vi "CellBild-v6.2.vi"() -> ()   [LabVIEW 2014]
uses:
  <vilib>/Utility/error.llb/DialogType.ctl
  <vilib>/DAQmx/create/channels.llb/DAQmx Create Channel (DI-Digital Input).vi
  <vilib>/DAQmx/create/channels.llb/DAQmx Create Channel (CO-Pulse Generation-Frequency).vi
  <vilib>/DAQmx/configure/timing.llb/DAQmx Timing (Implicit).vi
  <vilib>/DAQmx/create/channels.llb/DAQmx Create Channel (DO-Digital Output).vi
  <vilib>/DAQmx/write.llb/DAQmx Write (Digital Bool 1Line 1Point).vi
  <vilib>/DAQmx/write.llb/DAQmx Write (Analog DBL 1Chan 1Samp).vi
  <resource>/objmgr/daqmx.rc
panel:
  out "Pump running":bool
  out "dV":dbl format="%#.4g"
  out "Closing":bool
  out "In Done\nstate":bool
  in  "Tab Control":T1(tab)
  out "Shots to acquire":i32
  out "Shot no.":i32
  in  "Pump start":bool
  in  "Pulsed":bool
  in  "Populate":bool
  out "Full Power \nFrames":i32
  in  "Low Power\nFrames":i32
  in  "Link shutters":bool
  in  "FRAP":bool
  in  "EPI":bool
  in  "HALF DC":bool caption="Power"
  in  "manual laser control":bool
  in  "Continous ill":bool
  in  "Link rates":bool=TRUE
  in  "ALL OFF":bool
  in  "561 nm":bool
  in  "473 nm":bool
  in  "ALL LASERS":bool
  in  "Duty Cycle 1":dbl(knob)=0.47 caption="Duty Cycle\nlaser on state" min=0.001 max=0.999 step=0.05 scale=0.1..0.5
  in  "Frequency 1":dbl(knob)=100.0 caption="Laser\nrepetition rate" min=0.001 max=40000000.0 step=1.0 scale=1.0..500.0
  in  "stop":bool
  in  "Illuminated Frames":i32=10 min=0
  in  "Frame rate":dbl(knob)=200.0 min=0.01 max=40000000.0 step=1.0 scale=1.0..500.0
  in  "First frame\ndelay (ms)":dbl=15.0 min=50.0 format="%#_13g"
  in  "Finishing frames":i32=8
  out "Initial delay\n473 nm (ms)":dbl
  out "Trigger pulses":i32
  out "Initial frames":i32=2
  out "Laser pulses":i32
  out "Initial calculated\ndelay (frames)":dbl
  out "Laser delay (ms)":dbl
  out "Frames to acquire":i32
  in  "Duty Cycle \nDenominator":dbl=10.0 caption="Power\nDenominator" min=1.0 step=1.0
  out "AFLEX warning":bool caption="AFLEX conditions\nnormal"
  out "Duty Cycle 1\nfull DC":dbl(knob)=0.45 caption="Duty Cycle\nlaser on state" min=0.001 max=0.999 step=0.05 scale=0.1..0.5
  out "AFLEX warning 2":bool caption="AFLEX conditions\nnormal"
  out "Frame Rate display":dbl=2000.0 caption="Frame rate" min=0.0
  in  "Link shutters 2":bool caption="Link shutters"
  in  "FRAP 2":bool
  in  "EPI 2":bool
  out "initial delay\n473 nm (ms) 2":dbl caption="initial delay\n473 nm (ms)"
  in  "Link rates 2":bool=TRUE caption="Link rates"
  in  "Duty Cycle 2":dbl(knob)=0.47 caption="Duty Cycle\nlaser on state" min=0.001 max=0.999 step=0.05 scale=0.1..0.5
  in  "Frequency 2":dbl(knob)=100.0 caption="Laser\nrepetition rate" min=0.001 max=40000000.0 step=1.0 scale=1.0..500.0
  in  "Duty Cycle camera 2":dbl(knob)=0.001 caption="Duty Cycle\ncamera trigger" min=0.001 max=0.999 step=0.001 scale=0.001..0.999
  in  "Frame rate 2":dbl(knob)=200.0 caption="Frame rate" min=0.01 max=40000000.0 step=1.0 scale=1.0..500.0
  in  "AFLEX":bool
  in  "ALL OFF 2":bool
  in  "561 nm 2":bool
  in  "473 nm 2":bool
  in  "ALL LASERS 2":bool caption="ALL LASERS"
  in  "HALF DC 2":bool caption="Power"
  in  "Duty Cycle \nDenominator 2":dbl=2.0 caption="Power \nDenominator" min=1.0 step=1.0
  in  "Link shutters 3":bool
  in  "FRAP 3":bool
  in  "EPI 3":bool
  in  "FlowRateUnit":u32(ring) items=["ml/min", "ml/hr", "ul/min", "ul/hr"]
  in  "Flow rate":dbl=10.0
  in  "Syringe size":dbl(ring)=4.7 items=["1 ml"=4.7, "2.5 ml"=9.0, "3 ml"=8.59, "5 ml"=11.99, "10 ml"=14.48, "20 ml"=19.05, "30 ml"=21.59, "60 ml"=26.6]
  in  "Shots after pump start":i32=4
  in  "Deliverable volume (ml)":dbl min=0.0 step=0.1 format="%.4g"
  in  "Running time (s)":dbl=452.0
  in  "Shots before pump start":i32=1
  in  "Enable pump control":bool
  in  "Manual pump ctrl":bool
  in  "Pump initialisation":bool=TRUE
  in  "Pump ID":i32=3
  in  "Pump control port":refnum<visa-resource-name>="COM7"
  in  "Power control":bool=TRUE
  in  "idle state, shutdown":i32(ring)=10214 items=["High"=10192, "Low"=10214]
  in  "error in":errorcluster
  out "error out":errorcluster
  in  "561 nm counter":tag="Dev1/ctr4"
  in  "trigger ready source":tag="/Dev1/PFI3"
  in  "Camera trigger":tag="Dev1/ctr0"
  in  "473 nm counter":tag="Dev1/ctr2"
  in  "idle state, camera trig":i32(ring)=10214 items=["High"=10192, "Low"=10214]
  in  "idle state, lasers":i32(ring)=10214 items=["High"=10192, "Low"=10214]
  out "Loops":i32
  in  "Duty Cycle camera":dbl(knob)=0.0001 caption="Duty Cycle\ncamera trigger" min=0.0001 max=0.9999 step=5e-05 scale=0.0001..0.9999
  out "Duty Cycle 1\npreset":dbl(knob)=0.45 caption="Duty Cycle\nlaser on state" min=0.001 max=0.999 step=0.05 scale=0.1..0.999
  out "laser delay (s)":dbl
  in  "EPI ctrl":tag="Dev1/port0/line0"
  in  "FRAP ctrl":tag="Dev1/port0/line16"
  out "Duty Cycle 2\nmemory":dbl(knob)=0.45 caption="Duty Cycle\nlaser on state" min=0.001 max=0.999 step=0.05 scale=0.1..0.999
  in  "561nm line":tag="Dev2/ao0"
  in  "473nm line":tag="Dev2/ao1"
  in  "Level at max 473nm (0-5V)":dbl=4.200000000000002 caption="Level at max (0-5V)" min=0.0 max=5.0 step=0.05 format="%_4g"
  in  "473nm power level (0-1)":dbl=1.0 caption="Initial power level (0-1)" min=0.0 max=1.0 format="%_3g"
  in  "Level at max 561nm (0-5V)":dbl=4.225 caption="Level at max (0-5V)" min=0.0 max=5.0 step=0.05 format="%_4g"
  in  "561nm power level (0-1)":dbl=1.0 caption="Initial power level (0-1)" min=0.0 max=1.0 format="%_3g"
  out "561 task":refnum<k21>
  out "473 task":refnum<k21>
  out "HALF DC TEXT":string
  in  "delay\ncompensation":dbl format="%#_13g"
  out "Inited pump port":refnum<visa-resource-name>
  in  "vi path":path=path "C:/Biology/CellBild/Microfluidics/SPM100 control no loop v3.3.vi"
  out "modal pump reference":refnum<vi>
  # "Total number of frames to be\nilluminated (both channels)"
  # "Maximum number of frames\nthat can be acquired"
  # "Diagnostics"
  # "Laser Controls"
  # "Frame rate control"
  # "Shutter Controls"
  # "This tab generates a continous sequence of camera trigger pulses.\nLasers are synchronised with trigger pulse train but not synchronised with Micro-Manager acquisition start."
  # "Laser Controls"
  # "Shutter Controls"
  # "Frame rate control"
  # "Sequence settings"
  # "Pump settings"
  # "Enable pump sequence"
  # "Needed for \nmulti-shot \nacquisitions"
  # "IMPORTANT\nSafety for pump"
  # "Manual pump control"
  # "Total time \nfor all shots"
  # "Initial settings\nDAQ terminals"
  # "Pump control"
  # "Laser control counters"
  # "Laser power control settings"
  # "Camera trigger"
  # "Shutter control lines"
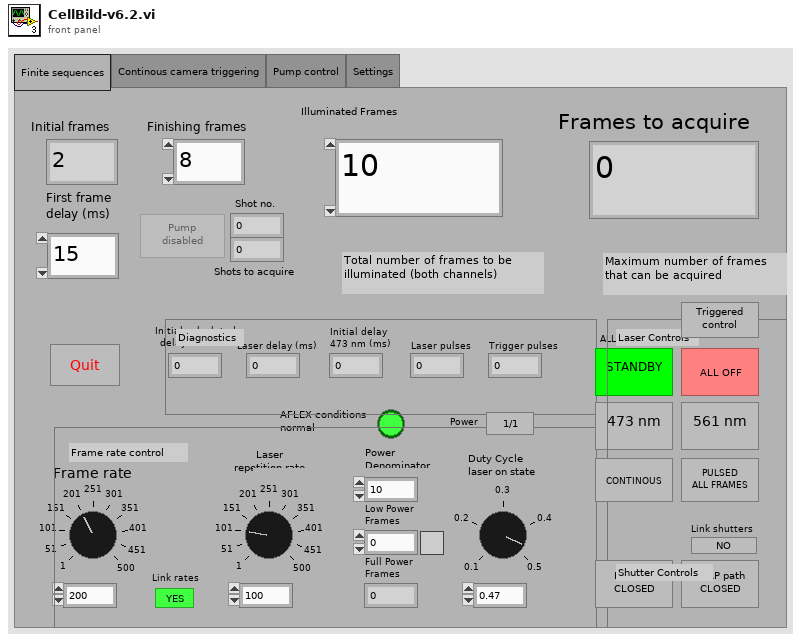
[diagram p1: front panel]
types:
  T1 = enum32{"Finite sequences", "Continous camera triggering", "Pump control", "Settings"}
  T2 = enum8{"Enabled", "Disabled", "Disabled and Grayed Out"}
  T3 = typedef "DialogType.ctl" = u16
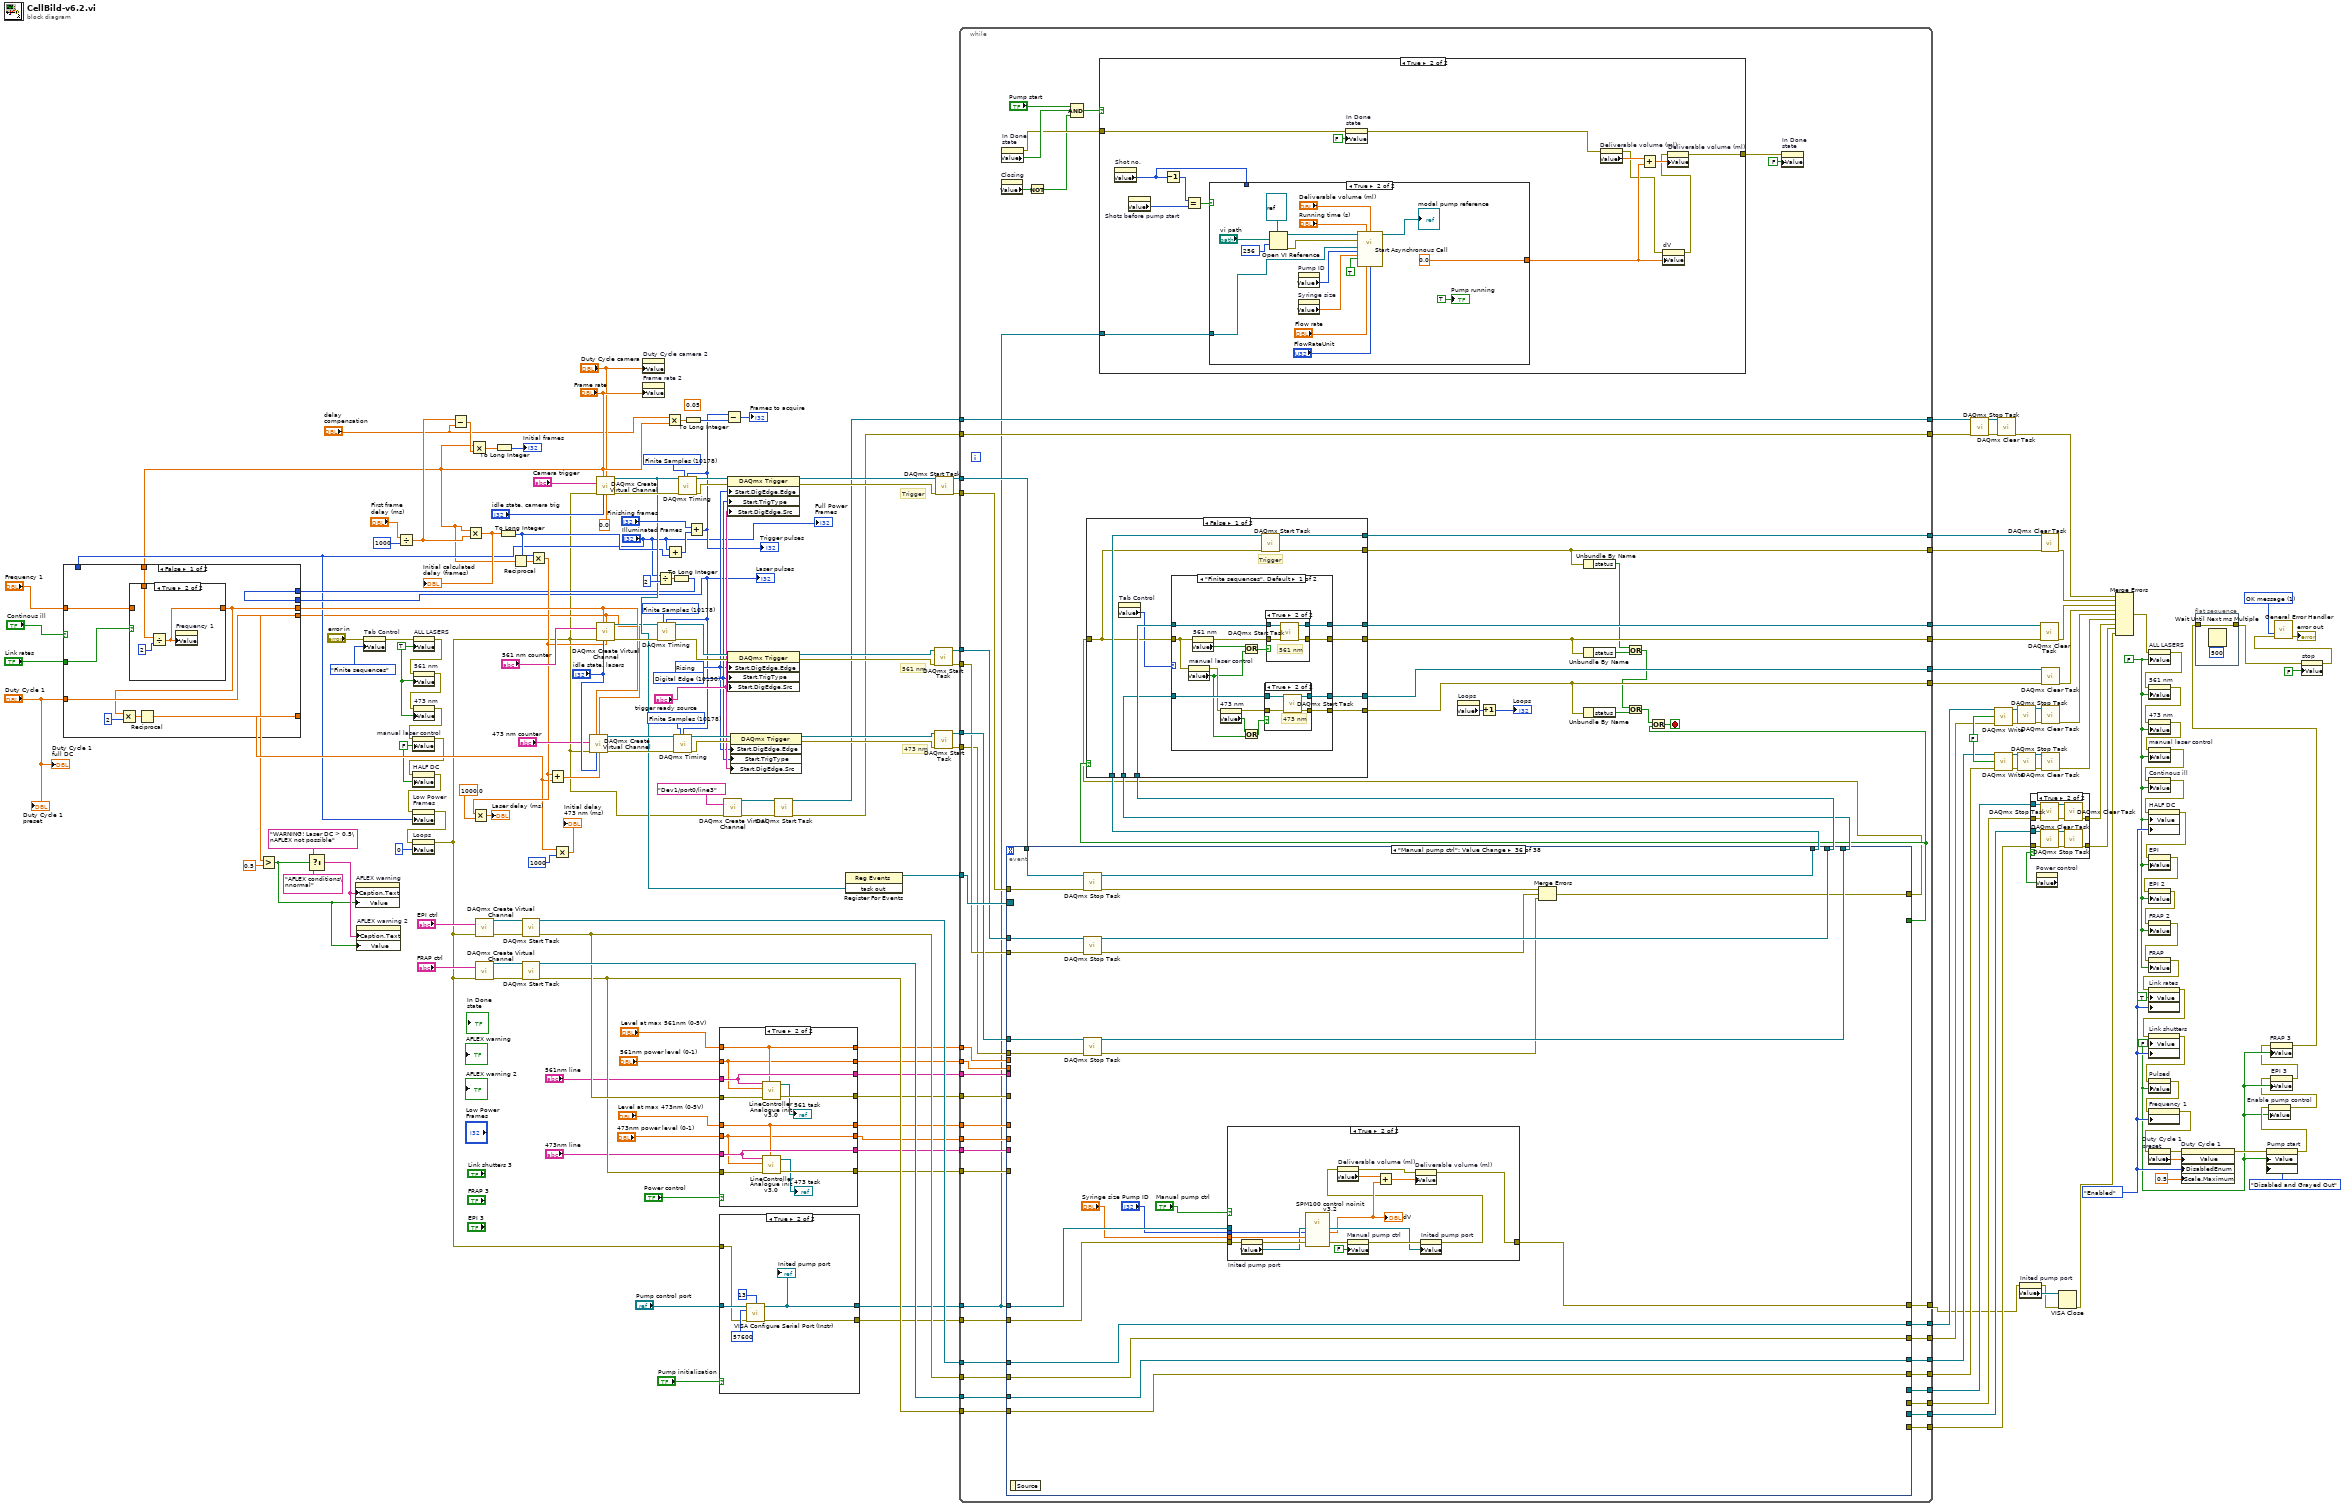
[diagram p0: block diagram]
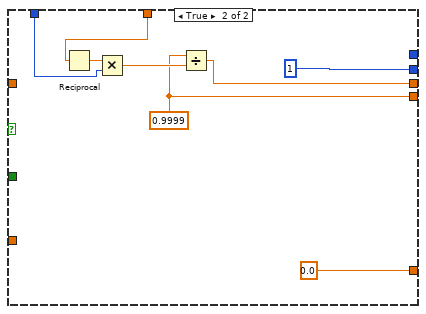
[diagram p6: hidden frame]
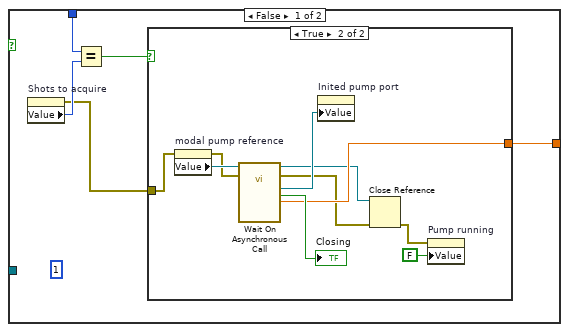
[diagram p8: hidden frame]
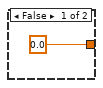
[diagram p9: hidden frame]
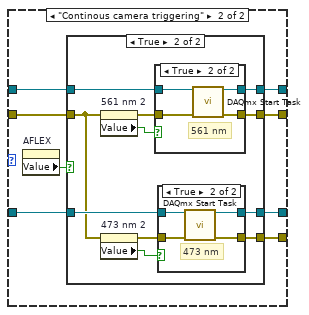
[diagram p12: hidden frame]
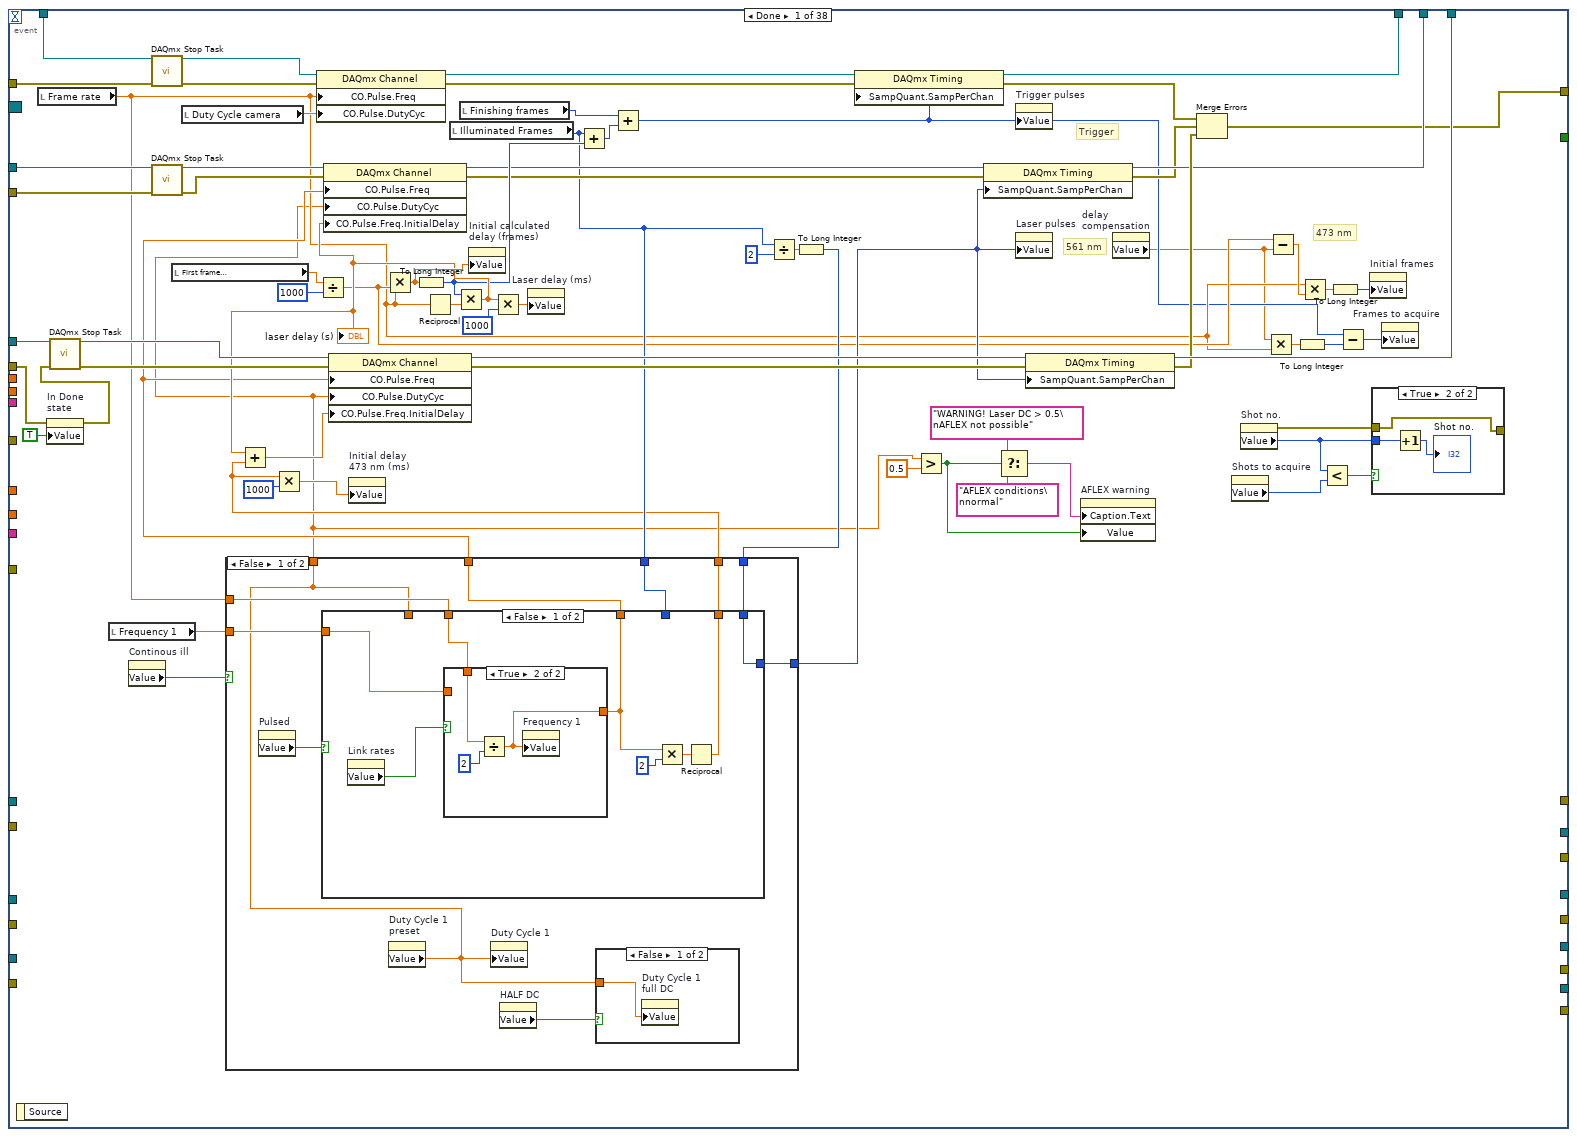
[diagram p17: hidden frame]
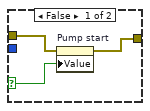
[diagram p18: hidden frame]
diagram:
  w74 = T2."Enabled" ("Disabled")
  (unwired) 0.05 ("x")
  w7 = FALSE ("Link shutters")
  w100 = FALSE ("data")
  w84 = FALSE ("manual laser control")
  w126 = TRUE ("Lasers on")
  w45 = FALSE ("Lasers on")
  w167 = 10178 items=["Finite Samples"=10178, "Continuous Samples"=10123, "Hardware Timed Single Point"=12522] ("sample mode")
  w185 = 10178 items=["Finite Samples"=10178, "Continuous Samples"=10123, "Hardware Timed Single Point"=12522] ("sample mode")
  w162 = 10150 items=["Analog Edge"=10099, "Digital Edge"=10150, "Digital Pattern"=10398, "Analog Window"=10103, "None"=10230] ("Start.TrigType")
  w161 = 10280 items=["Rising"=10280, "Falling"=10171] ("Start.DigEdge.Edge")
  w195 = T3 1 items=["no dialog", "OK message", "continue or stop message", "OK message + warnings", "continue/stop + warnings"] ("type of dialog (OK msg:1)")
  w197 = 10178 items=["Finite Samples"=10178, "Continuous Samples"=10123, "Hardware Timed Single Point"=12522] ("sample mode")
  # "Trigger"
  # "473 nm"
  # "561 nm"
  n1 = property on="Tab Control" class="TabCtl (strict)"(error in="error in", "Value"=T1."Finite sequences" ("Tab Control")) -> (error out=w125:errorcluster)  [unwired: 1 in, 1 out]
  n2 = Divide(x="First frame\ndelay (ms)", y=1000) -> (x/y=w92:dbl)
  n3 = property on="ALL LASERS" class="Bool (strict)"(error in=w125, "Value"=w126) -> (error out=w128:errorcluster)  [unwired: 1 in, 1 out]
  n4 = property on="561 nm" class="Bool (strict)"(error in=w128, "Value"=w126) -> (error out=w127:errorcluster)  [unwired: 1 in, 1 out]
  n5 = property on="473 nm" class="Bool (strict)"(error in=w127, "Value"=w126) -> (error out=w124:errorcluster)  [unwired: 1 in, 1 out]
  n6 = property on="manual laser control" class="Bool (strict)"(error in=w124, "Value"=w84) -> (error out=w83:errorcluster)  [unwired: 1 in, 1 out]
  n7 = property on="HALF DC" class="Bool (strict)"(error in=w83, "Value"=w84) -> (error out=w82:errorcluster)  [unwired: 1 in, 1 out]
  n8 = property on="Low Power\nFrames" class="DigNum (strict)"(error in=w82, "Value"="Illuminated Frames") -> (error out=w29:errorcluster)  [unwired: 1 in, 1 out]
  n9 = property on="Loops" class="DigNum (strict)"(error in=w29, "Value"=0 ("Frame")) -> (error out=w14:errorcluster)  [unwired: 1 in, 1 out]
  n10 = Subtract(x=w92, y="delay\ncompensation") -> (x-y=w91:dbl)
  n11 = Multiply(x="Frame rate", y=w92) -> (x*y=w156:dbl)
  "Initial calculated\ndelay (frames)" <- w156
  n12 = Multiply(x="Frame rate", y=w91) -> (x*y=w93:dbl)
  n13 = call-poly <vilib>:"DAQmx Create Virtual Channel.vi"("lines"="EPI ctrl", "error in"=w14) -> ("task out"=w114:refnum<k21>, "error out"=w113:errorcluster)  [unwired: 12 in]
  n14 = call-poly <vilib>:"DAQmx Create Virtual Channel.vi"("lines"="FRAP ctrl", "error in"=w14) -> ("task out"=w116:refnum<k21>, "error out"=w115:errorcluster)  [unwired: 12 in]
  n15 = To Long Integer(number=w93) -> (32bit integer=→"Initial frames":i32)
  n16 = To Long Integer(number=w156) -> (32bit integer=w95:i32)
  n17 = Reciprocal(x="Frame rate") -> (1/x=w153:dbl)
  n18 = call <vilib>:"DAQmx Start Task.vi"("task/channels in"=w114, "error in"=w113) -> ("task out"=w112:refnum<k21>, "error out"=w62:errorcluster)  [unwired: 12 in]
  n19 = call <vilib>:"DAQmx Start Task.vi"("task/channels in"=w116, "error in"=w115) -> ("task out"=w111:refnum<k21>, "error out"=w61:errorcluster)  [unwired: 12 in]
  n20 = Multiply(x=w95, y=w153) -> (x*y=w151:dbl)
  n21 = Multiply(x=w151, y=1000.0) -> (x*y=→"Laser delay (ms)":dbl)
  n22 = call-poly <vilib>:"DAQmx Create Virtual Channel.vi"("frequency"="Frame rate", "duty cycle"="Duty Cycle camera", "counter"="Camera trigger", "error in"=w14, "idle state"="idle state, camera trig", "initial delay"=0.0) -> ("task out"=w146:refnum<k21>, "error out"=w186:errorcluster)  [unwired: 8 in]
  n23 = property on="Duty Cycle camera 2" class="Knob (strict)"("Value"="Duty Cycle camera") -> ()  [unwired: 2 in, 2 out]
  n24 = property on="Frame rate 2" class="Knob (strict)"("Value"="Frame rate") -> ()  [unwired: 2 in, 2 out]
  n25 = Divide(x="Illuminated Frames", y=2) -> (x/y=w154:dbl)
  n26 = Multiply(x="delay\ncompensation", y="Frame rate") -> (x*y=w88:dbl)
  n27 = Add(x="Illuminated Frames", y=w95) -> (x+y=w157:i32)
  n28 = To Long Integer(number=w154) -> (32bit integer=w131:i32)
  n29 = case shown="False" "Continous ill" {
    tunnel: [w200 w214] -> w152
    tunnel: "Frame rate" -> [w207 w219]
    tunnel: "Frequency 1" -> [w206 _]
    tunnel: "Illuminated Frames" -> [_ w217]
    tunnel: w131 -> [w205 _]
    tunnel: [w205 1] -> w134
    tunnel: "Link rates" -> [w204 _]
    tunnel: [w203 w213] -> w65
    tunnel: "Duty Cycle 1" -> [w203 _]
    tunnel: [w199 0.0] -> w90
    frame False {
      n30 = case shown="True" w204 {
        tunnel: [w208 w209] -> w200
        tunnel: w207 -> [_ w211]
        tunnel: w206 -> [w208 _]
        frame False {
        }
        frame True {
          n31 = Divide(x=w211, y=2) -> (x/y=w209:dbl)
          n32 = property on="Frequency 1" class="Knob (strict)"("Value"=w209) -> ()  [unwired: 2 in, 2 out]
        }
      }
      n33 = Multiply(x=w200, y=2) -> (x*y=w201:dbl)
      n34 = Reciprocal(x=w201) -> (1/x=w199:dbl)
    }
    frame True {
      w213 = 0.9999 ("x")
      n35 = Reciprocal(x=w219) -> (1/x=w218:dbl)
      n36 = Multiply(x=w218, y=w217) -> (x*y=w215:dbl)
      n37 = Divide(x=w213, y=w215) -> (x/y=w214:dbl)
    }
  }
  "Laser pulses" <- w134
  n38 = Greater?(x=w65, y=0.5) -> (0:w63:bool)
  n39 = Select(t="WARNING! Laser DC > 0.5\nAFLEX not possible", s=w63, f="AFLEX conditions\nnormal") -> (s? t:f=w64:string)
  n40 = property on="AFLEX warning" class="Bool (strict)"("Caption.Text"=w64, "Value"=w63) -> ()  [unwired: 2 in, 2 out]
  n41 = property on="AFLEX warning 2" class="Bool (strict)"("Caption.Text"=w64, "Value"=w63) -> ()  [unwired: 2 in, 2 out]
  n42 = Add(x=w151, y=w90) -> (x+y=w166:dbl)
  n43 = Multiply(x=w90, y=1000) -> (x*y=→"Initial delay\n473 nm (ms)":dbl)
  n44 = call-poly <vilib>:"DAQmx Create Virtual Channel.vi"("frequency"=w152, "duty cycle"=w65, "counter"="473 nm counter", "error in"=w14, "idle state"="idle state, lasers", "initial delay"=w166) -> ("task out"=w169:refnum<k21>, "error out"=w168:errorcluster)  [unwired: 8 in]
  n45 = call-poly <vilib>:"DAQmx Create Virtual Channel.vi"("frequency"=w152, "duty cycle"=w65, "counter"="561 nm counter", "error in"=w14, "idle state"="idle state, lasers", "initial delay"=w151) -> ("task out"=w145:refnum<k21>, "error out"=w193:errorcluster)  [unwired: 8 in]
  n46 = call-poly <vilib>:"DAQmx Timing.vi"("task/channels in"=w145, "sample mode"=w197, "samples per channel"=w134, "error in"=w193) -> ("task out"=w192:refnum<k21>, "error out"=w191:errorcluster)  [unwired: 10 in]
  n47 = call-poly <vilib>:"DAQmx Timing.vi"("task/channels in"=w169, "sample mode"=w167, "samples per channel"=w134, "error in"=w168) -> ("task out"=w165:refnum<k21>, "error out"=w164:errorcluster)  [unwired: 10 in]
  n48 = To Long Integer(number=w88) -> (32bit integer=w87:i32)
  n49 = Add(x="Finishing frames", y=w157) -> (x+y=w86:i32)
  "Trigger pulses" <- w86
  n50 = call-poly <vilib>:"DAQmx Timing.vi"("task/channels in"=w146, "sample mode"=w185, "samples per channel"=w86, "error in"=w186) -> ("task out"=w184:refnum<k21>, "error out"=w183:errorcluster)  [unwired: 10 in]
  n51 = case shown="True" "Power control" {
    tunnel: w62 -> [w227 w239]
    tunnel: w61 -> [w226 w238]
    tunnel: [w227 w237] -> w60
    tunnel: [w226 w236] -> w56
    tunnel: [w221 w235] -> w44
    tunnel: [w220 w234] -> w43
    tunnel: "561nm line" -> [w221 w235]
    tunnel: "473nm line" -> [w220 w234]
    tunnel: "561nm power level (0-1)" -> [w225 w232]
    tunnel: "473nm power level (0-1)" -> [w224 w230]
    tunnel: [w225 w232] -> w33
    tunnel: [w224 w230] -> w35
    tunnel: "Level at max 561nm (0-5V)" -> [w223 w233]
    tunnel: "Level at max 473nm (0-5V)" -> [w222 w231]
    tunnel: [w223 w233] -> w34
    tunnel: [w222 w231] -> w36
    frame False {
    }
    frame True {
      n52 = call "LineController Analogue init v3.0.vi"("lines"=w235, "Power level (0-1)"=w232, "error in"=w239, "Level at max (0-5V)"=w233) -> ("task out"=→"561 task":refnum<k21>, "error out"=w237:errorcluster)  [unwired: 1 in, 1 out]
      n53 = call "LineController Analogue init v3.0.vi"("lines"=w234, "Power level (0-1)"=w230, "error in"=w238, "Level at max (0-5V)"=w231) -> ("task out"=→"473 task":refnum<k21>, "error out"=w236:errorcluster)  [unwired: 1 in, 1 out]
    }
  }
  n54 = case shown="True" "Pump initialisation" {
    tunnel: "Pump control port" -> [w241 w245]
    tunnel: w14 -> [w240 w244]
    tunnel: [w241 w243] -> w13
    tunnel: [w240 w242] -> w12
    frame False {
    }
    frame True {
      n55 = call <vilib>:"VISA Configure Serial Port (Instr).vi"("VISA resource name"=w245, "termination char\n(0xA = '\\n' = LF)"=u8 13 ("termination char\n(0xD = '\\r' = CR)"), "baud rate (9600)"=u32 57600 ("baud rate"), "error in (no error)"=w244) -> ("VISA resource name out"=w243:refnum<visa-resource-name>, "error out"=w242:errorcluster)  [unwired: 10 in]
      "Inited pump port" <- w243
    }
  }
  n56 = call-poly <vilib>:"DAQmx Create Virtual Channel.vi"("lines"=tag "Dev1/port0/line3", "error in"=w14) -> ("task out"=w27:refnum<k21>, "error out"=w26:errorcluster)  [unwired: 12 in]
  n57 = Subtract(x=w86, y=w87) -> (x-y=→"Frames to acquire":i32)
  n58 = property class="DAQmx Trigger"(reference=w184, error in=w183, "Start.DigEdge.Edge"=w161, "Start.TrigType"=w162, "Start.DigEdge.Src"="trigger ready source") -> (reference out=w181:refnum<k21>, error out=w180:errorcluster)
  n59 = property class="DAQmx Trigger"(reference=w192, error in=w191, "Start.DigEdge.Edge"=w161, "Start.TrigType"=w162, "Start.DigEdge.Src"="trigger ready source") -> (reference out=w72:refnum<k21>, error out=w71:errorcluster)
  n60 = property class="DAQmx Trigger"(reference=w165, error in=w164, "Start.DigEdge.Edge"=w161, "Start.TrigType"=w162, "Start.DigEdge.Src"="trigger ready source") -> (reference out=w70:refnum<k21>, error out=w69:errorcluster)
  n61 = call <vilib>:"DAQmx Start Task.vi"("task/channels in"=w27, "error in"=w26) -> ("task out"=w25:refnum<k21>, "error out"=w24:errorcluster)  [unwired: 12 in]
  n62 = register-events(w146) -> (reference out=w188:refnum<event-registration>)  [unwired: 2 in, 1 out]
  n63 = call <vilib>:"DAQmx Start Task.vi"("task/channels in"=w72, "error in"=w71) -> ("task out"=w196:refnum<k21>, "error out"=w190:errorcluster)  [unwired: 12 in]
  n64 = call <vilib>:"DAQmx Start Task.vi"("task/channels in"=w70, "error in"=w69) -> ("task out"=w160:refnum<k21>, "error out"=w159:errorcluster)  [unwired: 12 in]
  n65 = call <vilib>:"DAQmx Start Task.vi"("task/channels in"=w181, "error in"=w180) -> ("task out"=w179:refnum<k21>, "error out"=w178:errorcluster)  [unwired: 12 in]
  n66 = while {
    tunnel: w196 -> [w301]
    tunnel: w190 -> [w283]
    tunnel: [w305] -> w142
    tunnel: w188 -> [w304]
    tunnel: w179 -> [w302]
    tunnel: w178 -> [w298]
    tunnel: [w303] -> w176
    tunnel: [w292] -> w175
    tunnel: w160 -> [w296]
    tunnel: w159 -> [w282]
    tunnel: [w297] -> w139
    tunnel: [w291] -> w144
    tunnel: [w290] -> w140
    tunnel: w112 -> [w281]
    tunnel: w62 -> [w280]
    tunnel: w111 -> [w279]
    tunnel: w61 -> [w278]
    tunnel: [w277] -> w99
    tunnel: [w276] -> w98
    tunnel: [w275] -> w97
    tunnel: [w274] -> w57
    tunnel: w60 -> [w273]
    tunnel: [w272] -> w59
    tunnel: w56 -> [w271]
    tunnel: [w270] -> w53
    tunnel: [w269] -> w50
    tunnel: [w268] -> w51
    tunnel: w44 -> [w267]
    tunnel: w43 -> [w266]
    tunnel: w36 -> [w265]
    tunnel: w35 -> [w264]
    tunnel: w34 -> [w263]
    tunnel: w33 -> [w262]
    tunnel: w25 -> [w261]
    tunnel: w24 -> [w260]
    tunnel: [w261] -> w23
    tunnel: [w260] -> w22
    tunnel: w13 -> [w257]
    tunnel: w12 -> [w259]
    tunnel: [w258] -> w2
    stop <- w306 stop-if-true
    n67 = property on="Closing" class="Bool (strict)"() -> ("Value"=w251:bool)  [unwired: 2 in, 2 out]
    n68 = property on="In Done\nstate" class="Bool (strict)"() -> (error out=w252:errorcluster, "Value"=w253:bool)  [unwired: 2 in, 1 out]
    n69 = event shown="[35] \"Manual pump ctrl\": Value Change" {
      selector: w304 -> [_ _ _ _ _ _ _ _ _ _ _ _ _ _ _ _ _ _ _ _ _ _ _ _ _ _ _ _ _ _ _ _ _ _ _ _ _ _]
      dyn-events: _ -> [_ _ _ _ _ _ _ _ _ _ _ _ _ _ _ _ _ _ _ _ _ _ _ _ _ _ _ _ _ _ _ _ _ _ _ _ _ _]
      timeout: _ -> [_ _ _ _ _ _ _ _ _ _ _ _ _ _ _ _ _ _ _ _ _ _ _ _ _ _ _ _ _ _ _ _ _ _ _ _ _ _]
      tunnel: [w435 w568 w607 w857 w955 w1017 w1060 w1109 w1190 w1282 w1348 w1386 w1407 w1572 w1651 w1714 w1741 w1923 w2039 w2285 w2507 w2662 w2721 w2812 w2862 w2919 w3001 w3033 w3065 w3081 w3134 w3202 w3257 w3320 w3360 w3410 w3451 w3482] -> w256
      tunnel: [_ "stop" _ _ _ _ _ _ _ _ _ _ _ _ _ _ _ _ _ _ _ _ _ _ _ _ _ _ _ _ _ _ _ _ _ _ _ _] -> w284
      tunnel: w302 -> [w499 w573 w609 w859 w957 w1019 w1062 w1111 w1192 w1283 w1350 w1388 w1409 w1574 w1653 w1716 w1743 w1925 w2023 w2272 w2493 w2664 w2723 w2814 w2853 w2910 w2992 w3024 w3056 w3070 w3125 w3192 w3247 w3327 w3366 w3416 w3457 w3488]
      tunnel: w301 -> [w498 w567 w608 w858 w956 w1018 w1061 w1110 w1191 w1246 w1349 w1387 w1408 w1573 w1652 w1715 w1742 w1924 w2019 w2268 w2489 w2663 w2722 w2813 w2857 w2914 w2996 w3028 w3060 w3078 w3133 w3199 w3254 w3324 w3368 w3418 w3459 w3490]
      tunnel: [w466 w559 w594 w826 w923 w1002 w1044 w1099 w1157 w1253 w1332 w1369 w1395 w1540 w1619 w1693 w1735 w1903 w2032 w2279 w2500 w2631 w2688 w2779 w2866 w2904 w2974 w3008 w3040 w3083 w3119 w3205 w3243 w3323 w3363 w3413 w3454 w3485] -> w300
      tunnel: [w476 w574 w598 w835 w933 w1004 w1042 w1097 w1167 w1263 w1333 w1370 w1396 w1550 w1629 w1699 w1737 w1909 w2034 w2281 w2502 w2641 w2698 w2789 w2851 w2908 w2990 w3022 w3054 w3068 w3123 w3191 w3246 w3326 w3364 w3414 w3455 w3486] -> w299
      tunnel: w283 -> [w497 w572 w606 w856 w954 w1016 w1059 w1108 w1189 w1245 w1347 w1385 w1406 w1571 w1650 w1713 w1727 w1894 w2017 w2266 w2487 w2661 w2720 w2811 w2855 w2912 w2994 w3026 w3058 w3076 w3131 w3201 w3256 w3322 w3367 w3417 w3458 w3489]
      tunnel: w298 -> [w496 w575 w605 w855 w953 w1015 w1058 w1107 w1188 w1281 w1346 w1384 w1405 w1570 w1649 w1712 w1740 w1922 w2021 w2270 w2491 w2660 w2719 w2810 w2852 w2909 w2991 w3023 w3055 w3069 w3124 w3193 w3248 w3325 w3365 w3415 w3456 w3487]
      tunnel: w282 -> [w437 w570 w603 w853 w951 w1013 w1056 w1105 w1186 w1243 w1344 w1382 w1403 w1568 w1647 w1710 w1738 w1920 w2037 w2283 w2505 w2658 w2717 w2808 w2859 w2916 w2998 w3030 w3062 w3072 w3127 w3195 w3250 w3319 w3369 w3419 w3460 w3491]
      tunnel: w296 -> [w495 w571 w604 w854 w952 w1014 w1057 w1106 w1187 w1244 w1345 w1383 w1404 w1569 w1648 w1711 w1739 w1921 w2038 w2284 w2506 w2659 w2718 w2809 w2861 w2918 w3000 w3032 w3064 w3074 w3129 w3197 w3252 w3318 w3370 w3420 w3461 w3492]
      tunnel: [w470 w553 w596 w829 w927 w999 w1047 w1102 w1161 w1257 w1331 w1368 w1393 w1544 w1623 w1696 w1736 w1906 w2033 w2280 w2501 w2635 w2692 w2783 w2863 w2902 w2972 w3004 w3036 w3082 w3118 w3206 w3241 w3316 w3362 w3412 w3453 w3484] -> w295
      tunnel: w281 -> [_ w550 _ _ _ w1011 w1055 w1104 _ _ _ _ _ _ _ _ _ _ _ _ _ _ _ _ _ _ _ _ _ _ _ _ _ w3335 w3377 w3407 w3448 w3479]
      tunnel: w280 -> [_ w549 _ _ _ w998 w1054 w1103 _ _ _ _ _ _ _ _ _ _ _ _ _ _ _ _ _ _ _ _ _ _ _ _ _ w3314 w3376 w3404 w3445 w3476]
      tunnel: w279 -> [_ w548 _ _ _ w1010 w1053 w1096 _ _ _ _ _ _ _ _ _ _ _ _ _ _ _ _ _ _ _ _ _ _ _ _ _ w3334 w3375 w3406 w3447 w3478]
      tunnel: w278 -> [_ w547 _ _ _ w1009 w1041 w1095 _ _ _ _ _ _ _ _ _ _ _ _ _ _ _ _ _ _ _ _ _ _ _ _ _ w3333 w3357 w3405 w3446 w3477]
      tunnel: [_ w550 _ _ _ w1008 w1051 w1104 _ _ _ _ _ _ _ _ _ _ _ _ _ _ _ _ _ _ _ _ _ _ _ _ _ w3332 w3374 w3407 w3448 w3479] -> w277
      tunnel: [_ w549 _ _ _ w1007 w1050 w1103 _ _ _ _ _ _ _ _ _ _ _ _ _ _ _ _ _ _ _ _ _ _ _ _ _ w3331 w3373 w3404 w3445 w3476] -> w276
      tunnel: [_ w548 _ _ _ w1006 w1049 w1096 _ _ _ _ _ _ _ _ _ _ _ _ _ _ _ _ _ _ _ _ _ _ _ _ _ w3330 w3372 w3406 w3447 w3478] -> w275
      tunnel: [_ w547 _ _ _ w1005 w1048 w1095 _ _ _ _ _ _ _ _ _ _ _ _ _ _ _ _ _ _ _ _ _ _ _ _ _ w3329 w3371 w3405 w3446 w3477] -> w274
      tunnel: w273 -> [_ w545 _ _ _ _ _ w1093 _ _ _ _ _ _ _ _ w1726 w1888 w2015 w2263 _ _ _ _ _ _ _ _ _ _ _ _ _ _ _ _ _ _]
      tunnel: [_ w542 _ _ _ _ _ w1085 _ _ _ _ _ _ _ _ w1717 w1887 w2013 w2258 _ _ _ _ _ _ _ _ _ _ _ _ _ _ _ _ _ _] -> w272
      tunnel: w271 -> [_ w546 _ _ _ _ _ w1092 _ _ _ _ _ _ _ _ w1725 w1889 w2012 w2262 _ _ _ _ _ _ _ _ _ _ _ _ _ _ _ _ _ _]
      tunnel: [_ w541 _ _ _ _ _ w1083 _ _ _ _ _ _ _ _ w1720 w1885 w2010 w2257 _ _ _ _ _ _ _ _ _ _ _ _ _ _ _ _ _ _] -> w270
      tunnel: [_ w546 _ _ _ _ _ w1082 _ _ _ _ _ _ _ _ w1719 w1884 w2006 w2254 _ _ _ _ _ _ _ _ _ _ _ _ _ _ _ _ _ _] -> w269
      tunnel: [_ w545 _ _ _ _ _ w1084 _ _ _ _ _ _ _ _ w1718 w1886 w2007 w2253 _ _ _ _ _ _ _ _ _ _ _ _ _ _ _ _ _ _] -> w268
      tunnel: w267 -> [_ _ _ _ _ _ _ w1091 _ _ _ _ _ _ _ _ _ _ _ _ _ _ _ _ _ _ _ _ _ _ _ _ _ _ _ _ _ _]
      tunnel: w266 -> [_ _ _ _ _ _ _ w1090 _ _ _ _ _ _ _ _ _ _ _ _ _ _ _ _ _ _ _ _ _ _ _ _ _ _ _ _ _ _]
      tunnel: w265 -> [_ _ _ _ _ _ _ w1089 _ _ _ _ _ _ _ _ _ _ _ _ _ _ _ _ _ _ _ _ _ _ _ _ _ _ _ _ _ _]
      tunnel: w264 -> [_ _ _ _ _ _ _ w1088 _ _ _ _ _ _ _ _ _ _ _ _ _ _ _ _ _ _ _ _ _ _ _ _ _ _ _ _ _ _]
      tunnel: w263 -> [_ _ _ _ _ _ _ w1087 _ _ _ _ _ _ _ _ _ _ _ _ _ _ _ _ _ _ _ _ _ _ _ _ _ _ _ _ _ _]
      tunnel: w262 -> [_ _ _ _ _ _ _ w1086 _ _ _ _ _ _ _ _ _ _ _ _ _ _ _ _ _ _ _ _ _ _ _ _ _ _ _ _ _ _]
      tunnel: w257 -> [_ _ w589 _ _ _ _ _ _ _ _ _ _ _ _ _ _ _ _ _ _ _ _ _ _ _ _ _ _ _ _ _ _ _ _ w3402 _ _]
      tunnel: w259 -> [_ _ w588 _ _ _ _ _ _ _ _ _ _ _ _ _ _ _ _ _ _ _ _ _ _ _ _ _ _ _ _ _ _ _ _ w3401 w3443 w3471]
      tunnel: [_ _ w587 _ _ _ _ _ _ _ _ _ _ _ _ _ _ _ _ _ _ _ _ _ _ _ _ _ _ _ _ _ _ _ _ w3400 w3438 w3473] -> w258
      event Done {
        # "Trigger"
        # "473 nm"
        # "561 nm"
        n70 = event-data() -> ()  [unwired: 1 in, 1 out]
        n71 = local read "Frame rate"() -> (w446:dbl)
        n72 = property on="In Done\nstate" class="Bool (strict)"(error in=w437, "Value"=TRUE ("In Done\nstate")) -> (error out=w430:errorcluster)  [unwired: 1 in, 1 out]
        n73 = call <vilib>:"DAQmx Stop Task.vi"("task/channels in"=w495, "error in"=w430) -> ("task out"=w483:refnum<k21>, "error out"=w482:errorcluster)  [unwired: 12 in]
        n74 = local read "Frequency 1"() -> (w458:dbl)
        n75 = property on="Continous ill" class="Bool (strict)"() -> ("Value"=w460:bool)  [unwired: 2 in, 2 out]
        n76 = call <vilib>:"DAQmx Stop Task.vi"("task/channels in"=w499, "error in"=w496) -> ("task out"=w489:refnum<k21>, "error out"=w488:errorcluster)  [unwired: 12 in]
        n77 = call <vilib>:"DAQmx Stop Task.vi"("task/channels in"=w498, "error in"=w497) -> ("task out"=w486:refnum<k21>, "error out"=w485:errorcluster)  [unwired: 12 in]
        n78 = local read "First frame\ndelay (ms)"() -> (w491:dbl)
        n79 = local read "Duty Cycle camera"() -> (w487:dbl)
        n80 = property class="DAQmx Channel"(reference=w489, error in=w488, "CO.Pulse.Freq"=w446, "CO.Pulse.DutyCyc"=w487) -> (reference out=w477:refnum<k21>, error out=w475:errorcluster)
        n81 = Divide(x=w491, y=1000) -> (x/y=w451:dbl)
        n82 = Multiply(x=w446, y=w451) -> (x*y=w493:dbl)
        n83 = To Long Integer(number=w493) -> (32bit integer=w472:i32)
        n84 = Reciprocal(x=w446) -> (1/x=w492:dbl)
        n85 = local read "Illuminated Frames"() -> (w459:i32)
        n86 = Multiply(x=w472, y=w492) -> (x*y=w478:dbl)
        "laser delay (s)" <- w478
        n87 = local read "Finishing frames"() -> (w473:i32)
        n88 = property on="Initial calculated\ndelay (frames)" class="DigNum (strict)"("Value"=w493) -> ()  [unwired: 2 in, 2 out]
        n89 = Multiply(x=w478, y=1000) -> (x*y=w484:dbl)
        n90 = property on="Laser delay (ms)" class="DigNum (strict)"("Value"=w484) -> ()  [unwired: 2 in, 2 out]
        n91 = Add(x=w459, y=w472) -> (x+y=w461:i32)
        n92 = Add(x=w473, y=w461) -> (x+y=w445:i32)
        n93 = Divide(x=w459, y=2) -> (x/y=w462:dbl)
        n94 = To Long Integer(number=w462) -> (32bit integer=w456:i32)
        n95 = case shown="False" w460 {
          tunnel: [w512 w533] -> w457
          tunnel: w446 -> [w514 w534]
          tunnel: w458 -> [w515 _]
          tunnel: w459 -> [w508 w538]
          tunnel: [w509 1] -> w455
          tunnel: [w506 w535] -> w439
          tunnel: w456 -> [w511 _]
          tunnel: [w513 0.0] -> w450
          frame False {
            n96 = property on="Pulsed" class="Bool (strict)"() -> ("Value"=w510:bool)  [unwired: 2 in, 2 out]
            n97 = property on="Duty Cycle 1\npreset" class="Knob (strict)"() -> ("Value"=w506:dbl)  [unwired: 2 in, 2 out]
            n98 = case shown="False" w510 {
              tunnel: w515 -> [w524 _]
              tunnel: w514 -> [w523 w530]
              tunnel: w506 -> [_ _]
              tunnel: [w519 0.0] -> w513
              tunnel: [w518 w530] -> w512
              tunnel: w511 -> [w517 _]
              tunnel: [w517 w529] -> w509
              tunnel: w508 -> [_ w529]
              frame False {
                n99 = property on="Link rates" class="Bool (strict)"() -> ("Value"=w522:bool)  [unwired: 2 in, 2 out]
                n100 = case shown="True" w522 {
                  tunnel: [w525 w526] -> w518
                  tunnel: w523 -> [_ w528]
                  tunnel: w524 -> [w525 _]
                  frame False {
                  }
                  frame True {
                    n101 = Divide(x=w528, y=2) -> (x/y=w526:dbl)
                    n102 = property on="Frequency 1" class="Knob (strict)"("Value"=w526) -> ()  [unwired: 2 in, 2 out]
                  }
                }
                n103 = Multiply(x=w518, y=2) -> (x*y=w521:dbl)
                n104 = Reciprocal(x=w521) -> (1/x=w519:dbl)
              }
              frame True {
              }
            }
            n105 = property on="Duty Cycle 1" class="Knob (strict)"("Value"=w506) -> ()  [unwired: 2 in, 2 out]
            n106 = property on="HALF DC" class="Bool (strict)"() -> ("Value"=w507:bool)  [unwired: 2 in, 2 out]
            n107 = case shown="False" w507 {
              tunnel: w506 -> [w516 _]
              frame False {
                n108 = property on="Duty Cycle 1\nfull DC" class="Knob (strict)"("Value"=w516) -> ()  [unwired: 2 in, 2 out]
              }
              frame True {
              }
            }
          }
          frame True {
            w535 = 0.9999 ("x")
            n109 = Reciprocal(x=w534) -> (1/x=w539:dbl)
            n110 = Multiply(x=w539, y=w538) -> (x*y=w536:dbl)
            n111 = property on="Duty Cycle 1" class="Knob (strict)"("Value"=w535) -> ()  [unwired: 2 in, 2 out]
            n112 = Divide(x=w535, y=w536) -> (x/y=w533:dbl)
            n113 = property on="Frequency 1" class="Knob (strict)"("Value"=w533) -> ()  [unwired: 2 in, 2 out]
          }
        }
        n114 = Add(x=w478, y=w450) -> (x+y=w479:dbl)
        n115 = Multiply(x=w450, y=1000) -> (x*y=w480:dbl)
        n116 = property class="DAQmx Channel"(reference=w486, error in=w485, "CO.Pulse.Freq"=w457, "CO.Pulse.DutyCyc"=w439, "CO.Pulse.Freq.InitialDelay"=w478) -> (reference out=w467:refnum<k21>, error out=w465:errorcluster)
        n117 = property class="DAQmx Channel"(reference=w483, error in=w482, "CO.Pulse.Freq"=w457, "CO.Pulse.DutyCyc"=w439, "CO.Pulse.Freq.InitialDelay"=w479) -> (reference out=w471:refnum<k21>, error out=w469:errorcluster)
        n118 = property on="Initial delay\n473 nm (ms)" class="DigNum (strict)"("Value"=w480) -> ()  [unwired: 2 in, 2 out]
        n119 = property class="DAQmx Timing"(reference=w477, error in=w475, "SampQuant.SampPerChan"=w445) -> (reference out=w476:refnum<k21>, error out=w474:errorcluster)
        n120 = Greater?(x=w439, y=0.5) -> (0:w440:bool)
        n121 = property class="DAQmx Timing"(reference=w467, error in=w465, "SampQuant.SampPerChan"=w455) -> (reference out=w466:refnum<k21>, error out=w464:errorcluster)
        n122 = Select(t="WARNING! Laser DC > 0.5\nAFLEX not possible", s=w440, f="AFLEX conditions\nnormal") -> (s? t:f=w441:string)
        n123 = property on="Trigger pulses" class="DigNum (strict)"("Value"=w445) -> ()  [unwired: 2 in, 2 out]
        n124 = property on="Laser pulses" class="DigNum (strict)"("Value"=w455) -> ()  [unwired: 2 in, 2 out]
        n125 = property class="DAQmx Timing"(reference=w471, error in=w469, "SampQuant.SampPerChan"=w455) -> (reference out=w470:refnum<k21>, error out=w468:errorcluster)
        n126 = property on="AFLEX warning" class="Bool (strict)"("Caption.Text"=w441, "Value"=w440) -> ()  [unwired: 2 in, 2 out]
        n127 = property on="delay\ncompensation" class="DigNum (strict)"() -> ("Value"=w438:dbl)  [unwired: 2 in, 2 out]
        n128 = Merge Errors(w474, w464, w468) -> (w435:errorcluster)
        n129 = property on="Shots to acquire" class="DigNum (strict)"() -> ("Value"=w433:i32)  [unwired: 2 in, 2 out]
        n130 = property on="Shot no." class="DigNum (strict)"() -> (error out=w432:errorcluster, "Value"=w431:i32)  [unwired: 2 in, 1 out]
        n131 = Multiply(x=w438, y=w446) -> (x*y=w447:dbl)
        n132 = Subtract(x=w451, y=w438) -> (x-y=w453:dbl)
        n133 = To Long Integer(number=w447) -> (32bit integer=w448:i32)
        n134 = Multiply(x=w446, y=w453) -> (x*y=w454:dbl)
        n135 = Less?(x=w431, y=w433) -> (x < y?=w434:bool)
        n136 = To Long Integer(number=w454) -> (32bit integer=w452:i32)
        n137 = Subtract(x=w445, y=w448) -> (x-y=w449:i32)
        n138 = property on="Initial frames" class="DigNum (strict)"("Value"=w452) -> ()  [unwired: 2 in, 2 out]
        n139 = case shown="True" w434 {
          selector: w434 -> [w502 _]
          tunnel: w431 -> [_ w505]
          tunnel: w432 -> [w501 w503]
          tunnel: [w500 w503] -> _
          frame False {
            n140 = property on="Pump start" class="Bool (strict)"(error in=w501, "Value"=w502) -> (error out=w500:errorcluster)  [unwired: 1 in, 1 out]
          }
          frame True {
            n141 = Increment(x=w505) -> (x+1=→"Shot no.":i32)
          }
        }
        n142 = property on="Frames to acquire" class="DigNum (strict)"("Value"=w449) -> ()  [unwired: 2 in, 2 out]
      }
      event "stop": Value Change {
        # "display iterations\nbefore exiting"
        # "Trigger"
        # "473 nm"
        # "561 nm"
        n143 = event-data() -> ()  [unwired: 1 in, 1 out]
        n144 = call <vilib>:"DAQmx Stop Task.vi"("task/channels in"=w571, "error in"=w570) -> ("task out"=w558:refnum<k21>, "error out"=w557:errorcluster)  [unwired: 12 in]
        n145 = call <vilib>:"DAQmx Stop Task.vi"("task/channels in"=w573, "error in"=w575) -> ("task out"=w574:refnum<k21>, "error out"=w569:errorcluster)  [unwired: 12 in]
        n146 = call <vilib>:"DAQmx Stop Task.vi"("task/channels in"=w567, "error in"=w572) -> ("task out"=w566:refnum<k21>, "error out"=w565:errorcluster)  [unwired: 12 in]
        n147 = property class="DAQmx Channel"(reference=w566, error in=w565, "CO.Pulse.IdleState"="idle state, shutdown") -> (reference out=w564:refnum<k21>, error out=w563:errorcluster)
        n148 = property class="DAQmx Channel"(reference=w558, error in=w557, "CO.Pulse.IdleState"="idle state, shutdown") -> (reference out=w554:refnum<k21>, error out=w552:errorcluster)
        n149 = call <vilib>:"DAQmx Start Task.vi"("task/channels in"=w564, "error in"=w563) -> ("task out"=w560:refnum<k21>, "error out"=w562:errorcluster)  [unwired: 12 in]
        n150 = call <vilib>:"DAQmx Start Task.vi"("task/channels in"=w554, "error in"=w552) -> ("task out"=w555:refnum<k21>, "error out"=w556:errorcluster)  [unwired: 12 in]
        n151 = call <vilib>:"DAQmx Stop Task.vi"("task/channels in"=w560, "error in"=w562) -> ("task out"=w559:refnum<k21>, "error out"=w561:errorcluster)  [unwired: 12 in]
        n152 = call <vilib>:"DAQmx Stop Task.vi"("task/channels in"=w555, "error in"=w556) -> ("task out"=w553:refnum<k21>, "error out"=w544:errorcluster)  [unwired: 12 in]
        n153 = case shown="True" FALSE {
          tunnel: [w577 w578] -> w540
          tunnel: w544 -> [w577 w581]
          frame False {
          }
          frame True {
            n154 = property on="Loops" class="DigNum (strict)"(error in=w581) -> (error out=w579:errorcluster, "Value"=w586:i32)  [unwired: 1 in, 1 out]
            n155 = property on="Loops" class="DigNum (strict)"(error in=w579, "Value"=0 ("Frame")) -> (error out=w578:errorcluster)  [unwired: 1 in, 1 out]
            n156 = Number To Decimal String(number=w586) -> (decimal integer string=w583:string)  [unwired: 1 in]
            n157 = Concatenate Strings("The application has run " ("string"), w583, " iterations" ("string")) -> (w582:string)
            n158 = One Button Dialog(message=w582) -> ()  [unwired: 1 in, 1 out]
          }
        }
        n159 = Merge Errors(w569, w561, w540) -> (w568:errorcluster)
        n160 = property on="473 task" class="DAQmxName (strict)"() -> ("Value"=w541:refnum<k21>)  [unwired: 2 in, 2 out]
        n161 = property on="561 task" class="DAQmxName (strict)"() -> ("Value"=w542:refnum<k21>)  [unwired: 2 in, 2 out]
      }
      event "Tab Control": Value Change {
        n162 = event-data() -> ()  [unwired: 1 in, 1 out]
        n163 = call <vilib>:"DAQmx Stop Task.vi"("task/channels in"=w609, "error in"=w605) -> ("task out"=w602:refnum<k21>, "error out"=w591:errorcluster)  [unwired: 12 in]
        n164 = call <vilib>:"DAQmx Stop Task.vi"("task/channels in"=w604, "error in"=w603) -> ("task out"=w600:refnum<k21>, "error out"=w599:errorcluster)  [unwired: 12 in]
        n165 = call <vilib>:"DAQmx Stop Task.vi"("task/channels in"=w608, "error in"=w606) -> ("task out"=w601:refnum<k21>, "error out"=w592:errorcluster)  [unwired: 12 in]
        n166 = case shown="\"Pump control\"" "Tab Control" {
          tunnel: w602 -> [w711 w772 w800]
          tunnel: w591 -> [w710 w759 w799]
          tunnel: w601 -> [w708 w749 w798]
          tunnel: w592 -> [w707 w768 w797]
          tunnel: w600 -> [w705 w740 w796]
          tunnel: w599 -> [w682 w741 w795]
          tunnel: [w676 w765 w800] -> w598
          tunnel: [w674 w763 w799] -> w597
          tunnel: [w691 w740 w796] -> w596
          tunnel: [w689 w742 w795] -> w595
          tunnel: [w681 w749 w798] -> w594
          tunnel: [w680 w768 w797] -> w593
          tunnel: w589 -> [_ _ _]
          tunnel: w588 -> [w614 w723 w794]
          tunnel: [w614 w723 w794] -> w587
          frame "Finite sequences", Default {
            w631 = 10178 items=["Finite Samples"=10178, "Continuous Samples"=10123, "Hardware Timed Single Point"=12522] ("SampQuant.SampMode")
            w617 = T2."Enabled" ("Disabled")
            (unwired) 0.05 ("x")
            (unwired) 0.05 ("y")
            w623 = FALSE ("AFLEX")
            w673 = 10214 items=["High"=10192, "Low"=10214] ("CO.Pulse.IdleState")
            w678 = 10150 items=["Analog Edge"=10099, "Digital Edge"=10150, "Digital Pattern"=10398, "Analog Window"=10103, "None"=10230] ("Start.TrigType")
            w679 = 10178 items=["Finite Samples"=10178, "Continuous Samples"=10123, "Hardware Timed Single Point"=12522] ("SampQuant.SampMode")
            # "Trigger"
            # "473 nm"
            # "561 nm"
            n167 = property on="Duty Cycle \nDenominator 2" class="DigNum (strict)"(error in=w614, "DisabledEnum"=T2."Disabled and Grayed Out" ("Disabled")) -> (error out=w628:errorcluster, "Value"=w626:dbl)  [unwired: 1 in, 1 out]
            n168 = property on="Duty Cycle 2" class="Knob (strict)"() -> ("Value"=w633:dbl)  [unwired: 2 in, 2 out]
            n169 = local read "First frame\ndelay (ms)"() -> (w713:dbl)
            n170 = local read "Duty Cycle camera"() -> (w709:dbl)
            n171 = local read "Frequency 1"() -> (w697:dbl)
            n172 = Multiply(x=w697, y=2) -> (x*y=w703:dbl)
            n173 = Reciprocal(x=w703) -> (1/x=w701:dbl)
            n174 = property on="Duty Cycle \nDenominator" class="DigNum (strict)"(error in=w628, "Value"=w626, "DisabledEnum"=w617) -> (error out=w627:errorcluster)  [unwired: 1 in, 1 out]
            n175 = Greater?(x=w633, y=0.5) -> (0:w634:bool)
            n176 = local read "Frame rate"() -> (w646:dbl)
            n177 = property on="Duty Cycle 1\npreset" class="Knob (strict)"("Value"=w633) -> ()  [unwired: 2 in, 2 out]
            n178 = Multiply(x=w701, y=1000) -> (x*y=w700:dbl)
            n179 = property on="Initial delay\n473 nm (ms)" class="DigNum (strict)"("Value"=w700) -> ()  [unwired: 2 in, 2 out]
            n180 = Select(t="WARNING! Laser DC > 0.5\nAFLEX not possible", s=w634, f="AFLEX conditions\nnormal") -> (s? t:f=w635:string)
            n181 = property on="manual laser control" class="Bool (strict)"(error in=w627, "Value"=w623) -> (error out=w662:errorcluster)  [unwired: 1 in, 1 out]
            n182 = property class="DAQmx Channel"(reference=w711, error in=w710, "CO.Pulse.Freq"=w646, "CO.Pulse.DutyCyc"=w709) -> (reference out=w696:refnum<k21>, error out=w695:errorcluster)
            n183 = Divide(x=w713, y=1000) -> (x/y=w650:dbl)
            n184 = property on="AFLEX warning" class="Bool (strict)"("Caption.Text"=w635, "Value"=w634) -> ()  [unwired: 2 in, 2 out]
            n185 = Multiply(x=w646, y=w650) -> (x*y=w715:dbl)
            n186 = property on="AFLEX" class="Bool (strict)"(error in=w662, "Value"=w623) -> (error out=w643:errorcluster)  [unwired: 1 in, 1 out]
            n187 = property on="delay\ncompensation" class="DigNum (strict)"() -> ("Value"=w615:dbl)  [unwired: 2 in, 2 out]
            n188 = To Long Integer(number=w715) -> (32bit integer=w693:i32)
            n189 = Reciprocal(x=w646) -> (1/x=w714:dbl)
            n190 = local read "Illuminated Frames"() -> (w683:i32)
            n191 = local read "Finishing frames"() -> (w694:i32)
            n192 = Multiply(x=w693, y=w714) -> (x*y=w698:dbl)
            n193 = Add(x=w698, y=w701) -> (x+y=w699:dbl)
            n194 = property class="DAQmx Channel"(reference=w708, error in=w707, "CO.Pulse.Freq"=w697, "CO.Pulse.DutyCyc"=w633, "CO.Pulse.Freq.InitialDelay"=w698, "CO.Pulse.IdleState"=w673) -> (reference out=w688:refnum<k21>, error out=w687:errorcluster)
            n195 = property class="DAQmx Channel"(reference=w705, error in=w682, "CO.Pulse.Freq"=w697, "CO.Pulse.DutyCyc"=w633, "CO.Pulse.Freq.InitialDelay"=w699, "CO.Pulse.IdleState"=w673) -> (reference out=w692:refnum<k21>, error out=w690:errorcluster)
            n196 = property on="Continous ill" class="Bool (strict)"(error in=w643, "Value"=w623) -> (error out=w642:errorcluster)  [unwired: 1 in, 1 out]
            n197 = property on="Initial calculated\ndelay (frames)" class="DigNum (strict)"("Value"=w715) -> ()  [unwired: 2 in, 2 out]
            n198 = Multiply(x=w698, y=1000) -> (x*y=w706:dbl)
            n199 = property on="Laser delay (ms)" class="DigNum (strict)"("Value"=w706) -> ()  [unwired: 2 in, 2 out]
            n200 = property on="Pulsed" class="Bool (strict)"(error in=w642, "Value"=w623) -> (error out=w644:errorcluster)  [unwired: 1 in, 1 out]
            n201 = Add(x=w683, y=w693) -> (x+y=w684:i32)
            n202 = property on="ALL LASERS 2" class="Bool (strict)"(error in=w644) -> (error out=w671:errorcluster, "Value"=w672:bool)  [unwired: 1 in, 1 out]
            n203 = Multiply(x=w615, y=w646) -> (x*y=w647:dbl)
            n204 = Subtract(x=w650, y=w615) -> (x-y=w652:dbl)
            n205 = Divide(x=w683, y=2) -> (x/y=w685:dbl)
            n206 = Add(x=w694, y=w684) -> (x+y=w645:i32)
            n207 = property class="DAQmx Timing"(reference=w696, error in=w695, "SampQuant.SampMode"=w679, "SampQuant.SampPerChan"=w645) -> (reference out=w677:refnum<k21>, error out=w675:errorcluster)
            n208 = To Long Integer(number=w647) -> (32bit integer=w648:i32)
            n209 = property on="ALL LASERS" class="Bool (strict)"(error in=w671, "Value"=w672) -> (error out=w668:errorcluster)  [unwired: 1 in, 1 out]
            n210 = Subtract(x=w645, y=w648) -> (x-y=w649:i32)
            n211 = Multiply(x=w646, y=w652) -> (x*y=w653:dbl)
            n212 = property on="Frames to acquire" class="DigNum (strict)"("Value"=w649) -> ()  [unwired: 2 in, 2 out]
            n213 = To Long Integer(number=w653) -> (32bit integer=w651:i32)
            n214 = To Long Integer(number=w685) -> (32bit integer=w632:i32)
            n215 = property on="473 nm 2" class="Bool (strict)"(error in=w668) -> (error out=w667:errorcluster, "Value"=w666:bool)  [unwired: 1 in, 1 out]
            n216 = property on="Trigger pulses" class="DigNum (strict)"("Value"=w645) -> ()  [unwired: 2 in, 2 out]
            n217 = property on="Initial frames" class="DigNum (strict)"("Value"=w651) -> ()  [unwired: 2 in, 2 out]
            n218 = property on="HALF DC" class="Bool (strict)"() -> ("Value"=w620:bool)  [unwired: 2 in, 2 out]
            n219 = property on="473 nm" class="Bool (strict)"(error in=w667, "Value"=w666) -> (error out=w665:errorcluster)  [unwired: 1 in, 1 out]
            n220 = property class="DAQmx Timing"(reference=w688, error in=w687, "SampQuant.SampMode"=w631, "SampQuant.SampPerChan"=w632) -> (reference out=w681:refnum<k21>, error out=w680:errorcluster)
            n221 = property class="DAQmx Timing"(reference=w692, error in=w690, "SampQuant.SampMode"=w631, "SampQuant.SampPerChan"=w632) -> (reference out=w691:refnum<k21>, error out=w689:errorcluster)
            n222 = property on="Low Power\nFrames" class="DigNum (strict)"("DisabledEnum"=w617) -> ("Value"=w619:i32)  [unwired: 2 in, 2 out]
            n223 = property on="Laser pulses" class="DigNum (strict)"("Value"=w632) -> ()  [unwired: 2 in, 2 out]
            n224 = property class="DAQmx Trigger"(reference=w677, error in=w675, "Start:Trigger Type"=w678) -> (reference out=w676:refnum<k21>, error out=w674:errorcluster)
            n225 = property on="561 nm 2" class="Bool (strict)"(error in=w665) -> (error out=w670:errorcluster, "Value"=w669:bool)  [unwired: 1 in, 1 out]
            n226 = case shown="True" w620 {
              tunnel: w619 -> [_ w722]
              tunnel: [w721 w722] -> w618
              frame False {
                n227 = property on="Full Power \nFrames" class="DigNum (strict)"() -> ("Value"=w721:i32)  [unwired: 2 in, 2 out]
              }
              frame True {
              }
            }
            n228 = property on="561 nm" class="Bool (strict)"(error in=w670, "Value"=w669) -> (error out=w663:errorcluster)  [unwired: 1 in, 1 out]
            n229 = property on="Illuminated Frames" class="DigNum (strict)"("Value"=w618) -> ()  [unwired: 2 in, 2 out]
            n230 = property on="Link rates 2" class="Bool (strict)"(error in=w663, "Value"=TRUE ("Link rates 2")) -> (error out=w611:errorcluster)  [unwired: 1 in, 1 out]
            n231 = property on="Enable pump control" class="Bool (strict)"(error in=w611) -> (error out=w610:errorcluster, "Value"=w612:bool)  [unwired: 1 in, 1 out]
            n232 = property on="Link shutters 2" class="Bool (strict)"(error in=w610) -> (error out=w657:errorcluster, "Value"=w658:bool)  [unwired: 1 in, 1 out]
            n233 = property on="Link shutters" class="Bool (strict)"(error in=w657, "Value"=w658) -> (error out=w656:errorcluster)  [unwired: 1 in, 1 out]
            n234 = property on="EPI 3" class="Bool (strict)"(error in=w656) -> (error out=w659:errorcluster, "Value"=w661:bool)  [unwired: 1 in, 1 out]
            n235 = property on="EPI" class="Bool (strict)"(error in=w659, "Value"=w661) -> (error out=w655:errorcluster)  [unwired: 1 in, 1 out]
            n236 = property on="FRAP 3" class="Bool (strict)"(error in=w655) -> (error out=w654:errorcluster, "Value"=w660:bool)  [unwired: 1 in, 1 out]
            n237 = property on="FRAP" class="Bool (strict)"(error in=w654, "Value"=w660) -> (error out=w625:errorcluster)  [unwired: 1 in, 1 out]
            n238 = property on="HALF DC 2" class="Bool (strict)"(error in=w625) -> (error out=w624:errorcluster, "Value"=w622:bool, "BoolText.Text"=w616:string)  [unwired: 1 in, 1 out]
            n239 = property on="HALF DC" class="Bool (strict)"(error in=w624, "Value"=w622, "BoolText.Text"=w616, "DisabledEnum"=w617) -> (error out=w641:errorcluster)  [unwired: 1 in, 1 out]
            n240 = property on="Link rates" class="Bool (strict)"(error in=w641, "DisabledEnum"=w617) -> (error out=w640:errorcluster)  [unwired: 1 in, 1 out]
            n241 = property on="Frequency 1" class="Knob (strict)"(error in=w640, "DisabledEnum"=w617) -> (error out=w639:errorcluster)  [unwired: 1 in, 1 out]
            n242 = property on="Duty Cycle 1" class="Knob (strict)"(error in=w639, "DisabledEnum"=w617, "Value"=w633) -> (error out=w629:errorcluster)  [unwired: 1 in, 1 out]
            n243 = property on="AFLEX warning" class="Bool (strict)"(error in=w629, "DisabledEnum"=w617) -> (error out=w621:errorcluster)  [unwired: 1 in, 1 out]
            n244 = property on="Populate" class="Bool"(error in=w621, "DisabledEnum"=w617) -> ()  [unwired: 1 in, 2 out]
            n245 = case shown="True" w612 {
              tunnel: [1 w718] -> w613
              frame False {
              }
              frame True {
                n246 = Add(x="Shots after pump start", y="Shots before pump start") -> (x+y=w718:i32)
              }
            }
            "Shots to acquire" <- w613
          }
          frame "Continous camera triggering" {
            w767 = 10230 items=["Analog Edge"=10099, "Digital Edge"=10150, "Digital Pattern"=10398, "Analog Window"=10103, "None"=10230] ("Start.TrigType")
            w739 = T2."Disabled and Grayed Out" ("Disabled")
            w773 = 10123 items=["Finite Samples"=10178, "Continuous Samples"=10123, "Hardware Timed Single Point"=12522] ("SampQuant.SampMode")
            n247 = property on="Link shutters" class="Bool (strict)"() -> (error out=w754:errorcluster, "Value"=w755:bool)  [unwired: 2 in, 1 out]
            n248 = property on="Link rates 2" class="Bool (strict)"(error in=w759, "DisabledEnum"=w739) -> (error out=w735:errorcluster)  [unwired: 1 in, 1 out]
            n249 = property on="Link shutters 2" class="Bool (strict)"(error in=w754, "Value"=w755) -> (error out=w753:errorcluster)  [unwired: 1 in, 1 out]
            n250 = property on="Power control" class="Bool (strict)"() -> ("Value"=w738:bool)  [unwired: 2 in, 2 out]
            n251 = property on="HALF DC" class="Bool (strict)"(error in=w735) -> (error out=w734:errorcluster, "Value"=w733:bool, "BoolText.Text"=w724:string)  [unwired: 1 in, 1 out]
            "HALF DC TEXT" <- w724
            n252 = property on="EPI 3" class="Bool (strict)"(error in=w753) -> (error out=w756:errorcluster, "Value"=w758:bool)  [unwired: 1 in, 1 out]
            n253 = case shown="False" w738 {
              tunnel: w739 -> [w774 _]
              tunnel: [w774 w775] -> w725
              tunnel: [w774 w775] -> w727
              frame False {
              }
              frame True {
                w775 = T2."Enabled" ("Disabled")
              }
            }
            n254 = property on="EPI 2" class="Bool (strict)"(error in=w756, "Value"=w758) -> (error out=w752:errorcluster)  [unwired: 1 in, 1 out]
            n255 = property on="HALF DC 2" class="Bool (strict)"(error in=w734, "Value"=w733, "BoolText.Text"=w724, "DisabledEnum"=w725) -> (error out=w760:errorcluster)  [unwired: 1 in, 1 out]
            n256 = property on="FRAP 3" class="Bool (strict)"(error in=w752) -> (error out=w751:errorcluster, "Value"=w757:bool)  [unwired: 1 in, 1 out]
            n257 = property on="Frequency 2" class="Knob (strict)"(error in=w760, "DisabledEnum"=w739) -> (error out=w729:errorcluster)  [unwired: 1 in, 1 out]
            n258 = property on="FRAP 2" class="Bool (strict)"(error in=w751, "Value"=w757) -> (error out=w750:errorcluster)  [unwired: 1 in, 1 out]
            n259 = property on="manual laser control" class="Bool (strict)"(error in=w750) -> (error out=w762:errorcluster, "Value"=w761:bool)  [unwired: 1 in, 1 out]
            n260 = case shown="True" w761 {
              selector: w761 -> [w776 _]
              tunnel: w762 -> [w777 w780]
              frame False {
                n261 = property on="ALL LASERS 2" class="Bool (strict)"(error in=w777, "Value"=w776) -> (error out=w778:errorcluster)  [unwired: 1 in, 1 out]
                n262 = property on="561 nm 2" class="Bool (strict)"(error in=w778, "Value"=w776) -> (error out=w779:errorcluster)  [unwired: 1 in, 1 out]
                n263 = property on="473 nm 2" class="Bool (strict)"(error in=w779, "Value"=w776) -> ()  [unwired: 1 in, 2 out]
              }
              frame True {
                n264 = property on="ALL LASERS" class="Bool (strict)"(error in=w780) -> (error out=w787:errorcluster, "Value"=w788:bool)  [unwired: 1 in, 1 out]
                n265 = property on="ALL LASERS 2" class="Bool (strict)"(error in=w787, "Value"=w788) -> (error out=w784:errorcluster)  [unwired: 1 in, 1 out]
                n266 = property on="561 nm" class="Bool (strict)"(error in=w784) -> (error out=w783:errorcluster, "Value"=w782:bool)  [unwired: 1 in, 1 out]
                n267 = property on="561 nm 2" class="Bool (strict)"(error in=w783, "Value"=w782) -> (error out=w781:errorcluster)  [unwired: 1 in, 1 out]
                n268 = property on="473 nm" class="Bool (strict)"(error in=w781) -> (error out=w786:errorcluster, "Value"=w785:bool)  [unwired: 1 in, 1 out]
                n269 = property on="473 nm 2" class="Bool (strict)"(error in=w786, "Value"=w785) -> ()  [unwired: 1 in, 2 out]
              }
            }
            n270 = property on="Duty Cycle 1" class="Knob (strict)"(error in=w729) -> (error out=w728:errorcluster, "Value"=w726:dbl)  [unwired: 1 in, 1 out]
            n271 = property on="Duty Cycle 2" class="Knob (strict)"(error in=w728, "Value"=w726, "DisabledEnum"=w727) -> (error out=w732:errorcluster)  [unwired: 1 in, 1 out]
            n272 = Greater?(x=w726, y=0.5) -> (0:w743:bool)
            n273 = property on="Duty Cycle \nDenominator" class="DigNum (strict)"(error in=w732) -> (error out=w731:errorcluster, "Value"=w730:dbl)  [unwired: 1 in, 1 out]
            n274 = Select(t="WARNING! Laser DC > 0.5\nAFLEX not possible", s=w743, f="AFLEX conditions\nnormal") -> (s? t:f=w744:string)
            n275 = property on="Duty Cycle \nDenominator 2" class="DigNum (strict)"(error in=w731, "Value"=w730, "DisabledEnum"=w727) -> (error out=w737:errorcluster)  [unwired: 1 in, 1 out]
            n276 = property on="AFLEX warning 2" class="Bool (strict)"(error in=w741, "Caption.Text"=w744, "Value"=w743, "DisabledEnum"=w739) -> (error out=w742:errorcluster)  [unwired: 1 in, 1 out]
            n277 = property on="Populate" class="Bool"(error in=w737, "DisabledEnum"=w727) -> (error out=w736:errorcluster)  [unwired: 1 in, 1 out]
            n278 = property class="DAQmx Channel"(reference=w772, error in=w736, "CO.Pulse.Freq"="Frame rate 2", "CO.Pulse.DutyCyc"="Duty Cycle camera 2") -> (reference out=w771:refnum<k21>, error out=w770:errorcluster)
            n279 = property class="DAQmx Timing"(reference=w771, error in=w770, "Sample Quantity:Sample Mode"=w773) -> (reference out=w766:refnum<k21>, error out=w764:errorcluster)
            n280 = property class="DAQmx Trigger"(reference=w766, error in=w764, "Start:Trigger Type"=w767) -> (reference out=w765:refnum<k21>, error out=w763:errorcluster)
            "Frame Rate display" <- "Frame rate 2"
          }
          frame "Pump control" {
            n281 = property on="473 nm" class="Bool (strict)"() -> (error out=w792:errorcluster, "Value"=w793:bool)  [unwired: 2 in, 1 out]
            n282 = property on="473 nm 2" class="Bool (strict)"(error in=w792, "Value"=w793) -> (error out=w791:errorcluster)  [unwired: 1 in, 1 out]
            n283 = property on="561 nm" class="Bool (strict)"(error in=w791) -> (error out=w790:errorcluster, "Value"=w789:bool)  [unwired: 1 in, 1 out]
            n284 = property on="561 nm 2" class="Bool (strict)"(error in=w790, "Value"=w789) -> ()  [unwired: 1 in, 2 out]
          }
        }
        n285 = Merge Errors(w597, w593, w595) -> (w607:errorcluster)
      }
      event "Continous ill": Value Change {
        (unwired) T2."Disabled and Grayed Out" ("Disabled")
        (unwired) 0.05 ("x")
        (unwired) 0.05 ("y")
        # "Trigger"
        # "473 nm"
        # "561 nm"
        n286 = event-data() -> ()  [unwired: 1 in, 1 out]
        n287 = local read "Frame rate"() -> (w804:dbl)
        n288 = call <vilib>:"DAQmx Stop Task.vi"("task/channels in"=w854, "error in"=w853) -> ("task out"=w841:refnum<k21>, "error out"=w840:errorcluster)  [unwired: 12 in]
        n289 = local read "Frequency 1"() -> (w817:dbl)
        n290 = property on="Continous ill" class="Bool (strict)"() -> ("Value"=w820:bool)  [unwired: 2 in, 2 out]
        n291 = call <vilib>:"DAQmx Stop Task.vi"("task/channels in"=w859, "error in"=w855) -> ("task out"=w847:refnum<k21>, "error out"=w846:errorcluster)  [unwired: 12 in]
        n292 = call <vilib>:"DAQmx Stop Task.vi"("task/channels in"=w858, "error in"=w856) -> ("task out"=w844:refnum<k21>, "error out"=w843:errorcluster)  [unwired: 12 in]
        n293 = local read "Duty Cycle camera"() -> (w845:dbl)
        n294 = local read "First frame\ndelay (ms)"() -> (w849:dbl)
        n295 = property class="DAQmx Channel"(reference=w847, error in=w846, "CO.Pulse.Freq"=w804, "CO.Pulse.DutyCyc"=w845) -> (reference out=w836:refnum<k21>, error out=w834:errorcluster)
        n296 = Divide(x=w849, y=1000) -> (x/y=w810:dbl)
        n297 = Multiply(x=w804, y=w810) -> (x*y=w851:dbl)
        n298 = To Long Integer(number=w851) -> (32bit integer=w831:i32)
        n299 = Reciprocal(x=w804) -> (1/x=w850:dbl)
        n300 = local read "Illuminated Frames"() -> (w819:i32)
        n301 = Multiply(x=w831, y=w850) -> (x*y=w813:dbl)
        n302 = property on="laser delay (s)" class="DigNum (strict)"("Value"=w813) -> ()  [unwired: 2 in, 2 out]
        n303 = local read "Finishing frames"() -> (w832:i32)
        n304 = property on="Initial calculated\ndelay (frames)" class="DigNum (strict)"("Value"=w851) -> ()  [unwired: 2 in, 2 out]
        n305 = Multiply(x=w813, y=1000) -> (x*y=w842:dbl)
        n306 = property on="Laser delay (ms)" class="DigNum (strict)"("Value"=w842) -> ()  [unwired: 2 in, 2 out]
        n307 = Add(x=w819, y=w831) -> (x+y=w821:i32)
        n308 = property on="delay\ncompensation" class="DigNum (strict)"() -> ("Value"=w801:dbl)  [unwired: 2 in, 2 out]
        n309 = Divide(x=w819, y=2) -> (x/y=w822:dbl)
        n310 = Add(x=w832, y=w821) -> (x+y=w803:i32)
        n311 = property class="DAQmx Timing"(reference=w836, error in=w834, "SampQuant.SampPerChan"=w803) -> (reference out=w835:refnum<k21>, error out=w833:errorcluster)
        n312 = To Long Integer(number=w822) -> (32bit integer=w815:i32)
        n313 = case shown="True" w820 {
          tunnel: [w869 w890] -> w816
          tunnel: w804 -> [w874 w895]
          tunnel: w817 -> [w875 _]
          tunnel: w819 -> [_ w893]
          tunnel: [w872 1] -> w814
          tunnel: [w861 w887] -> w818
          tunnel: w815 -> [w872 _]
          tunnel: [w868 0.0] -> w808
          frame False {
            w860 = T2."Enabled" ("Disabled")
            n314 = property on="Link rates" class="Bool (strict)"() -> ("Value"=w873:bool)  [unwired: 2 in, 2 out]
            n315 = property on="Duty Cycle 1\npreset" class="Knob (strict)"() -> ("Value"=w861:dbl)  [unwired: 2 in, 2 out]
            n316 = Greater?(x=w861, y=0.5) -> (0:w862:bool)
            n317 = case shown="True" w873 {
              tunnel: [w877 w879] -> w869
              tunnel: w874 -> [_ w881]
              tunnel: w875 -> [w877 _]
              tunnel: w860 -> [w876 w878]
              frame False {
                n318 = property on="Frequency 1" class="Knob (strict)"("DisabledEnum"=w876) -> ()  [unwired: 2 in, 2 out]
              }
              frame True {
                n319 = Divide(x=w881, y=2) -> (x/y=w879:dbl)
                n320 = property on="Frequency 1" class="Knob (strict)"("Value"=w879, "DisabledEnum"=w878) -> ()  [unwired: 2 in, 2 out]
              }
            }
            n321 = property on="HALF DC" class="Bool (strict)"("DisabledEnum"=w860) -> ()  [unwired: 2 in, 2 out]
            n322 = Select(t="WARNING! Laser DC > 0.5\nAFLEX not possible", s=w862, f="AFLEX conditions\nnormal") -> (s? t:f=w863:string)
            n323 = property on="Duty Cycle 1" class="Knob (strict)"("Value"=w861, "Scale.Maximum"=0.5 ("Scale.Range:Maximum"), "DisabledEnum"=w860) -> ()  [unwired: 2 in, 2 out]
            n324 = property on="AFLEX warning" class="Bool (strict)"("DisabledEnum"=w860, "Caption.Text"=w863, "Value"=w862) -> ()  [unwired: 2 in, 2 out]
            n325 = property on="Pulsed" class="Bool (strict)"("DisabledEnum"=w860) -> ()  [unwired: 2 in, 2 out]
            n326 = property on="Link rates" class="Bool (strict)"("DisabledEnum"=w860) -> ()  [unwired: 2 in, 2 out]
            n327 = property on="Populate" class="Bool"("DisabledEnum"=w860) -> ()  [unwired: 2 in, 2 out]
            n328 = Multiply(x=w869, y=2) -> (x*y=w871:dbl)
            n329 = Reciprocal(x=w871) -> (1/x=w868:dbl)
            n330 = property on="Low Power\nFrames" class="DigNum (strict)"("DisabledEnum"=w860) -> ()  [unwired: 2 in, 2 out]
            n331 = property on="Duty Cycle \nDenominator" class="DigNum (strict)"("DisabledEnum"=w860) -> ()  [unwired: 2 in, 2 out]
          }
          frame True {
            w883 = T2."Disabled and Grayed Out" ("Disabled")
            w887 = 0.9999 ("x")
            n332 = Reciprocal(x=w895) -> (1/x=w894:dbl)
            n333 = Multiply(x=w894, y=w893) -> (x*y=w891:dbl)
            n334 = property on="Link rates" class="Bool (strict)"("DisabledEnum"=w883) -> ()  [unwired: 2 in, 2 out]
            n335 = property on="Duty Cycle 1" class="Knob (strict)"("Value"=w887, "Scale.Maximum"=w887, "DisabledEnum"=w883) -> ()  [unwired: 2 in, 2 out]
            n336 = property on="AFLEX warning" class="Bool (strict)"("Caption.Text"="AFLEX conditions\nnormal" ("f"), "Value"=FALSE, "DisabledEnum"=w883) -> ()  [unwired: 2 in, 2 out]
            n337 = Divide(x=w887, y=w891) -> (x/y=w890:dbl)
            n338 = property on="Power control" class="Bool (strict)"() -> ("Value"=w884:bool)  [unwired: 2 in, 2 out]
            n339 = property on="Frequency 1" class="Knob (strict)"("Value"=w890, "DisabledEnum"=w883) -> ()  [unwired: 2 in, 2 out]
            n340 = case shown="True" w884 {
              tunnel: w883 -> [w896 _]
              tunnel: [w896 T2."Enabled" ("Disabled")] -> w882
              frame False {
              }
              frame True {
              }
            }
            n341 = property on="Duty Cycle \nDenominator" class="DigNum (strict)"("DisabledEnum"=w882) -> ()  [unwired: 2 in, 2 out]
            n342 = property on="Low Power\nFrames" class="DigNum (strict)"("DisabledEnum"=w882) -> ()  [unwired: 2 in, 2 out]
            n343 = property on="Pulsed" class="Bool (strict)"("Value"=FALSE ("Pulsed")) -> ()  [unwired: 2 in, 2 out]
            n344 = property on="Populate" class="Bool"("DisabledEnum"=w882) -> ()  [unwired: 2 in, 2 out]
            n345 = property on="HALF DC" class="Bool (strict)"("DisabledEnum"=w882) -> ()  [unwired: 2 in, 2 out]
          }
        }
        n346 = Add(x=w813, y=w808) -> (x+y=w837:dbl)
        n347 = Multiply(x=w808, y=1000) -> (x*y=w838:dbl)
        n348 = property class="DAQmx Channel"(reference=w844, error in=w843, "CO.Pulse.Freq"=w816, "CO.Pulse.DutyCyc"=w818, "CO.Pulse.Freq.InitialDelay"=w813) -> (reference out=w827:refnum<k21>, error out=w825:errorcluster)
        n349 = property class="DAQmx Channel"(reference=w841, error in=w840, "CO.Pulse.Freq"=w816, "CO.Pulse.DutyCyc"=w818, "CO.Pulse.Freq.InitialDelay"=w837) -> (reference out=w830:refnum<k21>, error out=w828:errorcluster)
        n350 = property on="Initial delay\n473 nm (ms)" class="DigNum (strict)"("Value"=w838) -> ()  [unwired: 2 in, 2 out]
        n351 = property class="DAQmx Timing"(reference=w827, error in=w825, "SampQuant.SampPerChan"=w814) -> (reference out=w826:refnum<k21>, error out=w824:errorcluster)
        n352 = property on="Trigger pulses" class="DigNum (strict)"("Value"=w803) -> ()  [unwired: 2 in, 2 out]
        n353 = property on="Laser pulses" class="DigNum (strict)"("Value"=w814) -> ()  [unwired: 2 in, 2 out]
        n354 = property class="DAQmx Timing"(reference=w830, error in=w828, "SampQuant.SampPerChan"=w814) -> (reference out=w829:refnum<k21>, error out=w802:errorcluster)
        n355 = Multiply(x=w801, y=w804) -> (x*y=w805:dbl)
        n356 = To Long Integer(number=w805) -> (32bit integer=w806:i32)
        n357 = Subtract(x=w810, y=w801) -> (x-y=w811:dbl)
        n358 = Subtract(x=w803, y=w806) -> (x-y=w807:i32)
        n359 = Multiply(x=w804, y=w811) -> (x*y=w812:dbl)
        n360 = property on="Frames to acquire" class="DigNum (strict)"("Value"=w807) -> ()  [unwired: 2 in, 2 out]
        n361 = To Long Integer(number=w812) -> (32bit integer=w809:i32)
        n362 = Merge Errors(w833, w824, w802) -> (w857:errorcluster)
        n363 = property on="Initial frames" class="DigNum (strict)"("Value"=w809) -> ()  [unwired: 2 in, 2 out]
      }
      event "Pulsed": Value Change {
        (unwired) 0.05 ("x")
        (unwired) 0.05 ("y")
        # "Trigger"
        # "473 nm"
        # "561 nm"
        n364 = event-data() -> ()  [unwired: 1 in, 1 out]
        n365 = local read "Frame rate"() -> (w902:dbl)
        n366 = call <vilib>:"DAQmx Stop Task.vi"("task/channels in"=w952, "error in"=w951) -> ("task out"=w939:refnum<k21>, "error out"=w938:errorcluster)  [unwired: 12 in]
        n367 = local read "Frequency 1"() -> (w915:dbl)
        n368 = call <vilib>:"DAQmx Stop Task.vi"("task/channels in"=w957, "error in"=w953) -> ("task out"=w945:refnum<k21>, "error out"=w944:errorcluster)  [unwired: 12 in]
        n369 = call <vilib>:"DAQmx Stop Task.vi"("task/channels in"=w956, "error in"=w954) -> ("task out"=w942:refnum<k21>, "error out"=w941:errorcluster)  [unwired: 12 in]
        n370 = local read "Duty Cycle camera"() -> (w943:dbl)
        n371 = local read "First frame\ndelay (ms)"() -> (w947:dbl)
        n372 = property class="DAQmx Channel"(reference=w945, error in=w944, "CO.Pulse.Freq"=w902, "CO.Pulse.DutyCyc"=w943) -> (reference out=w934:refnum<k21>, error out=w932:errorcluster)
        n373 = Divide(x=w947, y=1000) -> (x/y=w908:dbl)
        n374 = Multiply(x=w902, y=w908) -> (x*y=w949:dbl)
        n375 = To Long Integer(number=w949) -> (32bit integer=w929:i32)
        n376 = Reciprocal(x=w902) -> (1/x=w948:dbl)
        n377 = local read "Illuminated Frames"() -> (w917:i32)
        n378 = Multiply(x=w929, y=w948) -> (x*y=w911:dbl)
        n379 = property on="laser delay (s)" class="DigNum (strict)"("Value"=w911) -> ()  [unwired: 2 in, 2 out]
        n380 = local read "Finishing frames"() -> (w930:i32)
        n381 = property on="Initial calculated\ndelay (frames)" class="DigNum (strict)"("Value"=w949) -> ()  [unwired: 2 in, 2 out]
        n382 = Multiply(x=w911, y=1000) -> (x*y=w940:dbl)
        n383 = property on="Laser delay (ms)" class="DigNum (strict)"("Value"=w940) -> ()  [unwired: 2 in, 2 out]
        n384 = Add(x=w917, y=w929) -> (x+y=w918:i32)
        n385 = property on="delay\ncompensation" class="DigNum (strict)"() -> ("Value"=w898:dbl)  [unwired: 2 in, 2 out]
        n386 = Divide(x=w917, y=2) -> (x/y=w919:dbl)
        n387 = Add(x=w930, y=w918) -> (x+y=w901:i32)
        n388 = property class="DAQmx Timing"(reference=w934, error in=w932, "SampQuant.SampPerChan"=w901) -> (reference out=w933:refnum<k21>, error out=w931:errorcluster)
        n389 = To Long Integer(number=w919) -> (32bit integer=w913:i32)
        n390 = case shown="True" "Pulsed" {
          tunnel: [w967 w988] -> w914
          tunnel: w902 -> [w972 w988]
          tunnel: w915 -> [w973 _]
          tunnel: w917 -> [_ w990]
          tunnel: [w970 w990] -> w912
          tunnel: [w959 w981] -> w916
          tunnel: w913 -> [w970 _]
          tunnel: [w966 0.0] -> w906
          frame False {
            w958 = T2."Enabled" ("Disabled")
            n391 = property on="Duty Cycle 1\npreset" class="Knob (strict)"() -> ("Value"=w959:dbl)  [unwired: 2 in, 2 out]
            n392 = property on="Link rates" class="Bool (strict)"() -> ("Value"=w971:bool)  [unwired: 2 in, 2 out]
            n393 = property on="Duty Cycle 1" class="Knob (strict)"("Value"=w959, "Scale.Maximum"=0.5 ("Scale.Range:Maximum"), "DisabledEnum"=w958) -> ()  [unwired: 2 in, 2 out]
            n394 = case shown="True" w971 {
              tunnel: [w975 w977] -> w967
              tunnel: w972 -> [_ w979]
              tunnel: w973 -> [w975 _]
              tunnel: w958 -> [w974 w976]
              frame False {
                n395 = property on="Frequency 1" class="Knob (strict)"("DisabledEnum"=w974) -> ()  [unwired: 2 in, 2 out]
              }
              frame True {
                n396 = Divide(x=w979, y=2) -> (x/y=w977:dbl)
                n397 = property on="Frequency 1" class="Knob (strict)"("Value"=w977, "DisabledEnum"=w976) -> ()  [unwired: 2 in, 2 out]
              }
            }
            n398 = Greater?(x=w959, y=0.5) -> (0:w960:bool)
            n399 = Select(t="WARNING! Laser DC > 0.5\nAFLEX not possible", s=w960, f="AFLEX conditions\nnormal") -> (s? t:f=w961:string)
            n400 = property on="Link rates" class="Bool (strict)"("DisabledEnum"=w958) -> ()  [unwired: 2 in, 2 out]
            n401 = property on="Continous ill" class="Bool (strict)"("DisabledEnum"=w958) -> ()  [unwired: 2 in, 2 out]
            n402 = Multiply(x=w967, y=2) -> (x*y=w969:dbl)
            n403 = property on="AFLEX warning" class="Bool (strict)"("Caption.Text"=w961, "Value"=w960, "DisabledEnum"=w958) -> ()  [unwired: 2 in, 2 out]
            n404 = Reciprocal(x=w969) -> (1/x=w966:dbl)
          }
          frame True {
            w980 = T2."Enabled" ("Disabled")
            w982 = T2."Disabled and Grayed Out" ("Disabled")
            n405 = property on="Duty Cycle 1\npreset" class="Knob (strict)"() -> ("Value"=w981:dbl)  [unwired: 2 in, 2 out]
            n406 = Greater?(x=w981, y=0.5) -> (0:w983:bool)
            n407 = flat-sequence {
              tunnel: w981 -> [w993]
              frame #0 {
                n408 = property on="Continous ill" class="Bool (strict)"() -> ("Value"=w992:bool)  [unwired: 2 in, 2 out]
                n409 = case shown="False" w992 {
                  tunnel: w993 -> [w994 _]
                  frame False {
                    n410 = property on="Duty Cycle 1\npreset" class="Knob (strict)"("Value"=w994) -> ()  [unwired: 2 in, 2 out]
                  }
                  frame True {
                  }
                }
              }
              frame #1 {
                n411 = property on="Continous ill" class="Bool (strict)"("Value"=FALSE ("Pulsed")) -> ()  [unwired: 2 in, 2 out]
              }
            }
            n412 = property on="Duty Cycle 1" class="Knob (strict)"("Value"=w981, "Scale.Maximum"=0.9999 ("x"), "DisabledEnum"=w980) -> ()  [unwired: 2 in, 2 out]
            n413 = Select(t="WARNING! Laser DC > 0.5\nAFLEX not possible", s=w983, f="AFLEX conditions\nnormal") -> (s? t:f=w984:string)
            n414 = property on="Low Power\nFrames" class="DigNum (strict)"("DisabledEnum"=w980) -> ()  [unwired: 2 in, 2 out]
            n415 = property on="Populate" class="Bool"("DisabledEnum"=w980) -> ()  [unwired: 2 in, 2 out]
            n416 = property on="Duty Cycle \nDenominator" class="DigNum (strict)"("DisabledEnum"=w980) -> ()  [unwired: 2 in, 2 out]
            n417 = property on="AFLEX warning" class="Bool (strict)"("DisabledEnum"=w982, "Caption.Text"=w984, "Value"=w983) -> ()  [unwired: 2 in, 2 out]
            n418 = property on="Frequency 1" class="Knob (strict)"("Value"=w988, "DisabledEnum"=w982) -> ()  [unwired: 2 in, 2 out]
            n419 = property on="Link rates" class="Bool (strict)"("DisabledEnum"=w982) -> ()  [unwired: 2 in, 2 out]
          }
        }
        n420 = Add(x=w911, y=w906) -> (x+y=w935:dbl)
        n421 = Multiply(x=w906, y=1000) -> (x*y=w936:dbl)
        n422 = property class="DAQmx Channel"(reference=w942, error in=w941, "CO.Pulse.Freq"=w914, "CO.Pulse.DutyCyc"=w916, "CO.Pulse.Freq.InitialDelay"=w911) -> (reference out=w924:refnum<k21>, error out=w922:errorcluster)
        n423 = property class="DAQmx Channel"(reference=w939, error in=w938, "CO.Pulse.Freq"=w914, "CO.Pulse.DutyCyc"=w916, "CO.Pulse.Freq.InitialDelay"=w935) -> (reference out=w928:refnum<k21>, error out=w926:errorcluster)
        n424 = property on="Initial delay\n473 nm (ms)" class="DigNum (strict)"("Value"=w936) -> ()  [unwired: 2 in, 2 out]
        n425 = property class="DAQmx Timing"(reference=w924, error in=w922, "SampQuant.SampPerChan"=w912) -> (reference out=w923:refnum<k21>, error out=w921:errorcluster)
        n426 = property on="Trigger pulses" class="DigNum (strict)"("Value"=w901) -> ()  [unwired: 2 in, 2 out]
        n427 = property on="Laser pulses" class="DigNum (strict)"("Value"=w912) -> ()  [unwired: 2 in, 2 out]
        n428 = property class="DAQmx Timing"(reference=w928, error in=w926, "SampQuant.SampPerChan"=w912) -> (reference out=w927:refnum<k21>, error out=w925:errorcluster)
        n429 = Multiply(x=w898, y=w902) -> (x*y=w903:dbl)
        n430 = To Long Integer(number=w903) -> (32bit integer=w904:i32)
        n431 = Subtract(x=w908, y=w898) -> (x-y=w909:dbl)
        n432 = Subtract(x=w901, y=w904) -> (x-y=w905:i32)
        n433 = Multiply(x=w902, y=w909) -> (x*y=w910:dbl)
        n434 = property on="HALF DC" class="Bool (strict)"("DisabledEnum"=T2."Enabled" ("Disabled")) -> ()  [unwired: 2 in, 2 out]
        n435 = property on="Frames to acquire" class="DigNum (strict)"("Value"=w905) -> ()  [unwired: 2 in, 2 out]
        n436 = To Long Integer(number=w910) -> (32bit integer=w907:i32)
        n437 = Merge Errors(w931, w921, w925) -> (w955:errorcluster)
        n438 = property on="Initial frames" class="DigNum (strict)"("Value"=w907) -> ()  [unwired: 2 in, 2 out]
      }
      event "EPI": Value Change {
        n439 = event-data() -> ()  [unwired: 1 in, 1 out]
        n440 = property on="EPI 3" class="Bool (strict)"(error in=w998, "Value"="EPI") -> (error out=w997:errorcluster)  [unwired: 1 in, 1 out]
        n441 = call <vilib>:"DAQmx Stop Task.vi"("task/channels in"=w1019, "error in"=w1015) -> ("task out"=w1004:refnum<k21>, "error out"=w1003:errorcluster)  [unwired: 12 in]
        n442 = call <vilib>:"DAQmx Stop Task.vi"("task/channels in"=w1018, "error in"=w1016) -> ("task out"=w1002:refnum<k21>, "error out"=w1001:errorcluster)  [unwired: 12 in]
        n443 = call <vilib>:"DAQmx Stop Task.vi"("task/channels in"=w1014, "error in"=w1013) -> ("task out"=w999:refnum<k21>, "error out"=w1000:errorcluster)  [unwired: 12 in]
        n444 = case shown="True" "Link shutters" {
          tunnel: w1011 -> [w1025 w1038]
          tunnel: w997 -> [w1024 w1037]
          tunnel: w1010 -> [w1021 w1036]
          tunnel: w1009 -> [w1020 w1035]
          tunnel: [w1020 w1028] -> w1005
          tunnel: [w1021 w1033] -> w1006
          tunnel: [w1023 w1032] -> w1008
          tunnel: [w1022 w1031] -> w1007
          tunnel: "EPI" -> [w1026 w1030]
          frame False {
            n445 = call-poly <vilib>:"DAQmx Write.vi"("task/channels in"=w1025, "data"=w1026, "error in"=w1024) -> ("task out"=w1023:refnum<k21>, "error out"=w1022:errorcluster)  [unwired: 10 in, 1 out]
          }
          frame True {
            n446 = Not(x=w1030) -> (.not. x?=w1027:bool)
            n447 = call-poly <vilib>:"DAQmx Write.vi"("task/channels in"=w1038, "data"=w1030, "error in"=w1037) -> ("task out"=w1032:refnum<k21>, "error out"=w1031:errorcluster)  [unwired: 10 in, 1 out]
            n448 = call-poly <vilib>:"DAQmx Write.vi"("task/channels in"=w1036, "data"=w1027, "error in"=w1035) -> ("task out"=w1033:refnum<k21>, "error out"=w1034:errorcluster)  [unwired: 10 in, 1 out]
            n449 = property on="FRAP" class="Bool (strict)"(error in=w1034, "Value"=w1027) -> (error out=w1029:errorcluster)  [unwired: 1 in, 1 out]
            n450 = property on="FRAP 3" class="Bool (strict)"(error in=w1029, "Value"=w1027) -> (error out=w1028:errorcluster)  [unwired: 1 in, 1 out]
          }
        }
        n451 = Merge Errors(w1003, w1001, w1000) -> (w1017:errorcluster)
      }
      event "FRAP": Value Change {
        n452 = event-data() -> ()  [unwired: 1 in, 1 out]
        n453 = call <vilib>:"DAQmx Stop Task.vi"("task/channels in"=w1057, "error in"=w1056) -> ("task out"=w1047:refnum<k21>, "error out"=w1046:errorcluster)  [unwired: 12 in]
        n454 = property on="FRAP 3" class="Bool (strict)"(error in=w1041, "Value"="FRAP") -> (error out=w1040:errorcluster)  [unwired: 1 in, 1 out]
        n455 = call <vilib>:"DAQmx Stop Task.vi"("task/channels in"=w1062, "error in"=w1058) -> ("task out"=w1042:refnum<k21>, "error out"=w1043:errorcluster)  [unwired: 12 in]
        n456 = call <vilib>:"DAQmx Stop Task.vi"("task/channels in"=w1061, "error in"=w1059) -> ("task out"=w1044:refnum<k21>, "error out"=w1045:errorcluster)  [unwired: 12 in]
        n457 = property on="Link shutters" class="Bool (strict)"() -> ("Value"=w1052:bool)  [unwired: 2 in, 2 out]
        n458 = case shown="True" w1052 {
          tunnel: w1055 -> [w1064 w1079]
          tunnel: w1054 -> [w1065 w1073]
          tunnel: w1053 -> [w1068 w1080]
          tunnel: w1040 -> [w1067 w1074]
          tunnel: [w1066 w1075] -> w1048
          tunnel: [w1063 w1078] -> w1049
          tunnel: [w1064 w1077] -> w1051
          tunnel: [w1065 w1076] -> w1050
          tunnel: "FRAP" -> [w1069 w1081]
          frame False {
            n459 = call-poly <vilib>:"DAQmx Write.vi"("task/channels in"=w1068, "data"=w1069, "error in"=w1067) -> ("task out"=w1063:refnum<k21>, "error out"=w1066:errorcluster)  [unwired: 10 in, 1 out]
          }
          frame True {
            n460 = Not(x=w1081) -> (.not. x?=w1070:bool)
            n461 = call-poly <vilib>:"DAQmx Write.vi"("task/channels in"=w1080, "data"=w1081, "error in"=w1074) -> ("task out"=w1078:refnum<k21>, "error out"=w1075:errorcluster)  [unwired: 10 in, 1 out]
            n462 = call-poly <vilib>:"DAQmx Write.vi"("task/channels in"=w1079, "data"=w1070, "error in"=w1073) -> ("task out"=w1077:refnum<k21>, "error out"=w1072:errorcluster)  [unwired: 10 in, 1 out]
            n463 = property on="EPI 3" class="Bool (strict)"(error in=w1072, "Value"=w1070) -> (error out=w1071:errorcluster)  [unwired: 1 in, 1 out]
            n464 = property on="EPI" class="Bool (strict)"(error in=w1071, "Value"=w1070) -> (error out=w1076:errorcluster)  [unwired: 1 in, 1 out]
          }
        }
        n465 = Merge Errors(w1043, w1045, w1046) -> (w1060:errorcluster)
      }
      event "Power control": Value Change {
        n466 = event-data() -> ()  [unwired: 1 in, 1 out]
        n467 = call <vilib>:"DAQmx Stop Task.vi"("task/channels in"=w1111, "error in"=w1107) -> ("task out"=w1097:refnum<k21>, "error out"=w1098:errorcluster)  [unwired: 12 in]
        n468 = call <vilib>:"DAQmx Stop Task.vi"("task/channels in"=w1110, "error in"=w1108) -> ("task out"=w1099:refnum<k21>, "error out"=w1100:errorcluster)  [unwired: 12 in]
        n469 = call <vilib>:"DAQmx Stop Task.vi"("task/channels in"=w1106, "error in"=w1105) -> ("task out"=w1102:refnum<k21>, "error out"=w1101:errorcluster)  [unwired: 12 in]
        n470 = property on="Power control" class="Bool (strict)"() -> ("Value"=w1094:bool)  [unwired: 2 in, 2 out]
        n471 = case shown="False" w1094 {
          tunnel: w1093 -> [w1118 w1129]
          tunnel: w1092 -> [w1116 w1132]
          tunnel: w1091 -> [_ w1128]
          tunnel: w1090 -> [_ w1133]
          tunnel: w1089 -> [_ w1130]
          tunnel: w1088 -> [_ w1131]
          tunnel: w1087 -> [_ w1126]
          tunnel: w1086 -> [_ w1127]
          tunnel: [_ w1123] -> w1085
          tunnel: [w1115 w1125] -> w1084
          tunnel: [_ w1122] -> w1083
          tunnel: [w1114 w1124] -> w1082
          frame False {
            n472 = property on="561 task" class="DAQmxName (strict)"() -> ("Value"=w1113:refnum<k21>)  [unwired: 2 in, 2 out]
            n473 = property on="473 task" class="DAQmxName (strict)"() -> ("Value"=w1112:refnum<k21>)  [unwired: 2 in, 2 out]
            n474 = call <vilib>:"DAQmx Stop Task.vi"("task/channels in"=w1113, "error in"=w1118) -> ("task out"=w1117:refnum<k21>, "error out"=w1121:errorcluster)  [unwired: 12 in]
            n475 = call <vilib>:"DAQmx Stop Task.vi"("task/channels in"=w1112, "error in"=w1116) -> ("task out"=w1119:refnum<k21>, "error out"=w1120:errorcluster)  [unwired: 12 in]
            n476 = call <vilib>:"DAQmx Clear Task.vi"("task in"=w1117, "error in"=w1121) -> ("error out"=w1115:errorcluster)  [unwired: 13 in]
            n477 = call <vilib>:"DAQmx Clear Task.vi"("task in"=w1119, "error in"=w1120) -> ("error out"=w1114:errorcluster)  [unwired: 13 in]
          }
          frame True {
            n478 = call "LineController Analogue init v3.0.vi"("lines"=w1128, "Power level (0-1)"=w1127, "error in"=w1129, "Level at max (0-5V)"=w1126) -> ("task out"=w1123:refnum<k21>, "error out"=w1125:errorcluster)  [unwired: 1 in, 1 out]
            n479 = call "LineController Analogue init v3.0.vi"("lines"=w1133, "Power level (0-1)"=w1131, "error in"=w1132, "Level at max (0-5V)"=w1130) -> ("task out"=w1122:refnum<k21>, "error out"=w1124:errorcluster)  [unwired: 1 in, 1 out]
            n480 = property on="561 task" class="DAQmxName (strict)"("Value"=w1123) -> ()  [unwired: 2 in, 2 out]
            n481 = property on="473 task" class="DAQmxName (strict)"("Value"=w1122) -> ()  [unwired: 2 in, 2 out]
          }
        }
        n482 = Merge Errors(w1098, w1100, w1101) -> (w1109:errorcluster)
      }
      event "Illuminated Frames": Value Change {
        (unwired) 0.05 ("x")
        (unwired) 0.05 ("y")
        (unwired) 2 ("y")
        # "Trigger"
        # "473 nm"
        # "561 nm"
        n483 = event-data() -> ()  [unwired: 1 in, 1 out]
        n484 = call <vilib>:"DAQmx Stop Task.vi"("task/channels in"=w1191, "error in"=w1189) -> ("task out"=w1177:refnum<k21>, "error out"=w1176:errorcluster)  [unwired: 12 in]
        n485 = local read "Frame rate"() -> (w1142:dbl)
        n486 = call <vilib>:"DAQmx Stop Task.vi"("task/channels in"=w1187, "error in"=w1186) -> ("task out"=w1174:refnum<k21>, "error out"=w1173:errorcluster)  [unwired: 12 in]
        n487 = call <vilib>:"DAQmx Stop Task.vi"("task/channels in"=w1192, "error in"=w1188) -> ("task out"=w1180:refnum<k21>, "error out"=w1179:errorcluster)  [unwired: 12 in]
        n488 = local read "Frequency 1"() -> (w1141:dbl)
        n489 = local read "First frame\ndelay (ms)"() -> (w1182:dbl)
        n490 = property on="Continous ill" class="Bool (strict)"() -> ("Value"=w1143:bool)  [unwired: 2 in, 2 out]
        n491 = local read "Duty Cycle camera"() -> (w1178:dbl)
        n492 = property class="DAQmx Channel"(reference=w1180, error in=w1179, "CO.Pulse.Freq"=w1142, "CO.Pulse.DutyCyc"=w1178) -> (reference out=w1168:refnum<k21>, error out=w1166:errorcluster)
        n493 = Divide(x=w1182, y=1000) -> (x/y=w1149:dbl)
        n494 = Multiply(x=w1142, y=w1149) -> (x*y=w1184:dbl)
        n495 = To Long Integer(number=w1184) -> (32bit integer=w1163:i32)
        n496 = Reciprocal(x=w1142) -> (1/x=w1183:dbl)
        n497 = property on="delay\ncompensation" class="DigNum (strict)"() -> ("Value"=w1134:dbl)  [unwired: 2 in, 2 out]
        n498 = local read "Illuminated Frames"() -> (w1139:i32)
        n499 = Multiply(x=w1163, y=w1183) -> (x*y=w1169:dbl)
        n500 = local read "Finishing frames"() -> (w1164:i32)
        n501 = property on="Initial calculated\ndelay (frames)" class="DigNum (strict)"("Value"=w1184) -> ()  [unwired: 2 in, 2 out]
        n502 = Multiply(x=w1169, y=1000) -> (x*y=w1175:dbl)
        n503 = property on="Laser delay (ms)" class="DigNum (strict)"("Value"=w1175) -> ()  [unwired: 2 in, 2 out]
        n504 = Add(x=w1139, y=w1163) -> (x+y=w1152:i32)
        n505 = Subtract(x=w1149, y=w1134) -> (x-y=w1150:dbl)
        n506 = Multiply(x=w1134, y=w1142) -> (x*y=w1145:dbl)
        n507 = property on="Full Power \nFrames" class="DigNum (strict)"("Value"=w1139) -> ()  [unwired: 2 in, 2 out]
        n508 = Add(x=w1164, y=w1152) -> (x+y=w1144:i32)
        n509 = To Long Integer(number=w1145) -> (32bit integer=w1146:i32)
        n510 = Multiply(x=w1142, y=w1150) -> (x*y=w1151:dbl)
        n511 = Divide(x=w1139, y=2) -> (x/y=w1153:dbl)
        n512 = To Long Integer(number=w1153) -> (32bit integer=w1138:i32)
        n513 = case shown="False" w1143 {
          tunnel: [w1200 w1220] -> w1136
          tunnel: [w1193 1] -> w1137
          tunnel: [w1198 w1221] -> w1140
          tunnel: [w1201 0.0] -> w1135
          tunnel: w1142 -> [w1196 w1218]
          tunnel: w1141 -> [w1197 _]
          tunnel: w1138 -> [w1195 _]
          tunnel: w1139 -> [w1194 w1217]
          frame False {
            n514 = property on="Pulsed" class="Bool (strict)"() -> ("Value"=w1199:bool)  [unwired: 2 in, 2 out]
            n515 = property on="Duty Cycle 1\npreset" class="Knob (strict)"() -> ("Value"=w1198:dbl)  [unwired: 2 in, 2 out]
            n516 = case shown="False" w1199 {
              tunnel: w1198 -> [_ _]
              tunnel: [w1206 0.0] -> w1201
              tunnel: [w1205 w1215] -> w1200
              tunnel: w1197 -> [w1204 _]
              tunnel: w1196 -> [w1203 w1215]
              tunnel: w1195 -> [w1202 _]
              tunnel: w1194 -> [_ w1214]
              tunnel: [w1202 w1214] -> w1193
              frame False {
                n517 = property on="Link rates" class="Bool (strict)"() -> ("Value"=w1209:bool)  [unwired: 2 in, 2 out]
                n518 = case shown="True" w1209 {
                  tunnel: [w1210 w1212] -> w1205
                  tunnel: w1204 -> [w1210 _]
                  tunnel: w1203 -> [_ w1211]
                  frame False {
                  }
                  frame True {
                    n519 = Divide(x=w1211, y=2) -> (x/y=w1212:dbl)
                    n520 = property on="Frequency 1" class="Knob (strict)"("Value"=w1212) -> ()  [unwired: 2 in, 2 out]
                  }
                }
                n521 = Multiply(x=w1205, y=2) -> (x*y=w1208:dbl)
                n522 = Reciprocal(x=w1208) -> (1/x=w1206:dbl)
              }
              frame True {
              }
            }
            n523 = property on="Duty Cycle 1" class="Knob (strict)"("Value"=w1198) -> ()  [unwired: 2 in, 2 out]
          }
          frame True {
            w1221 = 0.9999 ("x")
            n524 = Reciprocal(x=w1218) -> (1/x=w1224:dbl)
            n525 = Multiply(x=w1224, y=w1217) -> (x*y=w1222:dbl)
            n526 = property on="Duty Cycle 1" class="Knob (strict)"("Value"=w1221) -> ()  [unwired: 2 in, 2 out]
            n527 = Divide(x=w1221, y=w1222) -> (x/y=w1220:dbl)
            n528 = property on="Frequency 1" class="Knob (strict)"("Value"=w1220) -> ()  [unwired: 2 in, 2 out]
          }
        }
        n529 = Add(x=w1169, y=w1135) -> (x+y=w1170:dbl)
        n530 = Multiply(x=w1135, y=1000) -> (x*y=w1171:dbl)
        n531 = property class="DAQmx Channel"(reference=w1177, error in=w1176, "CO.Pulse.Freq"=w1136, "CO.Pulse.DutyCyc"=w1140, "CO.Pulse.Freq.InitialDelay"=w1169) -> (reference out=w1158:refnum<k21>, error out=w1156:errorcluster)
        n532 = property class="DAQmx Channel"(reference=w1174, error in=w1173, "CO.Pulse.Freq"=w1136, "CO.Pulse.DutyCyc"=w1140, "CO.Pulse.Freq.InitialDelay"=w1170) -> (reference out=w1162:refnum<k21>, error out=w1160:errorcluster)
        n533 = property on="Initial delay\n473 nm (ms)" class="DigNum (strict)"("Value"=w1171) -> ()  [unwired: 2 in, 2 out]
        n534 = property class="DAQmx Timing"(reference=w1168, error in=w1166, "SampQuant.SampPerChan"=w1144) -> (reference out=w1167:refnum<k21>, error out=w1165:errorcluster)
        n535 = To Long Integer(number=w1151) -> (32bit integer=w1148:i32)
        n536 = Subtract(x=w1144, y=w1146) -> (x-y=w1147:i32)
        n537 = property on="Frames to acquire" class="DigNum (strict)"("Value"=w1147) -> ()  [unwired: 2 in, 2 out]
        n538 = property class="DAQmx Timing"(reference=w1162, error in=w1160, "SampQuant.SampPerChan"=w1137) -> (reference out=w1161:refnum<k21>, error out=w1159:errorcluster)
        n539 = property on="Initial frames" class="DigNum (strict)"("Value"=w1148) -> ()  [unwired: 2 in, 2 out]
        n540 = property class="DAQmx Timing"(reference=w1158, error in=w1156, "SampQuant.SampPerChan"=w1137) -> (reference out=w1157:refnum<k21>, error out=w1155:errorcluster)
        n541 = property on="Laser pulses" class="DigNum (strict)"("Value"=w1137) -> ()  [unwired: 2 in, 2 out]
        n542 = property on="Trigger pulses" class="DigNum (strict)"("Value"=w1144) -> ()  [unwired: 2 in, 2 out]
        n543 = Merge Errors(w1165, w1155, w1159) -> (w1190:errorcluster)
      }
      event "Frame rate": Value Change {
        (unwired) 0.05 ("x")
        (unwired) 0.05 ("y")
        # "Trigger"
        # "473 nm"
        # "561 nm"
        n544 = event-data() -> ()  [unwired: 1 in, 1 out]
        n545 = local read "Duty Cycle camera"() -> (w1247:dbl)
        n546 = call <vilib>:"DAQmx Stop Task.vi"("task/channels in"=w1244, "error in"=w1243) -> ("task out"=w1270:refnum<k21>, "error out"=w1269:errorcluster)  [unwired: 12 in]
        n547 = local read "Frame rate"() -> (w1228:dbl)
        n548 = property on="Continous ill" class="Bool (strict)"() -> ("Value"=w1235:bool)  [unwired: 2 in, 2 out]
        n549 = property on="Frequency 1" class="Knob (strict)"() -> ("Value"=w1233:dbl)  [unwired: 2 in, 2 out]
        n550 = call <vilib>:"DAQmx Stop Task.vi"("task/channels in"=w1283, "error in"=w1281) -> ("task out"=w1275:refnum<k21>, "error out"=w1274:errorcluster)  [unwired: 12 in]
        n551 = call <vilib>:"DAQmx Stop Task.vi"("task/channels in"=w1246, "error in"=w1245) -> ("task out"=w1273:refnum<k21>, "error out"=w1272:errorcluster)  [unwired: 12 in]
        n552 = local read "First frame\ndelay (ms)"() -> (w1277:dbl)
        n553 = property on="Frame rate 2" class="Knob (strict)"("Value"=w1228) -> ()  [unwired: 2 in, 2 out]
        n554 = property on="Duty Cycle camera 2" class="Knob (strict)"("Value"=w1247) -> ()  [unwired: 2 in, 2 out]
        n555 = Divide(x=w1277, y=1000) -> (x/y=w1240:dbl)
        n556 = property class="DAQmx Channel"(reference=w1275, error in=w1274, "CO.Pulse.Freq"=w1228, "CO.Pulse.DutyCyc"=w1247) -> (reference out=w1264:refnum<k21>, error out=w1262:errorcluster)
        n557 = Multiply(x=w1228, y=w1240) -> (x*y=w1279:dbl)
        n558 = To Long Integer(number=w1279) -> (32bit integer=w1259:i32)
        n559 = Reciprocal(x=w1228) -> (1/x=w1278:dbl)
        n560 = Multiply(x=w1259, y=w1278) -> (x*y=w1265:dbl)
        n561 = property on="Initial calculated\ndelay (frames)" class="DigNum (strict)"("Value"=w1279) -> ()  [unwired: 2 in, 2 out]
        n562 = local read "Illuminated Frames"() -> (w1234:i32)
        n563 = local read "Finishing frames"() -> (w1260:i32)
        n564 = Multiply(x=w1265, y=1000) -> (x*y=w1271:dbl)
        n565 = property on="Laser delay (ms)" class="DigNum (strict)"("Value"=w1271) -> ()  [unwired: 2 in, 2 out]
        n566 = Divide(x=w1234, y=2) -> (x/y=w1249:dbl)
        n567 = To Long Integer(number=w1249) -> (32bit integer=w1230:i32)
        n568 = case shown="False" w1235 {
          tunnel: [w1291 w1311] -> w1232
          tunnel: [w1284 1] -> w1229
          tunnel: [w1289 w1312] -> w1227
          tunnel: [w1292 0.0] -> w1226
          tunnel: w1228 -> [w1287 w1309]
          tunnel: w1233 -> [w1288 _]
          tunnel: w1230 -> [w1286 _]
          tunnel: w1234 -> [w1285 w1308]
          frame False {
            n569 = property on="Pulsed" class="Bool (strict)"() -> ("Value"=w1290:bool)  [unwired: 2 in, 2 out]
            n570 = property on="Duty Cycle 1\npreset" class="Knob (strict)"() -> ("Value"=w1289:dbl)  [unwired: 2 in, 2 out]
            n571 = case shown="False" w1290 {
              tunnel: w1289 -> [_ _]
              tunnel: [w1297 0.0] -> w1292
              tunnel: [w1296 w1306] -> w1291
              tunnel: w1288 -> [w1295 _]
              tunnel: w1287 -> [w1294 w1306]
              tunnel: w1286 -> [w1293 _]
              tunnel: w1285 -> [_ w1305]
              tunnel: [w1293 w1305] -> w1284
              frame False {
                n572 = property on="Link rates" class="Bool (strict)"() -> ("Value"=w1300:bool)  [unwired: 2 in, 2 out]
                n573 = case shown="False" w1300 {
                  tunnel: [w1301 w1303] -> w1296
                  tunnel: w1295 -> [w1301 _]
                  tunnel: w1294 -> [_ w1302]
                  frame False {
                  }
                  frame True {
                    n574 = Divide(x=w1302, y=2) -> (x/y=w1303:dbl)
                    n575 = property on="Frequency 1" class="Knob (strict)"("Value"=w1303) -> ()  [unwired: 2 in, 2 out]
                  }
                }
                n576 = Multiply(x=w1296, y=2) -> (x*y=w1299:dbl)
                n577 = Reciprocal(x=w1299) -> (1/x=w1297:dbl)
              }
              frame True {
              }
            }
            n578 = property on="Duty Cycle 1" class="Knob (strict)"("Value"=w1289) -> ()  [unwired: 2 in, 2 out]
          }
          frame True {
            w1312 = 0.9999 ("x")
            n579 = Reciprocal(x=w1309) -> (1/x=w1315:dbl)
            n580 = Multiply(x=w1315, y=w1308) -> (x*y=w1313:dbl)
            n581 = property on="Duty Cycle 1" class="Knob (strict)"("Value"=w1312) -> ()  [unwired: 2 in, 2 out]
            n582 = Divide(x=w1312, y=w1313) -> (x/y=w1311:dbl)
            n583 = property on="Frequency 1" class="Knob (strict)"("Value"=w1311) -> ()  [unwired: 2 in, 2 out]
          }
        }
        n584 = Add(x=w1265, y=w1226) -> (x+y=w1266:dbl)
        n585 = Multiply(x=w1226, y=1000) -> (x*y=w1267:dbl)
        n586 = property class="DAQmx Channel"(reference=w1273, error in=w1272, "CO.Pulse.Freq"=w1232, "CO.Pulse.DutyCyc"=w1227, "CO.Pulse.Freq.InitialDelay"=w1265) -> (reference out=w1254:refnum<k21>, error out=w1252:errorcluster)
        n587 = property class="DAQmx Channel"(reference=w1270, error in=w1269, "CO.Pulse.Freq"=w1232, "CO.Pulse.DutyCyc"=w1227, "CO.Pulse.Freq.InitialDelay"=w1266) -> (reference out=w1258:refnum<k21>, error out=w1256:errorcluster)
        n588 = property on="Frequency 2" class="Knob (strict)"("Value"=w1232) -> ()  [unwired: 2 in, 2 out]
        n589 = property on="Initial delay\n473 nm (ms)" class="DigNum (strict)"("Value"=w1267) -> ()  [unwired: 2 in, 2 out]
        n590 = property on="Duty Cycle 2" class="Knob (strict)"("Value"=w1227) -> ()  [unwired: 2 in, 2 out]
        n591 = Add(x=w1234, y=w1259) -> (x+y=w1248:i32)
        n592 = Add(x=w1260, y=w1248) -> (x+y=w1231:i32)
        n593 = property class="DAQmx Timing"(reference=w1264, error in=w1262, "SampQuant.SampPerChan"=w1231) -> (reference out=w1263:refnum<k21>, error out=w1261:errorcluster)
        n594 = property on="delay\ncompensation" class="DigNum (strict)"() -> ("Value"=w1225:dbl)  [unwired: 2 in, 2 out]
        n595 = property on="Trigger pulses" class="DigNum (strict)"("Value"=w1231) -> ()  [unwired: 2 in, 2 out]
        n596 = property class="DAQmx Timing"(reference=w1254, error in=w1252, "SampQuant.SampPerChan"=w1229) -> (reference out=w1253:refnum<k21>, error out=w1251:errorcluster)
        n597 = Multiply(x=w1225, y=w1228) -> (x*y=w1236:dbl)
        n598 = Subtract(x=w1240, y=w1225) -> (x-y=w1241:dbl)
        n599 = property class="DAQmx Timing"(reference=w1258, error in=w1256, "SampQuant.SampPerChan"=w1229) -> (reference out=w1257:refnum<k21>, error out=w1255:errorcluster)
        n600 = property on="Laser pulses" class="DigNum (strict)"("Value"=w1229) -> ()  [unwired: 2 in, 2 out]
        n601 = To Long Integer(number=w1236) -> (32bit integer=w1237:i32)
        n602 = Multiply(x=w1228, y=w1241) -> (x*y=w1242:dbl)
        n603 = Subtract(x=w1231, y=w1237) -> (x-y=w1238:i32)
        n604 = To Long Integer(number=w1242) -> (32bit integer=w1239:i32)
        n605 = property on="Frames to acquire" class="DigNum (strict)"("Value"=w1238) -> ()  [unwired: 2 in, 2 out]
        n606 = property on="Initial frames" class="DigNum (strict)"("Value"=w1239) -> ()  [unwired: 2 in, 2 out]
        n607 = Merge Errors(w1261, w1251, w1255) -> (w1282:errorcluster)
      }
      event "Frame rate 2": Value Change {
        # "Trigger"
        # "473 nm"
        # "561 nm"
        n608 = event-data() -> ()  [unwired: 1 in, 1 out]
        n609 = local read "Duty Cycle camera 2"() -> (w1325:dbl)
        n610 = call <vilib>:"DAQmx Stop Task.vi"("task/channels in"=w1345, "error in"=w1344) -> ("task out"=w1339:refnum<k21>, "error out"=w1338:errorcluster)  [unwired: 12 in]
        n611 = call <vilib>:"DAQmx Stop Task.vi"("task/channels in"=w1350, "error in"=w1346) -> ("task out"=w1343:refnum<k21>, "error out"=w1342:errorcluster)  [unwired: 12 in]
        n612 = call <vilib>:"DAQmx Stop Task.vi"("task/channels in"=w1349, "error in"=w1347) -> ("task out"=w1341:refnum<k21>, "error out"=w1340:errorcluster)  [unwired: 12 in]
        n613 = local read "Frame rate 2"() -> (w1316:dbl)
        n614 = local read "Duty Cycle 2"() -> (w1321:dbl)
        n615 = property class="DAQmx Channel"(reference=w1343, error in=w1342, "CO.Pulse.Freq"=w1316, "CO.Pulse.DutyCyc"=w1325) -> (reference out=w1333:refnum<k21>, error out=w1326:errorcluster)
        n616 = case shown="True" "Link rates 2" {
          tunnel: w1316 -> [_ w1354]
          tunnel: [w1351 w1352] -> w1320
          frame False {
            n617 = local read "Frequency 2"() -> (w1351:dbl)
          }
          frame True {
            n618 = Divide(x=w1354, y=2) -> (x/y=w1352:dbl)
            n619 = property on="Frequency 2" class="Knob (strict)"("Value"=w1352) -> ()  [unwired: 2 in, 2 out]
          }
        }
        n620 = Multiply(x=w1320, y=2) -> (x*y=w1336:dbl)
        n621 = Reciprocal(x=w1336) -> (1/x=w1329:dbl)
        n622 = Multiply(x=w1329, y=1000) -> (x*y=w1334:dbl)
        n623 = property class="DAQmx Channel"(reference=w1341, error in=w1340, "CO.Pulse.Freq"=w1320, "CO.Pulse.DutyCyc"=w1321, "CO.Pulse.Freq.InitialDelay"=0.0) -> (reference out=w1332:refnum<k21>, error out=w1323:errorcluster)
        n624 = property class="DAQmx Channel"(reference=w1339, error in=w1338, "CO.Pulse.Freq"=w1320, "CO.Pulse.DutyCyc"=w1321, "CO.Pulse.Freq.InitialDelay"=w1329) -> (reference out=w1331:refnum<k21>, error out=w1330:errorcluster)
        n625 = property on="initial delay\n473 nm (ms) 2" class="DigNum (strict)"("Value"=w1334) -> ()  [unwired: 2 in, 2 out]
        n626 = property on="Frame rate" class="Knob (strict)"(error in=w1326, "Value"=w1316) -> (error out=w1327:errorcluster)  [unwired: 1 in, 1 out]
        n627 = property on="Frequency 1" class="Knob (strict)"(error in=w1323, "Value"=w1320) -> (error out=w1324:errorcluster)  [unwired: 1 in, 1 out]
        n628 = property on="Duty Cycle 1" class="Knob (strict)"(error in=w1324, "Value"=w1321) -> (error out=w1322:errorcluster)  [unwired: 1 in, 1 out]
        n629 = property on="Duty Cycle camera" class="Knob (strict)"(error in=w1327, "Value"=w1325) -> (error out=w1318:errorcluster)  [unwired: 1 in, 1 out]
        n630 = property on="Frame Rate display" class="DigNum (strict)"(error in=w1318, "Value"=w1316) -> (error out=w1317:errorcluster)  [unwired: 1 in, 1 out]
        n631 = Merge Errors(w1317, w1322, w1330) -> (w1348:errorcluster)
      }
      event "Frequency 2": Value Change {
        # "Trigger"
        # "473 nm"
        # "561 nm"
        n632 = event-data() -> ()  [unwired: 1 in, 1 out]
        n633 = local read "Frequency 2"() -> (w1355:dbl)
        n634 = call <vilib>:"DAQmx Stop Task.vi"("task/channels in"=w1383, "error in"=w1382) -> ("task out"=w1377:refnum<k21>, "error out"=w1376:errorcluster)  [unwired: 12 in]
        n635 = local read "Duty Cycle camera 2"() -> (w1361:dbl)
        n636 = call <vilib>:"DAQmx Stop Task.vi"("task/channels in"=w1388, "error in"=w1384) -> ("task out"=w1381:refnum<k21>, "error out"=w1380:errorcluster)  [unwired: 12 in]
        n637 = call <vilib>:"DAQmx Stop Task.vi"("task/channels in"=w1387, "error in"=w1385) -> ("task out"=w1379:refnum<k21>, "error out"=w1378:errorcluster)  [unwired: 12 in]
        n638 = Multiply(x=w1355, y=2) -> (x*y=w1374:dbl)
        n639 = local read "Duty Cycle 2"() -> (w1357:dbl)
        n640 = Reciprocal(x=w1374) -> (1/x=w1366:dbl)
        n641 = Multiply(x=w1366, y=1000) -> (x*y=w1372:dbl)
        n642 = property class="DAQmx Channel"(reference=w1379, error in=w1378, "CO.Pulse.Freq"=w1355, "CO.Pulse.DutyCyc"=w1357, "CO.Pulse.Freq.InitialDelay"=0.0) -> (reference out=w1369:refnum<k21>, error out=w1359:errorcluster)
        n643 = property class="DAQmx Channel"(reference=w1377, error in=w1376, "CO.Pulse.Freq"=w1355, "CO.Pulse.DutyCyc"=w1357, "CO.Pulse.Freq.InitialDelay"=w1366) -> (reference out=w1368:refnum<k21>, error out=w1367:errorcluster)
        n644 = property on="Link rates 2" class="Bool (strict)"() -> ("Value"=w1371:bool)  [unwired: 2 in, 2 out]
        n645 = property on="initial delay\n473 nm (ms) 2" class="DigNum (strict)"("Value"=w1372) -> ()  [unwired: 2 in, 2 out]
        n646 = case shown="True" w1371 {
          tunnel: w1355 -> [_ w1392]
          tunnel: [w1389 w1390] -> w1356
          frame False {
            n647 = local read "Frame rate 2"() -> (w1389:dbl)
          }
          frame True {
            n648 = Multiply(x=w1392, y=2) -> (x*y=w1390:dbl)
            n649 = property on="Frame rate 2" class="Knob (strict)"("Value"=w1390) -> ()  [unwired: 2 in, 2 out]
          }
        }
        n650 = property class="DAQmx Channel"(reference=w1381, error in=w1380, "CO.Pulse.Freq"=w1356, "CO.Pulse.DutyCyc"=w1361) -> (reference out=w1370:refnum<k21>, error out=w1363:errorcluster)
        n651 = property on="Frame rate" class="Knob (strict)"(error in=w1363, "Value"=w1356) -> (error out=w1364:errorcluster)  [unwired: 1 in, 1 out]
        n652 = property on="Frequency 1" class="Knob (strict)"(error in=w1359, "Value"=w1355) -> (error out=w1360:errorcluster)  [unwired: 1 in, 1 out]
        n653 = property on="Duty Cycle 1" class="Knob (strict)"(error in=w1360, "Value"=w1357) -> (error out=w1358:errorcluster)  [unwired: 1 in, 1 out]
        n654 = property on="Duty Cycle camera" class="Knob (strict)"(error in=w1364, "Value"=w1361) -> (error out=w1362:errorcluster)  [unwired: 1 in, 1 out]
        n655 = Merge Errors(w1362, w1358, w1367) -> (w1386:errorcluster)
      }
      event "AFLEX": Value Change {
        n656 = event-data() -> ()  [unwired: 1 in, 1 out]
        n657 = call <vilib>:"DAQmx Stop Task.vi"("task/channels in"=w1404, "error in"=w1403) -> ("task out"=w1398:refnum<k21>, "error out"=w1397:errorcluster)  [unwired: 12 in]
        n658 = call <vilib>:"DAQmx Stop Task.vi"("task/channels in"=w1409, "error in"=w1405) -> ("task out"=w1402:refnum<k21>, "error out"=w1401:errorcluster)  [unwired: 12 in]
        n659 = call <vilib>:"DAQmx Stop Task.vi"("task/channels in"=w1408, "error in"=w1406) -> ("task out"=w1400:refnum<k21>, "error out"=w1399:errorcluster)  [unwired: 12 in]
        n660 = case shown="False" "AFLEX" {
          selector: "AFLEX" -> [w1439 _]
          tunnel: [w1442 w1513] -> w1407
          tunnel: w1402 -> [w1449 w1512]
          tunnel: w1401 -> [w1444 w1496]
          tunnel: w1400 -> [w1426 w1510]
          tunnel: w1399 -> [w1412 w1483]
          tunnel: w1398 -> [w1431 w1509]
          tunnel: w1397 -> [w1436 w1480]
          tunnel: [w1448 w1490] -> w1396
          tunnel: [w1430 w1473] -> w1393
          tunnel: [w1425 w1477] -> w1395
          frame False {
            w1432 = 10150 items=["Analog Edge"=10099, "Digital Edge"=10150, "Digital Pattern"=10398, "Analog Window"=10103, "None"=10230] ("Start.TrigType")
            w1433 = 10150 items=["Analog Edge"=10099, "Digital Edge"=10150, "Digital Pattern"=10398, "Analog Window"=10103, "None"=10230] ("Start.TrigType")
            w1415 = T2."Disabled and Grayed Out" ("Disabled")
            w1452 = 10230 items=["Analog Edge"=10099, "Digital Edge"=10150, "Digital Pattern"=10398, "Analog Window"=10103, "None"=10230] ("Start.TrigType")
            w1455 = 10123 items=["Finite Samples"=10178, "Continuous Samples"=10123, "Hardware Timed Single Point"=12522] ("SampQuant.SampMode")
            n661 = property on="Power control" class="Bool (strict)"() -> ("Value"=w1414:bool)  [unwired: 2 in, 2 out]
            n662 = property on="Link rates 2" class="Bool (strict)"(error in=w1444, "DisabledEnum"=T2."Disabled and Grayed Out" ("Disabled")) -> (error out=w1434:errorcluster)  [unwired: 1 in, 1 out]
            n663 = property on="ALL LASERS 2" class="Bool (strict)"(error in=w1436, "Value"=w1439) -> (error out=w1440:errorcluster)  [unwired: 1 in, 1 out]
            n664 = case shown="True" w1414 {
              tunnel: w1415 -> [w1456 _]
              tunnel: [w1456 T2."Enabled" ("Disabled")] -> w1413
              frame False {
              }
              frame True {
              }
            }
            n665 = property on="561 nm 2" class="Bool (strict)"(error in=w1440, "Value"=w1439) -> (error out=w1441:errorcluster)  [unwired: 1 in, 1 out]
            n666 = property on="Duty Cycle \nDenominator" class="DigNum (strict)"(error in=w1412) -> (error out=w1411:errorcluster, "Value"=w1410:dbl)  [unwired: 1 in, 1 out]
            n667 = property on="473 nm 2" class="Bool (strict)"(error in=w1441, "Value"=w1439) -> (error out=w1438:errorcluster)  [unwired: 1 in, 1 out]
            n668 = property on="Duty Cycle \nDenominator 2" class="DigNum (strict)"(error in=w1411, "Value"=w1410, "DisabledEnum"=w1413) -> (error out=w1423:errorcluster)  [unwired: 1 in, 1 out]
            n669 = property on="Frame rate 2" class="Knob (strict)"() -> ("Value"=w1447:dbl)  [unwired: 2 in, 2 out]
            n670 = property on="Duty Cycle camera 2" class="Knob (strict)"() -> ("Value"=w1446:dbl)  [unwired: 2 in, 2 out]
            n671 = property on="Duty Cycle 2" class="Knob (strict)"(error in=w1438, "DisabledEnum"=w1415) -> (error out=w1437:errorcluster, "Value"=w1416:dbl)  [unwired: 1 in, 1 out]
            n672 = Greater?(x=w1416, y=0.5) -> (0:w1417:bool)
            n673 = property class="DAQmx Channel"(reference=w1449, error in=w1434, "CO.Pulse.Freq"=w1447, "CO.Pulse.DutyCyc"=w1446) -> (reference out=w1454:refnum<k21>, error out=w1453:errorcluster)
            n674 = property on="Frequency 2" class="Knob (strict)"(error in=w1437, "DisabledEnum"=w1415) -> (error out=w1435:errorcluster)  [unwired: 1 in, 1 out]
            n675 = Select(t="WARNING! Laser DC > 0.5\nAFLEX not possible", s=w1417, f="AFLEX conditions\nnormal") -> (s? t:f=w1418:string)
            n676 = property on="HALF DC 2" class="Bool (strict)"(error in=w1435, "DisabledEnum"=w1413) -> (error out=w1429:errorcluster)  [unwired: 1 in, 1 out]
            n677 = property on="AFLEX warning 2" class="Bool (strict)"(error in=w1423, "Caption.Text"=w1418, "Value"=w1417, "DisabledEnum"=w1415) -> (error out=w1422:errorcluster)  [unwired: 1 in, 1 out]
            n678 = property class="DAQmx Timing"(reference=w1454, error in=w1453, "Sample Quantity:Sample Mode"=w1455) -> (reference out=w1451:refnum<k21>, error out=w1450:errorcluster)
            n679 = property on="trigger ready source" class="DAQmxName"() -> ("Value"=w1427:string)  [unwired: 2 in, 2 out]
            n680 = property class="DAQmx Trigger"(reference=w1426, error in=w1422, "Start:Trigger Type"=w1433, "Start.DigEdge.Src"=w1427) -> (reference out=w1425:refnum<k21>, error out=w1424:errorcluster)
            n681 = property class="DAQmx Trigger"(reference=w1451, error in=w1450, "Start:Trigger Type"=w1452) -> (reference out=w1448:refnum<k21>, error out=w1443:errorcluster)
            n682 = property class="DAQmx Trigger"(reference=w1431, error in=w1429, "Start:Trigger Type"=w1432, "Start.DigEdge.Src"=w1427) -> (reference out=w1430:refnum<k21>, error out=w1428:errorcluster)
            n683 = Merge Errors(w1443, w1424, w1428) -> (w1442:errorcluster)
          }
          frame True {
            w1468 = tag "/Dev1/Ctr0InternalOutput" ("Start.DigEdge.Src")
            w1469 = 10150 items=["Analog Edge"=10099, "Digital Edge"=10150, "Digital Pattern"=10398, "Analog Window"=10103, "None"=10230] ("Start.TrigType")
            w1470 = 10150 items=["Analog Edge"=10099, "Digital Edge"=10150, "Digital Pattern"=10398, "Analog Window"=10103, "None"=10230] ("Start.TrigType")
            w1458 = T2."Enabled" ("Disabled")
            w1465 = T2."Enabled" ("Disabled")
            w1484 = 10214 items=["High"=10192, "Low"=10214] ("CO.Pulse.IdleState")
            w1485 = 10214 items=["High"=10192, "Low"=10214] ("CO.Pulse.IdleState")
            w1494 = 10230 items=["Analog Edge"=10099, "Digital Edge"=10150, "Digital Pattern"=10398, "Analog Window"=10103, "None"=10230] ("Start.TrigType")
            w1489 = 10123 items=["Finite Samples"=10178, "Continuous Samples"=10123, "Hardware Timed Single Point"=12522] ("SampQuant.SampMode")
            # "Trigger"
            # "473 nm"
            # "561 nm"
            n684 = property on="Link rates 2" class="Bool (strict)"(error in=w1496, "DisabledEnum"=T2."Enabled" ("Disabled")) -> (error out=w1495:errorcluster)  [unwired: 1 in, 1 out]
            n685 = property on="Frequency 2" class="Knob (strict)"(error in=w1480, "DisabledEnum"=w1458) -> (error out=w1481:errorcluster)  [unwired: 1 in, 1 out]
            n686 = property on="HALF DC 2" class="Bool (strict)"(error in=w1483, "DisabledEnum"=w1465) -> (error out=w1467:errorcluster)  [unwired: 1 in, 1 out]
            n687 = property on="Duty Cycle 2" class="Knob (strict)"(error in=w1481, "DisabledEnum"=w1458) -> (error out=w1479:errorcluster)  [unwired: 1 in, 1 out]
            n688 = property on="Duty Cycle \nDenominator 2" class="DigNum (strict)"(error in=w1467, "DisabledEnum"=w1465) -> (error out=w1466:errorcluster)  [unwired: 1 in, 1 out]
            n689 = Greater?(x="Duty Cycle 2", y=0.5) -> (0:w1460:bool)
            n690 = Select(t="WARNING! Laser DC > 0.5\nAFLEX not possible", s=w1460, f="AFLEX conditions\nnormal") -> (s? t:f=w1461:string)
            n691 = local read "Duty Cycle camera 2"() -> (w1511:dbl)
            n692 = local read "Frame rate 2"() -> (w1482:dbl)
            n693 = property on="AFLEX warning 2" class="Bool (strict)"("Caption.Text"=w1461, "Value"=w1460, "DisabledEnum"=w1458) -> ()  [unwired: 2 in, 2 out]
            n694 = property class="DAQmx Channel"(reference=w1512, error in=w1495, "CO.Pulse.Freq"=w1482, "CO.Pulse.DutyCyc"=w1511) -> (reference out=w1505:refnum<k21>, error out=w1504:errorcluster)
            n695 = property on="Link rates 2" class="Bool (strict)"() -> ("Value"=w1499:bool)  [unwired: 2 in, 2 out]
            n696 = case shown="True" w1499 {
              tunnel: w1482 -> [_ w1517]
              tunnel: ["Frequency 2" w1515] -> w1498
              frame False {
              }
              frame True {
                n697 = Divide(x=w1517, y=2) -> (x/y=w1515:dbl)
                n698 = property on="Frequency 2" class="Knob (strict)"("Value"=w1515) -> ()  [unwired: 2 in, 2 out]
              }
            }
            n699 = Multiply(x=w1498, y=2) -> (x*y=w1507:dbl)
            n700 = Reciprocal(x=w1507) -> (1/x=w1487:dbl)
            n701 = property class="DAQmx Channel"(reference=w1510, error in=w1466, "CO.Pulse.Freq"=w1498, "CO.Pulse.DutyCyc"="Duty Cycle 2", "CO.Pulse.Freq.InitialDelay"=0.0, "CO.Pulse.IdleState"=w1485) -> (reference out=w1501:refnum<k21>, error out=w1500:errorcluster)
            n702 = property class="DAQmx Channel"(reference=w1509, error in=w1479, "CO.Pulse.Freq"=w1498, "CO.Pulse.DutyCyc"="Duty Cycle 2", "CO.Pulse.Freq.InitialDelay"=w1487, "CO.Pulse.IdleState"=w1484) -> (reference out=w1503:refnum<k21>, error out=w1502:errorcluster)
            n703 = Multiply(x=w1487, y=1000) -> (x*y=→"initial delay\n473 nm (ms) 2":dbl)
            n704 = property class="DAQmx Timing"(reference=w1501, error in=w1500, "SampQuant.SampMode"=w1489) -> (reference out=w1478:refnum<k21>, error out=w1476:errorcluster)
            n705 = property class="DAQmx Timing"(reference=w1503, error in=w1502, "SampQuant.SampMode"=w1489) -> (reference out=w1474:refnum<k21>, error out=w1472:errorcluster)
            n706 = property class="DAQmx Timing"(reference=w1505, error in=w1504, "SampQuant.SampMode"=w1489) -> (reference out=w1491:refnum<k21>, error out=w1493:errorcluster)
            n707 = property class="DAQmx Trigger"(reference=w1478, error in=w1476, "Start:Trigger Type"=w1470, "Start.DigEdge.Src"=w1468) -> (reference out=w1477:refnum<k21>, error out=w1475:errorcluster)
            n708 = property class="DAQmx Trigger"(reference=w1474, error in=w1472, "Start:Trigger Type"=w1469, "Start.DigEdge.Src"=w1468) -> (reference out=w1473:refnum<k21>, error out=w1471:errorcluster)
            n709 = property class="DAQmx Trigger"(reference=w1491, error in=w1493, "Start:Trigger Type"=w1494) -> (reference out=w1490:refnum<k21>, error out=w1492:errorcluster)
            n710 = Merge Errors(w1492, w1475, w1471) -> (w1513:errorcluster)
            "Duty Cycle 2\nmemory" <- "Duty Cycle 2"
          }
        }
      }
      event "Frequency 1": Value Change {
        (unwired) 0.05 ("x")
        (unwired) 0.05 ("y")
        # "Trigger"
        # "473 nm"
        # "561 nm"
        n711 = event-data() -> ()  [unwired: 1 in, 1 out]
        n712 = local read "Duty Cycle camera"() -> (w1533:dbl)
        n713 = call <vilib>:"DAQmx Stop Task.vi"("task/channels in"=w1574, "error in"=w1570) -> ("task out"=w1562:refnum<k21>, "error out"=w1561:errorcluster)  [unwired: 12 in]
        n714 = call <vilib>:"DAQmx Stop Task.vi"("task/channels in"=w1573, "error in"=w1571) -> ("task out"=w1560:refnum<k21>, "error out"=w1559:errorcluster)  [unwired: 12 in]
        n715 = call <vilib>:"DAQmx Stop Task.vi"("task/channels in"=w1569, "error in"=w1568) -> ("task out"=w1557:refnum<k21>, "error out"=w1556:errorcluster)  [unwired: 12 in]
        n716 = local read "Duty Cycle 1"() -> (w1532:dbl)
        n717 = local read "Frequency 1"() -> (w1534:dbl)
        n718 = local read "First frame\ndelay (ms)"() -> (w1564:dbl)
        n719 = property on="Duty Cycle camera 2" class="Knob (strict)"("Value"=w1533) -> ()  [unwired: 2 in, 2 out]
        n720 = property on="Duty Cycle 2" class="Knob (strict)"("Value"=w1532) -> ()  [unwired: 2 in, 2 out]
        n721 = Divide(x=w1564, y=1000) -> (x/y=w1529:dbl)
        n722 = property on="Frequency 2" class="Knob (strict)"("Value"=w1534) -> ()  [unwired: 2 in, 2 out]
        n723 = property on="Link rates" class="Bool (strict)"() -> ("Value"=w1522:bool)  [unwired: 2 in, 2 out]
        n724 = property on="Pulsed" class="Bool (strict)"() -> ("Value"=w1519:bool)  [unwired: 2 in, 2 out]
        n725 = case shown="False" w1519 {
          tunnel: w1534 -> [w1582 _]
          tunnel: [w1580 0.0] -> w1520
          frame False {
            n726 = Multiply(x=w1582, y=2) -> (x*y=w1581:dbl)
            n727 = Reciprocal(x=w1581) -> (1/x=w1580:dbl)
          }
          frame True {
          }
        }
        n728 = Multiply(x=w1520, y=1000) -> (x*y=w1554:dbl)
        n729 = property on="Initial delay\n473 nm (ms)" class="DigNum (strict)"("Value"=w1554) -> ()  [unwired: 2 in, 2 out]
        n730 = local read "Illuminated Frames"() -> (w1535:i32)
        n731 = Or(x=w1522, y=w1519) -> (x .or. y?=w1521:bool)
        n732 = local read "Finishing frames"() -> (w1547:i32)
        n733 = case shown="True" w1521 {
          tunnel: [w1585 w1586] -> w1524
          tunnel: w1534 -> [_ w1588]
          frame False {
            n734 = local read "Frame rate"() -> (w1585:dbl)
          }
          frame True {
            n735 = Multiply(x=w1588, y=2) -> (x*y=w1586:dbl)
            n736 = property on="Frame rate" class="Knob (strict)"("Value"=w1586) -> ()  [unwired: 2 in, 2 out]
          }
        }
        n737 = property class="DAQmx Channel"(reference=w1562, error in=w1561, "CO.Pulse.Freq"=w1524, "CO.Pulse.DutyCyc"=w1533) -> (reference out=w1551:refnum<k21>, error out=w1549:errorcluster)
        n738 = property on="Frame rate 2" class="Knob (strict)"("Value"=w1524) -> ()  [unwired: 2 in, 2 out]
        n739 = Multiply(x=w1524, y=w1529) -> (x*y=w1566:dbl)
        n740 = To Long Integer(number=w1566) -> (32bit integer=w1546:i32)
        n741 = Reciprocal(x=w1524) -> (1/x=w1565:dbl)
        n742 = Multiply(x=w1546, y=w1565) -> (x*y=w1552:dbl)
        n743 = Add(x=w1552, y=w1520) -> (x+y=w1553:dbl)
        n744 = property class="DAQmx Channel"(reference=w1560, error in=w1559, "CO.Pulse.Freq"=w1534, "CO.Pulse.DutyCyc"=w1532, "CO.Pulse.Freq.InitialDelay"=w1552) -> (reference out=w1541:refnum<k21>, error out=w1539:errorcluster)
        n745 = property class="DAQmx Channel"(reference=w1557, error in=w1556, "CO.Pulse.Freq"=w1534, "CO.Pulse.DutyCyc"=w1532, "CO.Pulse.Freq.InitialDelay"=w1553) -> (reference out=w1545:refnum<k21>, error out=w1543:errorcluster)
        n746 = property on="Initial calculated\ndelay (frames)" class="DigNum (strict)"("Value"=w1566) -> ()  [unwired: 2 in, 2 out]
        n747 = Multiply(x=w1552, y=1000) -> (x*y=w1558:dbl)
        n748 = property on="Laser delay (ms)" class="DigNum (strict)"("Value"=w1558) -> ()  [unwired: 2 in, 2 out]
        n749 = Add(x=w1535, y=w1546) -> (x+y=w1537:i32)
        n750 = Add(x=w1547, y=w1537) -> (x+y=w1523:i32)
        n751 = case shown="True" w1519 {
          tunnel: [w1576 w1579] -> w1536
          tunnel: w1535 -> [w1575 w1579]
          frame False {
            n752 = Divide(x=w1575, y=2) -> (x/y=w1577:dbl)
            n753 = To Long Integer(number=w1577) -> (32bit integer=w1576:i32)
          }
          frame True {
          }
        }
        n754 = property on="delay\ncompensation" class="DigNum (strict)"() -> ("Value"=w1518:dbl)  [unwired: 2 in, 2 out]
        n755 = property class="DAQmx Timing"(reference=w1551, error in=w1549, "SampQuant.SampPerChan"=w1523) -> (reference out=w1550:refnum<k21>, error out=w1548:errorcluster)
        n756 = Multiply(x=w1518, y=w1524) -> (x*y=w1525:dbl)
        n757 = property on="Trigger pulses" class="DigNum (strict)"("Value"=w1523) -> ()  [unwired: 2 in, 2 out]
        n758 = property class="DAQmx Timing"(reference=w1541, error in=w1539, "SampQuant.SampPerChan"=w1536) -> (reference out=w1540:refnum<k21>, error out=w1538:errorcluster)
        n759 = property class="DAQmx Timing"(reference=w1545, error in=w1543, "SampQuant.SampPerChan"=w1536) -> (reference out=w1544:refnum<k21>, error out=w1542:errorcluster)
        n760 = To Long Integer(number=w1525) -> (32bit integer=w1526:i32)
        n761 = Subtract(x=w1529, y=w1518) -> (x-y=w1530:dbl)
        n762 = property on="Laser pulses" class="DigNum (strict)"("Value"=w1536) -> ()  [unwired: 2 in, 2 out]
        n763 = Multiply(x=w1524, y=w1530) -> (x*y=w1531:dbl)
        n764 = Subtract(x=w1523, y=w1526) -> (x-y=w1527:i32)
        n765 = To Long Integer(number=w1531) -> (32bit integer=w1528:i32)
        n766 = property on="Frames to acquire" class="DigNum (strict)"("Value"=w1527) -> ()  [unwired: 2 in, 2 out]
        n767 = property on="Initial frames" class="DigNum (strict)"("Value"=w1528) -> ()  [unwired: 2 in, 2 out]
        n768 = Merge Errors(w1548, w1538, w1542) -> (w1572:errorcluster)
      }
      event "Duty Cycle 1": Value Change {
        (unwired) 0.05 ("x")
        (unwired) 0.05 ("y")
        # "Trigger"
        # "473 nm"
        # "561 nm"
        n769 = event-data() -> ()  [unwired: 1 in, 1 out]
        n770 = property on="HALF DC" class="Bool (strict)"() -> ("Value"=w1591:bool)  [unwired: 2 in, 2 out]
        n771 = local read "Duty Cycle camera"() -> (w1613:dbl)
        n772 = call <vilib>:"DAQmx Stop Task.vi"("task/channels in"=w1653, "error in"=w1649) -> ("task out"=w1641:refnum<k21>, "error out"=w1640:errorcluster)  [unwired: 12 in]
        n773 = call <vilib>:"DAQmx Stop Task.vi"("task/channels in"=w1648, "error in"=w1647) -> ("task out"=w1636:refnum<k21>, "error out"=w1635:errorcluster)  [unwired: 12 in]
        n774 = local read "Frame rate"() -> (w1598:dbl)
        n775 = call <vilib>:"DAQmx Stop Task.vi"("task/channels in"=w1652, "error in"=w1650) -> ("task out"=w1639:refnum<k21>, "error out"=w1638:errorcluster)  [unwired: 12 in]
        n776 = local read "Duty Cycle 1"() -> (w1590:dbl)
        n777 = case shown="True" w1591 {
          tunnel: w1590 -> [w1654 w1659]
          frame False {
            n778 = property on="Duty Cycle 1\nfull DC" class="Knob (strict)"("Value"=w1654) -> ()  [unwired: 2 in, 2 out]
          }
          frame True {
            n779 = property on="Duty Cycle \nDenominator" class="DigNum (strict)"() -> ("Value"=w1660:dbl)  [unwired: 2 in, 2 out]
            n780 = Multiply(x=w1659, y=w1660) -> (x*y=w1656:dbl)
            n781 = Greater Or Equal?(x=w1656, y=1.0) -> (x >= y?=w1657:bool)
            n782 = case shown="True" w1657 {
              tunnel: w1656 -> [w1661 _]
              tunnel: [w1661 0.9999] -> w1655
              frame False {
              }
              frame True {
              }
            }
            n783 = property on="Duty Cycle 1\nfull DC" class="Knob (strict)"("Value"=w1655) -> ()  [unwired: 2 in, 2 out]
          }
        }
        n784 = Greater?(x=w1590, y=0.5) -> (0:w1592:bool)
        n785 = local read "First frame\ndelay (ms)"() -> (w1643:dbl)
        n786 = property on="Frame rate 2" class="Knob (strict)"("Value"=w1598) -> ()  [unwired: 2 in, 2 out]
        n787 = property on="Duty Cycle 1\npreset" class="Knob (strict)"("Value"=w1590) -> ()  [unwired: 2 in, 2 out]
        n788 = Select(t="WARNING! Laser DC > 0.5\nAFLEX not possible", s=w1592, f="AFLEX conditions\nnormal") -> (s? t:f=w1593:string)
        n789 = property on="Duty Cycle camera 2" class="Knob (strict)"("Value"=w1613) -> ()  [unwired: 2 in, 2 out]
        n790 = property on="AFLEX warning" class="Bool (strict)"("Caption.Text"=w1593, "Value"=w1592) -> ()  [unwired: 2 in, 2 out]
        n791 = property class="DAQmx Channel"(reference=w1641, error in=w1640, "CO.Pulse.Freq"=w1598, "CO.Pulse.DutyCyc"=w1613) -> (reference out=w1630:refnum<k21>, error out=w1628:errorcluster)
        n792 = Divide(x=w1643, y=1000) -> (x/y=w1610:dbl)
        n793 = Multiply(x=w1598, y=w1610) -> (x*y=w1645:dbl)
        n794 = property on="Duty Cycle 2" class="Knob (strict)"("Value"=w1590) -> ()  [unwired: 2 in, 2 out]
        n795 = property on="Pulsed" class="Bool (strict)"() -> ("Value"=w1603:bool)  [unwired: 2 in, 2 out]
        n796 = property on="Frequency 1" class="Knob (strict)"() -> ("Value"=w1604:dbl)  [unwired: 2 in, 2 out]
        n797 = To Long Integer(number=w1645) -> (32bit integer=w1625:i32)
        n798 = Reciprocal(x=w1598) -> (1/x=w1644:dbl)
        n799 = local read "Illuminated Frames"() -> (w1599:i32)
        n800 = Multiply(x=w1625, y=w1644) -> (x*y=w1631:dbl)
        n801 = local read "Finishing frames"() -> (w1626:i32)
        n802 = property on="delay\ncompensation" class="DigNum (strict)"() -> ("Value"=w1589:dbl)  [unwired: 2 in, 2 out]
        n803 = property on="Initial calculated\ndelay (frames)" class="DigNum (strict)"("Value"=w1645) -> ()  [unwired: 2 in, 2 out]
        n804 = Multiply(x=w1631, y=1000) -> (x*y=w1637:dbl)
        n805 = property on="Laser delay (ms)" class="DigNum (strict)"("Value"=w1637) -> ()  [unwired: 2 in, 2 out]
        n806 = Add(x=w1599, y=w1625) -> (x+y=w1614:i32)
        n807 = Divide(x=w1599, y=2) -> (x/y=w1615:dbl)
        n808 = Add(x=w1626, y=w1614) -> (x+y=w1605:i32)
        n809 = property class="DAQmx Timing"(reference=w1630, error in=w1628, "SampQuant.SampPerChan"=w1605) -> (reference out=w1629:refnum<k21>, error out=w1627:errorcluster)
        n810 = To Long Integer(number=w1615) -> (32bit integer=w1601:i32)
        n811 = case shown="False" w1603 {
          tunnel: [w1667 0.0] -> w1602
          tunnel: [w1666 w1676] -> w1597
          tunnel: w1604 -> [w1665 _]
          tunnel: w1598 -> [w1664 w1676]
          tunnel: w1601 -> [w1663 _]
          tunnel: w1599 -> [_ w1675]
          tunnel: [w1663 w1675] -> w1600
          frame False {
            n812 = property on="Link rates" class="Bool (strict)"() -> ("Value"=w1670:bool)  [unwired: 2 in, 2 out]
            n813 = case shown="True" w1670 {
              tunnel: [w1671 w1673] -> w1666
              tunnel: w1665 -> [w1671 _]
              tunnel: w1664 -> [_ w1672]
              frame False {
              }
              frame True {
                n814 = Divide(x=w1672, y=2) -> (x/y=w1673:dbl)
                n815 = property on="Frequency 1" class="Knob (strict)"("Value"=w1673) -> ()  [unwired: 2 in, 2 out]
              }
            }
            n816 = Multiply(x=w1666, y=2) -> (x*y=w1669:dbl)
            n817 = Reciprocal(x=w1669) -> (1/x=w1667:dbl)
          }
          frame True {
          }
        }
        n818 = Add(x=w1631, y=w1602) -> (x+y=w1632:dbl)
        n819 = Multiply(x=w1602, y=1000) -> (x*y=w1633:dbl)
        n820 = property class="DAQmx Channel"(reference=w1639, error in=w1638, "CO.Pulse.Freq"=w1597, "CO.Pulse.DutyCyc"=w1590, "CO.Pulse.Freq.InitialDelay"=w1631) -> (reference out=w1620:refnum<k21>, error out=w1618:errorcluster)
        n821 = property class="DAQmx Channel"(reference=w1636, error in=w1635, "CO.Pulse.Freq"=w1597, "CO.Pulse.DutyCyc"=w1590, "CO.Pulse.Freq.InitialDelay"=w1632) -> (reference out=w1624:refnum<k21>, error out=w1622:errorcluster)
        n822 = property on="Initial delay\n473 nm (ms)" class="DigNum (strict)"("Value"=w1633) -> ()  [unwired: 2 in, 2 out]
        n823 = property on="Frequency 2" class="Knob (strict)"("Value"=w1597) -> ()  [unwired: 2 in, 2 out]
        n824 = property on="Trigger pulses" class="DigNum (strict)"("Value"=w1605) -> ()  [unwired: 2 in, 2 out]
        n825 = property class="DAQmx Timing"(reference=w1620, error in=w1618, "SampQuant.SampPerChan"=w1600) -> (reference out=w1619:refnum<k21>, error out=w1617:errorcluster)
        n826 = property class="DAQmx Timing"(reference=w1624, error in=w1622, "SampQuant.SampPerChan"=w1600) -> (reference out=w1623:refnum<k21>, error out=w1621:errorcluster)
        n827 = property on="Laser pulses" class="DigNum (strict)"("Value"=w1600) -> ()  [unwired: 2 in, 2 out]
        n828 = Subtract(x=w1610, y=w1589) -> (x-y=w1612:dbl)
        n829 = Multiply(x=w1589, y=w1598) -> (x*y=w1606:dbl)
        n830 = Multiply(x=w1598, y=w1612) -> (x*y=w1611:dbl)
        n831 = To Long Integer(number=w1606) -> (32bit integer=w1607:i32)
        n832 = Subtract(x=w1605, y=w1607) -> (x-y=w1608:i32)
        n833 = To Long Integer(number=w1611) -> (32bit integer=w1609:i32)
        n834 = property on="Frames to acquire" class="DigNum (strict)"("Value"=w1608) -> ()  [unwired: 2 in, 2 out]
        n835 = property on="Initial frames" class="DigNum (strict)"("Value"=w1609) -> ()  [unwired: 2 in, 2 out]
        n836 = Merge Errors(w1627, w1617, w1621) -> (w1651:errorcluster)
      }
      event "Duty Cycle 2": Value Change {
        # "Trigger"
        # "473 nm"
        # "561 nm"
        n837 = event-data() -> ()  [unwired: 1 in, 1 out]
        n838 = call <vilib>:"DAQmx Stop Task.vi"("task/channels in"=w1711, "error in"=w1710) -> ("task out"=w1705:refnum<k21>, "error out"=w1704:errorcluster)  [unwired: 12 in]
        n839 = call <vilib>:"DAQmx Stop Task.vi"("task/channels in"=w1716, "error in"=w1712) -> ("task out"=w1709:refnum<k21>, "error out"=w1708:errorcluster)  [unwired: 12 in]
        n840 = call <vilib>:"DAQmx Stop Task.vi"("task/channels in"=w1715, "error in"=w1713) -> ("task out"=w1707:refnum<k21>, "error out"=w1706:errorcluster)  [unwired: 12 in]
        n841 = local read "Duty Cycle camera 2"() -> (w1690:dbl)
        n842 = local read "Duty Cycle 2"() -> (w1678:dbl)
        n843 = Greater?(x=w1678, y=0.5) -> (0:w1679:bool)
        n844 = Select(t="WARNING! Laser DC > 0.5\nAFLEX not possible", s=w1679, f="AFLEX conditions\nnormal") -> (s? t:f=w1680:string)
        n845 = local read "Frequency 2"() -> (w1686:dbl)
        n846 = Multiply(x=w1686, y=2) -> (x*y=w1702:dbl)
        n847 = local read "Frame rate 2"() -> (w1689:dbl)
        n848 = Reciprocal(x=w1702) -> (1/x=w1687:dbl)
        n849 = property on="AFLEX warning 2" class="Bool (strict)"("Caption.Text"=w1680, "Value"=w1679) -> ()  [unwired: 2 in, 2 out]
        n850 = Multiply(x=w1687, y=1000) -> (x*y=w1700:dbl)
        n851 = property class="DAQmx Channel"(reference=w1709, error in=w1708, "CO.Pulse.Freq"=w1689, "CO.Pulse.DutyCyc"=w1690) -> (reference out=w1699:refnum<k21>, error out=w1692:errorcluster)
        n852 = property class="DAQmx Channel"(reference=w1707, error in=w1706, "CO.Pulse.Freq"=w1686, "CO.Pulse.DutyCyc"=w1678, "CO.Pulse.Freq.InitialDelay"=0.0) -> (reference out=w1693:refnum<k21>, error out=w1694:errorcluster)
        n853 = property class="DAQmx Channel"(reference=w1705, error in=w1704, "CO.Pulse.Freq"=w1686, "CO.Pulse.DutyCyc"=w1678, "CO.Pulse.Freq.InitialDelay"=w1687) -> (reference out=w1696:refnum<k21>, error out=w1695:errorcluster)
        n854 = property on="initial delay\n473 nm (ms) 2" class="DigNum (strict)"("Value"=w1700) -> ()  [unwired: 2 in, 2 out]
        n855 = property on="Frame rate" class="Knob (strict)"(error in=w1692, "Value"=w1689) -> (error out=w1698:errorcluster)  [unwired: 1 in, 1 out]
        n856 = property on="Duty Cycle camera" class="Knob (strict)"(error in=w1698, "Value"=w1690) -> (error out=w1691:errorcluster)  [unwired: 1 in, 1 out]
        n857 = property on="Frequency 1" class="Knob (strict)"(error in=w1694, "Value"=w1686) -> (error out=w1697:errorcluster)  [unwired: 1 in, 1 out]
        n858 = property on="Duty Cycle 1" class="Knob (strict)"(error in=w1697, "Value"=w1678) -> (error out=w1685:errorcluster)  [unwired: 1 in, 1 out]
        n859 = property on="Duty Cycle 2\nmemory" class="Knob (strict)"(error in=w1685, "Value"=w1678) -> (error out=w1684:errorcluster)  [unwired: 1 in, 1 out]
        n860 = Merge Errors(w1691, w1684, w1695) -> (w1714:errorcluster)
      }
      event "HALF DC 2": Value Change {
        n861 = event-data() -> ()  [unwired: 1 in, 1 out]
        n862 = flat-sequence {
          tunnel: w1727 -> [w1756]
          tunnel: w1738 -> [w1757]
          tunnel: w1739 -> [w1758]
          tunnel: w1740 -> [w1759]
          tunnel: w1742 -> [w1760]
          tunnel: w1743 -> [w1761]
          tunnel: [w1761] -> w1734
          tunnel: [w1760] -> w1733
          tunnel: [w1759] -> w1732
          tunnel: [w1758] -> w1731
          tunnel: [w1757] -> w1730
          tunnel: [w1755] -> w1729
          tunnel: [w1754] -> w1728
          tunnel: w1726 -> [w1752]
          tunnel: w1725 -> [w1751]
          tunnel: [w1750] -> w1724
          tunnel: [w1749] -> w1723
          tunnel: [w1748] -> w1722
          tunnel: [w1747] -> w1721
          tunnel: [w1879] -> w1741
          tunnel: [w1865] -> w1737
          tunnel: [w1862] -> w1736
          tunnel: [w1859] -> w1735
          tunnel: w1734 -> [w1881]
          tunnel: w1733 -> [w1880]
          tunnel: w1732 -> [w1878]
          tunnel: w1731 -> [w1877]
          tunnel: w1730 -> [w1876]
          tunnel: w1729 -> [w1850]
          tunnel: w1728 -> [w1849]
          tunnel: w1724 -> [w1847]
          tunnel: w1723 -> [w1848]
          tunnel: w1722 -> [w1845]
          tunnel: w1721 -> [w1846]
          tunnel: [w1848] -> w1720
          tunnel: [w1847] -> w1719
          tunnel: [w1846] -> w1718
          tunnel: [w1845] -> w1717
          frame #0 {
            n863 = property on="Power control" class="Bool (strict)"() -> ("Value"=w1753:bool)  [unwired: 2 in, 2 out]
            n864 = property on="473 task" class="DAQmxName (strict)"() -> ("Value"=w1744:refnum<k21>)  [unwired: 2 in, 2 out]
            n865 = property on="561 task" class="DAQmxName (strict)"() -> ("Value"=w1745:refnum<k21>)  [unwired: 2 in, 2 out]
            n866 = case shown="True" w1753 {
              tunnel: w1756 -> [w1775 w1810]
              tunnel: [w1768 w1807] -> w1755
              tunnel: [w1767 w1823] -> w1754
              tunnel: w1752 -> [w1765 w1814]
              tunnel: w1751 -> [w1766 w1813]
              tunnel: [w1766 w1811] -> w1750
              tunnel: [w1762 w1812] -> w1749
              tunnel: [w1763 w1816] -> w1748
              tunnel: [w1765 w1815] -> w1747
              tunnel: "HALF DC 2" -> [w1764 w1806]
              tunnel: w1745 -> [w1763 w1805]
              tunnel: w1744 -> [w1762 w1804]
              frame False {
                n867 = case shown="True" w1764 {
                  tunnel: w1775 -> [w1786 w1799]
                  tunnel: [w1776 w1792] -> w1769
                  tunnel: [w1783 w1796] -> w1767
                  frame True {
                    n868 = property on="Duty Cycle 2" class="Knob (strict)"(error in=w1786) -> (error out=w1787:errorcluster, "Value"=w1788:dbl)  [unwired: 1 in, 1 out]
                    n869 = Number To Decimal String(number="Duty Cycle \nDenominator 2") -> (decimal integer string=w1780:string)  [unwired: 1 in]
                    n870 = Divide(x=w1788, y="Duty Cycle \nDenominator 2") -> (x/y=w1784:dbl)
                    n871 = property on="Duty Cycle 2" class="Knob (strict)"(error in=w1787, "Value"=w1784) -> (error out=w1777:errorcluster)  [unwired: 1 in, 1 out]
                    n872 = Concatenate Strings("1/" ("string"), w1780) -> (w1779:string)
                    n873 = property on="HALF DC 2" class="Bool (strict)"(error in=w1777, "BoolText.Text"=w1779) -> (error out=w1776:errorcluster)  [unwired: 1 in, 1 out]
                    n874 = Less?(x=w1784, y=0.0001) -> (x < y?=w1785:bool)
                    n875 = case shown="False" w1785 {
                      tunnel: [w1789 0.0001] -> w1783
                      tunnel: w1784 -> [w1789 _]
                      frame False {
                      }
                      frame True {
                      }
                    }
                  }
                  frame False {
                    n876 = property on="Duty Cycle \nDenominator 2" class="DigNum (strict)"() -> ("Value"=w1795:dbl)  [unwired: 2 in, 2 out]
                    n877 = property on="Duty Cycle 2" class="Knob (strict)"(error in=w1799) -> (error out=w1800:errorcluster, "Value"=w1801:dbl)  [unwired: 1 in, 1 out]
                    n878 = Multiply(x=w1801, y=w1795) -> (x*y=w1794:dbl)
                    n879 = property on="Duty Cycle 2" class="Knob (strict)"(error in=w1800, "Value"=w1794) -> (error out=w1793:errorcluster)  [unwired: 1 in, 1 out]
                    n880 = property on="HALF DC 2" class="Bool (strict)"(error in=w1793, "BoolText.Text"="1/1" ("Boolean Text.Text")) -> (error out=w1792:errorcluster)  [unwired: 1 in, 1 out]
                    n881 = Greater Or Equal?(x=w1794, y=1) -> (x >= y?=w1797:bool)
                    n882 = case shown="False" w1797 {
                      tunnel: [w1802 0.9999] -> w1796
                      tunnel: w1794 -> [w1802 _]
                      frame False {
                      }
                      frame True {
                      }
                    }
                  }
                }
                n883 = Greater?(x=w1767, y=0.5) -> (0:w1774:bool)
                n884 = Select(t="WARNING! Laser DC > 0.5\nAFLEX not possible", s=w1774, f="AFLEX conditions\nnormal") -> (s? t:f=w1773:string)
                n885 = property on="AFLEX warning 2" class="Bool (strict)"(error in=w1769, "Caption.Text"=w1773, "Value"=w1774) -> (error out=w1768:errorcluster)  [unwired: 1 in, 1 out]
              }
              frame True {
                n886 = property on="Duty Cycle \nDenominator 2" class="DigNum (strict)"(error in=w1810) -> (error out=w1808:errorcluster, "Value"=w1809:dbl)  [unwired: 1 in, 1 out]
                n887 = property on="Level at max 473nm (0-5V)" class="DigNum (strict)"(error in=w1813) -> (error out=w1821:errorcluster, "Value"=w1822:dbl)  [unwired: 1 in, 1 out]
                n888 = case shown="False" w1806 {
                  tunnel: w1809 -> [_ w1829]
                  tunnel: w1808 -> [w1826 w1828]
                  tunnel: [w1825 w1827] -> w1807
                  frame False {
                    n889 = property on="HALF DC 2" class="Bool (strict)"(error in=w1826, "BoolText.Text"="1/1" ("Boolean Text.Text")) -> (error out=w1825:errorcluster)  [unwired: 1 in, 1 out]
                  }
                  frame True {
                    n890 = Number To Decimal String(number=w1829) -> (decimal integer string=w1832:string)  [unwired: 1 in]
                    n891 = Concatenate Strings("1/" ("string"), w1832) -> (w1830:string)
                    n892 = property on="HALF DC 2" class="Bool (strict)"(error in=w1828, "BoolText.Text"=w1830) -> (error out=w1827:errorcluster)  [unwired: 1 in, 1 out]
                  }
                }
                n893 = case shown="True" w1806 {
                  tunnel: w1809 -> [_ w1838]
                  tunnel: [w1833 w1836] -> w1820
                  tunnel: w1822 -> [w1833 w1834]
                  frame False {
                  }
                  frame True {
                    n894 = Divide(x=1.0, y=w1838) -> (x/y=w1835:dbl)
                    n895 = Multiply(x=w1835, y=w1834) -> (x*y=w1836:dbl)
                  }
                }
                n896 = property on="Level at max 561nm (0-5V)" class="DigNum (strict)"(error in=w1814) -> (error out=w1818:errorcluster, "Value"=w1819:dbl)  [unwired: 1 in, 1 out]
                n897 = case shown="True" w1806 {
                  tunnel: w1809 -> [_ w1844]
                  tunnel: [w1839 w1842] -> w1817
                  tunnel: w1819 -> [w1839 w1840]
                  frame False {
                  }
                  frame True {
                    n898 = Divide(x=1.0, y=w1844) -> (x/y=w1841:dbl)
                    n899 = Multiply(x=w1841, y=w1840) -> (x*y=w1842:dbl)
                  }
                }
                n900 = call-poly <vilib>:"DAQmx Write.vi"("task/channels in"=w1805, "data"=w1817, "error in"=w1818) -> ("task out"=w1816:refnum<k21>, "error out"=w1815:errorcluster)  [unwired: 10 in, 1 out]
                n901 = call-poly <vilib>:"DAQmx Write.vi"("task/channels in"=w1804, "data"=w1820, "error in"=w1821) -> ("task out"=w1812:refnum<k21>, "error out"=w1811:errorcluster)  [unwired: 10 in, 1 out]
                n902 = property on="Duty Cycle 2" class="Knob (strict)"() -> ("Value"=w1823:dbl)  [unwired: 2 in, 2 out]
              }
            }
          }
          frame #1 {
            # "Trigger"
            # "473 nm"
            # "561 nm"
            n903 = call <vilib>:"DAQmx Stop Task.vi"("task/channels in"=w1877, "error in"=w1876) -> ("task out"=w1871:refnum<k21>, "error out"=w1870:errorcluster)  [unwired: 12 in]
            n904 = call <vilib>:"DAQmx Stop Task.vi"("task/channels in"=w1881, "error in"=w1878) -> ("task out"=w1875:refnum<k21>, "error out"=w1874:errorcluster)  [unwired: 12 in]
            n905 = call <vilib>:"DAQmx Stop Task.vi"("task/channels in"=w1880, "error in"=w1850) -> ("task out"=w1873:refnum<k21>, "error out"=w1872:errorcluster)  [unwired: 12 in]
            n906 = local read "Duty Cycle camera 2"() -> (w1855:dbl)
            n907 = local read "Frequency 2"() -> (w1851:dbl)
            n908 = Multiply(x=w1851, y=2) -> (x*y=w1868:dbl)
            n909 = local read "Frame rate 2"() -> (w1854:dbl)
            n910 = Reciprocal(x=w1868) -> (1/x=w1852:dbl)
            n911 = Multiply(x=w1852, y=1000) -> (x*y=w1866:dbl)
            n912 = property class="DAQmx Channel"(reference=w1875, error in=w1874, "CO.Pulse.Freq"=w1854, "CO.Pulse.DutyCyc"=w1855) -> (reference out=w1865:refnum<k21>, error out=w1857:errorcluster)
            n913 = property class="DAQmx Channel"(reference=w1873, error in=w1872, "CO.Pulse.Freq"=w1851, "CO.Pulse.DutyCyc"=w1849, "CO.Pulse.Freq.InitialDelay"=0.0) -> (reference out=w1859:refnum<k21>, error out=w1860:errorcluster)
            n914 = property class="DAQmx Channel"(reference=w1871, error in=w1870, "CO.Pulse.Freq"=w1851, "CO.Pulse.DutyCyc"=w1849, "CO.Pulse.Freq.InitialDelay"=w1852) -> (reference out=w1862:refnum<k21>, error out=w1861:errorcluster)
            n915 = property on="initial delay\n473 nm (ms) 2" class="DigNum (strict)"("Value"=w1866) -> ()  [unwired: 2 in, 2 out]
            n916 = property on="Frame rate" class="Knob (strict)"(error in=w1857, "Value"=w1854) -> (error out=w1864:errorcluster)  [unwired: 1 in, 1 out]
            n917 = property on="Duty Cycle camera" class="Knob (strict)"(error in=w1864, "Value"=w1855) -> (error out=w1856:errorcluster)  [unwired: 1 in, 1 out]
            n918 = property on="Frequency 1" class="Knob (strict)"(error in=w1860, "Value"=w1851) -> (error out=w1863:errorcluster)  [unwired: 1 in, 1 out]
            n919 = property on="Duty Cycle 1" class="Knob (strict)"(error in=w1863, "Value"=w1849) -> (error out=w1858:errorcluster)  [unwired: 1 in, 1 out]
            n920 = Merge Errors(w1856, w1858, w1861) -> (w1879:errorcluster)
          }
        }
      }
      event "Duty Cycle \nDenominator 2": Value Change {
        # "Trigger"
        # "473 nm"
        # "561 nm"
        n921 = event-data() -> ()  [unwired: 1 in, 1 out]
        n922 = property on="473 task" class="DAQmxName (strict)"() -> ("Value"=w1882:refnum<k21>)  [unwired: 2 in, 2 out]
        n923 = property on="HALF DC 2" class="Bool (strict)"() -> ("Value"=w1892:bool)  [unwired: 2 in, 2 out]
        n924 = property on="Power control" class="Bool (strict)"() -> ("Value"=w1890:bool)  [unwired: 2 in, 2 out]
        n925 = property on="561 task" class="DAQmxName (strict)"() -> ("Value"=w1883:refnum<k21>)  [unwired: 2 in, 2 out]
        n926 = case shown="False" w1890 {
          tunnel: w1894 -> [w1938 w1983]
          tunnel: [w1937 w1982] -> w1893
          tunnel: w1892 -> [w1936 w1967]
          tunnel: [w1930 w1984] -> w1891
          tunnel: [w1927 w1975] -> w1887
          tunnel: [w1926 w1974] -> w1885
          tunnel: w1889 -> [w1929 w1973]
          tunnel: [w1929 w1972] -> w1884
          tunnel: w1888 -> [w1928 w1971]
          tunnel: [w1928 w1968] -> w1886
          tunnel: w1883 -> [w1927 w1966]
          tunnel: w1882 -> [w1926 w1965]
          frame False {
            n927 = case shown="True" w1936 {
              tunnel: w1938 -> [w1949 w1961]
              tunnel: [w1940 w1955] -> w1937
              tunnel: [w1946 w1958] -> w1930
              frame True {
                n928 = property on="Duty Cycle \nDenominator 2" class="DigNum (strict)"() -> ("Value"=w1939:dbl)  [unwired: 2 in, 2 out]
                n929 = property on="Duty Cycle 2\nmemory" class="Knob (strict)"(error in=w1949) -> (error out=w1950:errorcluster, "Value"=w1951:dbl)  [unwired: 1 in, 1 out]
                n930 = Number To Decimal String(number=w1939) -> (decimal integer string=w1943:string)  [unwired: 1 in]
                n931 = Divide(x=w1951, y=w1939) -> (x/y=w1947:dbl)
                n932 = property on="Duty Cycle 2" class="Knob (strict)"(error in=w1950, "Value"=w1947) -> (error out=w1941:errorcluster)  [unwired: 1 in, 1 out]
                n933 = Concatenate Strings("1/" ("string"), w1943) -> (w1942:string)
                n934 = property on="HALF DC 2" class="Bool (strict)"(error in=w1941, "BoolText.Text"=w1942) -> (error out=w1940:errorcluster)  [unwired: 1 in, 1 out]
                n935 = Less?(x=w1947, y=0.0001) -> (x < y?=w1948:bool)
                n936 = case shown="True" w1948 {
                  tunnel: [w1952 0.0001] -> w1946
                  tunnel: w1947 -> [w1952 _]
                  frame False {
                  }
                  frame True {
                  }
                }
              }
              frame False {
                n937 = property on="Duty Cycle 2\nmemory" class="Knob (strict)"(error in=w1961) -> (error out=w1962:errorcluster, "Value"=w1957:dbl)  [unwired: 1 in, 1 out]
                n938 = property on="Duty Cycle 2" class="Knob (strict)"(error in=w1962, "Value"=w1957) -> (error out=w1956:errorcluster)  [unwired: 1 in, 1 out]
                n939 = property on="HALF DC 2" class="Bool (strict)"(error in=w1956, "BoolText.Text"="1/1" ("Boolean Text.Text")) -> (error out=w1955:errorcluster)  [unwired: 1 in, 1 out]
                n940 = Greater Or Equal?(x=w1957, y=1) -> (x >= y?=w1959:bool)
                n941 = case shown="False" w1959 {
                  tunnel: [w1963 0.9999] -> w1958
                  tunnel: w1957 -> [w1963 _]
                  frame False {
                  }
                  frame True {
                  }
                }
              }
            }
            n942 = Greater?(x=w1930, y=0.5) -> (0:w1931:bool)
            n943 = Select(t="WARNING! Laser DC > 0.5\nAFLEX not possible", s=w1931, f="AFLEX conditions\nnormal") -> (s? t:f=w1932:string)
            n944 = property on="AFLEX warning 2" class="Bool (strict)"("Caption.Text"=w1932, "Value"=w1931) -> ()  [unwired: 2 in, 2 out]
          }
          frame True {
            n945 = property on="Duty Cycle \nDenominator 2" class="DigNum (strict)"() -> ("Value"=w1970:dbl)  [unwired: 2 in, 2 out]
            n946 = property on="Duty Cycle 2" class="Knob (strict)"(error in=w1983) -> (error out=w1982:errorcluster, "Value"=w1984:dbl)  [unwired: 1 in, 1 out]
            n947 = property on="Level at max 561nm (0-5V)" class="DigNum (strict)"(error in=w1971) -> (error out=w1980:errorcluster, "Value"=w1981:dbl)  [unwired: 1 in, 1 out]
            n948 = case shown="True" w1967 {
              tunnel: w1970 -> [_ w2005]
              tunnel: [w2000 w2003] -> w1979
              tunnel: w1981 -> [w2000 w2001]
              frame False {
              }
              frame True {
                n949 = Divide(x=1.0, y=w2005) -> (x/y=w2002:dbl)
                n950 = Multiply(x=w2002, y=w2001) -> (x*y=w2003:dbl)
              }
            }
            n951 = call-poly <vilib>:"DAQmx Write.vi"("task/channels in"=w1966, "data"=w1979, "error in"=w1980) -> ("task out"=w1975:refnum<k21>, "error out"=w1969:errorcluster)  [unwired: 10 in, 1 out]
            n952 = case shown="False" w1967 {
              tunnel: w1970 -> [_ w1990]
              tunnel: w1969 -> [w1987 w1989]
              tunnel: [w1986 w1988] -> w1968
              frame False {
                n953 = property on="HALF DC 2" class="Bool (strict)"(error in=w1987, "BoolText.Text"="1/1" ("Boolean Text.Text")) -> (error out=w1986:errorcluster)  [unwired: 1 in, 1 out]
              }
              frame True {
                n954 = Number To Decimal String(number=w1990) -> (decimal integer string=w1993:string)  [unwired: 1 in]
                n955 = Concatenate Strings("1/" ("string"), w1993) -> (w1991:string)
                n956 = property on="HALF DC 2" class="Bool (strict)"(error in=w1989, "BoolText.Text"=w1991) -> (error out=w1988:errorcluster)  [unwired: 1 in, 1 out]
              }
            }
            n957 = property on="Level at max 473nm (0-5V)" class="DigNum (strict)"(error in=w1973) -> (error out=w1977:errorcluster, "Value"=w1978:dbl)  [unwired: 1 in, 1 out]
            n958 = case shown="True" w1967 {
              tunnel: w1970 -> [_ w1999]
              tunnel: [w1994 w1997] -> w1976
              tunnel: w1978 -> [w1994 w1995]
              frame False {
              }
              frame True {
                n959 = Divide(x=1.0, y=w1999) -> (x/y=w1996:dbl)
                n960 = Multiply(x=w1996, y=w1995) -> (x*y=w1997:dbl)
              }
            }
            n961 = call-poly <vilib>:"DAQmx Write.vi"("task/channels in"=w1965, "data"=w1976, "error in"=w1977) -> ("task out"=w1974:refnum<k21>, "error out"=w1972:errorcluster)  [unwired: 10 in, 1 out]
          }
        }
        n962 = call <vilib>:"DAQmx Stop Task.vi"("task/channels in"=w1921, "error in"=w1920) -> ("task out"=w1915:refnum<k21>, "error out"=w1914:errorcluster)  [unwired: 12 in]
        n963 = call <vilib>:"DAQmx Stop Task.vi"("task/channels in"=w1925, "error in"=w1922) -> ("task out"=w1919:refnum<k21>, "error out"=w1918:errorcluster)  [unwired: 12 in]
        n964 = call <vilib>:"DAQmx Stop Task.vi"("task/channels in"=w1924, "error in"=w1893) -> ("task out"=w1917:refnum<k21>, "error out"=w1916:errorcluster)  [unwired: 12 in]
        n965 = local read "Duty Cycle camera 2"() -> (w1899:dbl)
        n966 = local read "Frequency 2"() -> (w1895:dbl)
        n967 = Multiply(x=w1895, y=2) -> (x*y=w1912:dbl)
        n968 = local read "Frame rate 2"() -> (w1898:dbl)
        n969 = Reciprocal(x=w1912) -> (1/x=w1896:dbl)
        n970 = Multiply(x=w1896, y=1000) -> (x*y=w1910:dbl)
        n971 = property class="DAQmx Channel"(reference=w1919, error in=w1918, "CO.Pulse.Freq"=w1898, "CO.Pulse.DutyCyc"=w1899) -> (reference out=w1909:refnum<k21>, error out=w1901:errorcluster)
        n972 = property class="DAQmx Channel"(reference=w1917, error in=w1916, "CO.Pulse.Freq"=w1895, "CO.Pulse.DutyCyc"=w1891, "CO.Pulse.Freq.InitialDelay"=0.0) -> (reference out=w1903:refnum<k21>, error out=w1904:errorcluster)
        n973 = property class="DAQmx Channel"(reference=w1915, error in=w1914, "CO.Pulse.Freq"=w1895, "CO.Pulse.DutyCyc"=w1891, "CO.Pulse.Freq.InitialDelay"=w1896) -> (reference out=w1906:refnum<k21>, error out=w1905:errorcluster)
        n974 = property on="initial delay\n473 nm (ms) 2" class="DigNum (strict)"("Value"=w1910) -> ()  [unwired: 2 in, 2 out]
        n975 = property on="Frame rate" class="Knob (strict)"(error in=w1901, "Value"=w1898) -> (error out=w1908:errorcluster)  [unwired: 1 in, 1 out]
        n976 = property on="Duty Cycle camera" class="Knob (strict)"(error in=w1908, "Value"=w1899) -> (error out=w1900:errorcluster)  [unwired: 1 in, 1 out]
        n977 = property on="Frequency 1" class="Knob (strict)"(error in=w1904, "Value"=w1895) -> (error out=w1907:errorcluster)  [unwired: 1 in, 1 out]
        n978 = property on="Duty Cycle 1" class="Knob (strict)"(error in=w1907, "Value"=w1891) -> (error out=w1902:errorcluster)  [unwired: 1 in, 1 out]
        n979 = Merge Errors(w1900, w1902, w1905) -> (w1923:errorcluster)
      }
      event "HALF DC": Value Change {
        n980 = event-data() -> ()  [unwired: 1 in, 1 out]
        n981 = call <vilib>:"DAQmx Stop Task.vi"("task/channels in"=w2038, "error in"=w2037) -> ("task out"=w2036:refnum<k21>, "error out"=w2035:errorcluster)  [unwired: 12 in]
        n982 = call <vilib>:"DAQmx Stop Task.vi"("task/channels in"=w2019, "error in"=w2017) -> ("task out"=w2018:refnum<k21>, "error out"=w2016:errorcluster)  [unwired: 12 in]
        n983 = call <vilib>:"DAQmx Stop Task.vi"("task/channels in"=w2023, "error in"=w2021) -> ("task out"=w2022:refnum<k21>, "error out"=w2020:errorcluster)  [unwired: 12 in]
        n984 = flat-sequence {
          tunnel: w2035 -> [w2051]
          tunnel: w2036 -> [w2052]
          tunnel: w2020 -> [w2057]
          tunnel: w2018 -> [w2058]
          tunnel: w2022 -> [w2059]
          tunnel: [w2059] -> w2031
          tunnel: [w2058] -> w2030
          tunnel: [w2057] -> w2029
          tunnel: [w2052] -> w2028
          tunnel: [w2049] -> w2027
          tunnel: [w2056] -> w2026
          tunnel: [w2055] -> w2025
          tunnel: "HALF DC" -> [w2054]
          tunnel: w2016 -> [w2053]
          tunnel: w2015 -> [w2047]
          tunnel: [w2046] -> w2014
          tunnel: w2012 -> [w2045]
          tunnel: [w2044] -> w2011
          tunnel: [w2043] -> w2009
          tunnel: [w2042] -> w2008
          tunnel: [w2217] -> w2039
          tunnel: [w2202] -> w2034
          tunnel: [w2196] -> w2033
          tunnel: [w2192] -> w2032
          tunnel: w2031 -> [w2175]
          tunnel: w2030 -> [w2177]
          tunnel: w2029 -> [w2174]
          tunnel: w2028 -> [w2209]
          tunnel: w2027 -> [w2208]
          tunnel: w2026 -> [w2176]
          tunnel: w2025 -> [w2178]
          tunnel: w2014 -> [w2165]
          tunnel: [w2165] -> w2013
          tunnel: w2011 -> [w2164]
          tunnel: [w2164] -> w2010
          tunnel: w2009 -> [w2163]
          tunnel: w2008 -> [w2162]
          tunnel: [w2163] -> w2007
          tunnel: [w2162] -> w2006
          frame #0 {
            # "Switch between full power and low power\nstates"
            n985 = property on="Power control" class="Bool (strict)"() -> ("Value"=w2048:bool)  [unwired: 2 in, 2 out]
            n986 = property on="473 task" class="DAQmxName (strict)"() -> ("Value"=w2040:refnum<k21>)  [unwired: 2 in, 2 out]
            n987 = property on="561 task" class="DAQmxName (strict)"() -> ("Value"=w2041:refnum<k21>)  [unwired: 2 in, 2 out]
            n988 = case shown="True" w2048 {
              tunnel: [w2076 w2115] -> w2056
              tunnel: [w2075 w2128] -> w2055
              tunnel: w2054 -> [w2074 w2116]
              tunnel: w2053 -> [w2073 w2129]
              tunnel: w2051 -> [w2067 w2118]
              tunnel: "Duty Cycle \nDenominator" -> [w2065 w2119]
              tunnel: [w2064 w2117] -> w2049
              tunnel: w2047 -> [w2063 w2133]
              tunnel: [w2060 w2127] -> w2046
              tunnel: w2045 -> [w2062 w2123]
              tunnel: [w2061 w2122] -> w2044
              tunnel: [w2063 w2121] -> w2043
              tunnel: [w2062 w2120] -> w2042
              tunnel: w2041 -> [w2060 w2114]
              tunnel: w2040 -> [w2061 w2113]
              frame False {
                n989 = case shown="False" w2074 {
                  tunnel: [w2085 w2105] -> w2076
                  tunnel: [w2078 w2103] -> w2075
                  tunnel: w2073 -> [w2087 w2099]
                  tunnel: [w2078 w2103] -> w2066
                  tunnel: w2065 -> [w2077 w2100]
                  frame True {
                    n990 = property on="Duty Cycle 1" class="Knob (strict)"(error in=w2087) -> (error out=w2093:errorcluster, "Value"=w2092:dbl)  [unwired: 1 in, 1 out]
                    n991 = Divide(x=w2092, y=w2077) -> (x/y=w2080:dbl)
                    n992 = Number To Decimal String(number=w2077) -> (decimal integer string=w2082:string)  [unwired: 1 in]
                    n993 = property on="Duty Cycle 1" class="Knob (strict)"(error in=w2093, "Value"=w2080) -> (error out=w2079:errorcluster)  [unwired: 1 in, 1 out]
                    n994 = property on="Duty Cycle 1\npreset" class="Knob (strict)"(error in=w2079, "Value"=w2080) -> (error out=w2081:errorcluster)  [unwired: 1 in, 1 out]
                    n995 = property on="Low Power\nFrames" class="DigNum (strict)"(error in=w2081) -> (error out=w2089:errorcluster, "Value"=w2088:i32)  [unwired: 1 in, 1 out]
                    n996 = property on="Illuminated Frames" class="DigNum (strict)"(error in=w2089, "Value"=w2088) -> (error out=w2086:errorcluster)  [unwired: 1 in, 1 out]
                    n997 = Concatenate Strings("1/" ("string"), w2082) -> (w2084:string)
                    n998 = Less?(x=w2080, y=0.0001) -> (x < y?=w2090:bool)
                    n999 = case shown="False" w2090 {
                      tunnel: [w2094 0.0001] -> w2078
                      tunnel: w2080 -> [w2094 _]
                      frame False {
                      }
                      frame True {
                      }
                    }
                    n1000 = property on="HALF DC" class="Bool (strict)"(error in=w2086, "BoolText.Text"=w2084) -> (error out=w2085:errorcluster)  [unwired: 1 in, 1 out]
                  }
                  frame False {
                    n1001 = property on="Duty Cycle 1" class="Knob (strict)"() -> ("Value"=w2110:dbl)  [unwired: 2 in, 2 out]
                    n1002 = Multiply(x=w2110, y=w2100) -> (x*y=w2102:dbl)
                    n1003 = property on="Duty Cycle 1" class="Knob (strict)"(error in=w2099, "Value"=w2102) -> (error out=w2104:errorcluster)  [unwired: 1 in, 1 out]
                    n1004 = property on="Duty Cycle 1\npreset" class="Knob (strict)"(error in=w2104, "Value"=w2102) -> (error out=w2101:errorcluster)  [unwired: 1 in, 1 out]
                    n1005 = property on="Duty Cycle 1\nfull DC" class="Knob (strict)"(error in=w2101, "Value"=w2102) -> (error out=w2098:errorcluster)  [unwired: 1 in, 1 out]
                    n1006 = property on="HALF DC" class="Bool (strict)"(error in=w2098, "BoolText.Text"="1/1" ("Boolean Text.Text")) -> (error out=w2097:errorcluster)  [unwired: 1 in, 1 out]
                    n1007 = property on="Full Power \nFrames" class="DigNum (strict)"(error in=w2097) -> (error out=w2107:errorcluster, "Value"=w2106:i32)  [unwired: 1 in, 1 out]
                    n1008 = Greater Or Equal?(x=w2102, y=1) -> (x >= y?=w2109:bool)
                    n1009 = property on="Illuminated Frames" class="DigNum (strict)"(error in=w2107, "Value"=w2106) -> (error out=w2105:errorcluster)  [unwired: 1 in, 1 out]
                    n1010 = case shown="False" w2109 {
                      tunnel: [w2111 0.9999] -> w2103
                      tunnel: w2102 -> [w2111 _]
                      frame False {
                      }
                      frame True {
                      }
                    }
                  }
                }
                n1011 = Greater?(x=w2066, y=0.5) -> (0:w2068:bool)
                n1012 = Select(t="WARNING! Laser DC > 0.5\nAFLEX not possible", s=w2068, f="AFLEX conditions\nnormal") -> (s? t:f=w2069:string)
                n1013 = property on="AFLEX warning" class="Bool (strict)"(error in=w2067, "Caption.Text"=w2069, "Value"=w2068) -> (error out=w2064:errorcluster)  [unwired: 1 in, 1 out]
              }
              frame True {
                n1014 = property on="Duty Cycle 1" class="Knob (strict)"(error in=w2129) -> (error out=w2115:errorcluster, "Value"=w2128:dbl)  [unwired: 1 in, 1 out]
                n1015 = case shown="True" w2116 {
                  tunnel: w2119 -> [_ w2145]
                  tunnel: w2118 -> [w2137 w2141]
                  tunnel: [w2135 w2144] -> w2117
                  frame False {
                    n1016 = property on="Full Power \nFrames" class="DigNum (strict)"(error in=w2137) -> (error out=w2138:errorcluster, "Value"=w2139:i32)  [unwired: 1 in, 1 out]
                    n1017 = property on="Illuminated Frames" class="DigNum (strict)"(error in=w2138, "Value"=w2139) -> (error out=w2136:errorcluster)  [unwired: 1 in, 1 out]
                    n1018 = property on="HALF DC" class="Bool (strict)"(error in=w2136, "BoolText.Text"="1/1" ("Boolean Text.Text")) -> (error out=w2135:errorcluster)  [unwired: 1 in, 1 out]
                  }
                  frame True {
                    n1019 = Number To Decimal String(number=w2145) -> (decimal integer string=w2146:string)  [unwired: 1 in]
                    n1020 = property on="Low Power\nFrames" class="DigNum (strict)"(error in=w2141) -> (error out=w2143:errorcluster, "Value"=w2142:i32)  [unwired: 1 in, 1 out]
                    n1021 = Concatenate Strings("1/" ("string"), w2146) -> (w2148:string)
                    n1022 = property on="Illuminated Frames" class="DigNum (strict)"(error in=w2143, "Value"=w2142) -> (error out=w2140:errorcluster)  [unwired: 1 in, 1 out]
                    n1023 = property on="HALF DC" class="Bool (strict)"(error in=w2140, "BoolText.Text"=w2148) -> (error out=w2144:errorcluster)  [unwired: 1 in, 1 out]
                  }
                }
                n1024 = property on="Level at max 473nm (0-5V)" class="DigNum (strict)"(error in=w2123) -> (error out=w2125:errorcluster, "Value"=w2124:dbl)  [unwired: 1 in, 1 out]
                n1025 = case shown="True" w2116 {
                  tunnel: w2119 -> [_ w2154]
                  tunnel: [w2149 w2152] -> w2126
                  tunnel: w2124 -> [w2149 w2150]
                  frame False {
                  }
                  frame True {
                    n1026 = Divide(x=1.0, y=w2154) -> (x/y=w2151:dbl)
                    n1027 = Multiply(x=w2151, y=w2150) -> (x*y=w2152:dbl)
                  }
                }
                n1028 = property on="Level at max 561nm (0-5V)" class="DigNum (strict)"(error in=w2133) -> (error out=w2131:errorcluster, "Value"=w2130:dbl)  [unwired: 1 in, 1 out]
                n1029 = case shown="True" w2116 {
                  tunnel: w2119 -> [_ w2160]
                  tunnel: [w2155 w2158] -> w2132
                  tunnel: w2130 -> [w2155 w2156]
                  frame False {
                  }
                  frame True {
                    n1030 = Divide(x=1.0, y=w2160) -> (x/y=w2157:dbl)
                    n1031 = Multiply(x=w2157, y=w2156) -> (x*y=w2158:dbl)
                  }
                }
                n1032 = call-poly <vilib>:"DAQmx Write.vi"("task/channels in"=w2113, "data"=w2126, "error in"=w2125) -> ("task out"=w2122:refnum<k21>, "error out"=w2120:errorcluster)  [unwired: 10 in, 1 out]
                n1033 = call-poly <vilib>:"DAQmx Write.vi"("task/channels in"=w2114, "data"=w2132, "error in"=w2131) -> ("task out"=w2127:refnum<k21>, "error out"=w2121:errorcluster)  [unwired: 10 in, 1 out]
              }
            }
          }
          frame #1 {
            (unwired) 0.05 ("x")
            (unwired) 0.05 ("y")
            # "Force system to calculate from updated values"
            # "Trigger"
            # "473 nm"
            # "561 nm"
            n1034 = local read "First frame\ndelay (ms)"() -> (w2213:dbl)
            n1035 = local read "Frequency 1"() -> (w2168:dbl)
            n1036 = local read "Duty Cycle camera"() -> (w2211:dbl)
            n1037 = property on="Continous ill" class="Bool (strict)"() -> ("Value"=w2173:bool)  [unwired: 2 in, 2 out]
            n1038 = local read "Frame rate"() -> (w2169:dbl)
            n1039 = property class="DAQmx Channel"(reference=w2175, error in=w2174, "CO.Pulse.Freq"=w2169, "CO.Pulse.DutyCyc"=w2211) -> (reference out=w2203:refnum<k21>, error out=w2201:errorcluster)
            n1040 = Divide(x=w2213, y=1000) -> (x/y=w2183:dbl)
            n1041 = Multiply(x=w2169, y=w2183) -> (x*y=w2215:dbl)
            n1042 = To Long Integer(number=w2215) -> (32bit integer=w2198:i32)
            n1043 = Reciprocal(x=w2169) -> (1/x=w2214:dbl)
            n1044 = local read "Illuminated Frames"() -> (w2172:i32)
            n1045 = Multiply(x=w2198, y=w2214) -> (x*y=w2204:dbl)
            n1046 = local read "Finishing frames"() -> (w2199:i32)
            n1047 = property on="Initial calculated\ndelay (frames)" class="DigNum (strict)"("Value"=w2215) -> ()  [unwired: 2 in, 2 out]
            n1048 = Multiply(x=w2204, y=1000) -> (x*y=w2210:dbl)
            n1049 = property on="delay\ncompensation" class="DigNum (strict)"() -> ("Value"=w2161:dbl)  [unwired: 2 in, 2 out]
            n1050 = property on="Laser delay (ms)" class="DigNum (strict)"("Value"=w2210) -> ()  [unwired: 2 in, 2 out]
            n1051 = Add(x=w2172, y=w2198) -> (x+y=w2187:i32)
            n1052 = Divide(x=w2172, y=2) -> (x/y=w2188:dbl)
            n1053 = Subtract(x=w2183, y=w2161) -> (x-y=w2185:dbl)
            n1054 = Multiply(x=w2161, y=w2169) -> (x*y=w2180:dbl)
            n1055 = To Long Integer(number=w2188) -> (32bit integer=w2171:i32)
            n1056 = case shown="False" w2173 {
              tunnel: [w2223 w2243] -> w2167
              tunnel: w2169 -> [w2225 w2244]
              tunnel: w2168 -> [w2226 _]
              tunnel: w2172 -> [w2219 w2248]
              tunnel: [w2220 1] -> w2170
              tunnel: [w2218 w2245] -> _
              tunnel: w2171 -> [w2222 _]
              tunnel: [w2224 0.0] -> w2166
              frame False {
                n1057 = property on="Frequency 1" class="Knob (strict)" props=["Value"]() -> ()  [unwired: 2 in, 3 out]
                n1058 = property on="Pulsed" class="Bool (strict)"() -> ("Value"=w2221:bool)  [unwired: 2 in, 2 out]
                n1059 = local read "Duty Cycle 1\npreset"() -> (w2218:dbl)
                n1060 = case shown="False" w2221 {
                  tunnel: w2226 -> [w2234 _]
                  tunnel: w2225 -> [w2233 w2240]
                  tunnel: w2218 -> [_ _]
                  tunnel: [w2229 0.0] -> w2224
                  tunnel: [w2228 w2240] -> w2223
                  tunnel: w2222 -> [w2227 _]
                  tunnel: [w2227 w2239] -> w2220
                  tunnel: w2219 -> [_ w2239]
                  frame False {
                    n1061 = property on="Link rates" class="Bool (strict)"() -> ("Value"=w2232:bool)  [unwired: 2 in, 2 out]
                    n1062 = case shown="True" w2232 {
                      tunnel: [w2235 w2236] -> w2228
                      tunnel: w2233 -> [_ w2238]
                      tunnel: w2234 -> [w2235 _]
                      frame False {
                      }
                      frame True {
                        n1063 = Divide(x=w2238, y=2) -> (x/y=w2236:dbl)
                        n1064 = property on="Frequency 1" class="Knob (strict)"("Value"=w2236) -> ()  [unwired: 2 in, 2 out]
                      }
                    }
                    n1065 = Multiply(x=w2228, y=2) -> (x*y=w2231:dbl)
                    n1066 = Reciprocal(x=w2231) -> (1/x=w2229:dbl)
                  }
                  frame True {
                  }
                }
                n1067 = property on="Duty Cycle 1" class="Knob (strict)"("Value"=w2218) -> ()  [unwired: 2 in, 2 out]
                n1068 = property on="Duty Cycle 1\npreset" class="Knob (strict)"("Value"=w2218) -> ()  [unwired: 2 in, 2 out]
              }
              frame True {
                w2245 = 0.9999 ("x")
                n1069 = Reciprocal(x=w2244) -> (1/x=w2249:dbl)
                n1070 = Multiply(x=w2249, y=w2248) -> (x*y=w2246:dbl)
                n1071 = property on="Duty Cycle 1" class="Knob (strict)"("Value"=w2245) -> ()  [unwired: 2 in, 2 out]
                n1072 = Divide(x=w2245, y=w2246) -> (x/y=w2243:dbl)
                n1073 = property on="Frequency 1" class="Knob (strict)"("Value"=w2243) -> ()  [unwired: 2 in, 2 out]
              }
            }
            n1074 = property class="DAQmx Channel"(reference=w2177, error in=w2176, "CO.Pulse.Freq"=w2167, "CO.Pulse.DutyCyc"=w2178, "CO.Pulse.Freq.InitialDelay"=w2204) -> (reference out=w2193:refnum<k21>, error out=w2191:errorcluster)
            n1075 = Add(x=w2204, y=w2166) -> (x+y=w2205:dbl)
            n1076 = property class="DAQmx Channel"(reference=w2209, error in=w2208, "CO.Pulse.Freq"=w2167, "CO.Pulse.DutyCyc"=w2178, "CO.Pulse.Freq.InitialDelay"=w2205) -> (reference out=w2197:refnum<k21>, error out=w2195:errorcluster)
            n1077 = Multiply(x=w2166, y=1000) -> (x*y=w2206:dbl)
            n1078 = property on="Initial delay\n473 nm (ms)" class="DigNum (strict)"("Value"=w2206) -> ()  [unwired: 2 in, 2 out]
            n1079 = Add(x=w2199, y=w2187) -> (x+y=w2179:i32)
            n1080 = property class="DAQmx Timing"(reference=w2203, error in=w2201, "SampQuant.SampPerChan"=w2179) -> (reference out=w2202:refnum<k21>, error out=w2200:errorcluster)
            n1081 = Multiply(x=w2169, y=w2185) -> (x*y=w2186:dbl)
            n1082 = To Long Integer(number=w2180) -> (32bit integer=w2181:i32)
            n1083 = Subtract(x=w2179, y=w2181) -> (x-y=w2182:i32)
            n1084 = To Long Integer(number=w2186) -> (32bit integer=w2184:i32)
            n1085 = property on="Trigger pulses" class="DigNum (strict)"("Value"=w2179) -> ()  [unwired: 2 in, 2 out]
            n1086 = property class="DAQmx Timing"(reference=w2193, error in=w2191, "SampQuant.SampPerChan"=w2170) -> (reference out=w2192:refnum<k21>, error out=w2190:errorcluster)
            n1087 = property class="DAQmx Timing"(reference=w2197, error in=w2195, "SampQuant.SampPerChan"=w2170) -> (reference out=w2196:refnum<k21>, error out=w2194:errorcluster)
            n1088 = property on="Frames to acquire" class="DigNum (strict)"("Value"=w2182) -> ()  [unwired: 2 in, 2 out]
            n1089 = property on="Laser pulses" class="DigNum (strict)"("Value"=w2170) -> ()  [unwired: 2 in, 2 out]
            n1090 = property on="Initial frames" class="DigNum (strict)"("Value"=w2184) -> ()  [unwired: 2 in, 2 out]
            n1091 = Merge Errors(w2200, w2190, w2194) -> (w2217:errorcluster)
          }
        }
      }
      event "Duty Cycle \nDenominator": Value Change {
        n1092 = event-data() -> ()  [unwired: 1 in, 1 out]
        n1093 = call <vilib>:"DAQmx Stop Task.vi"("task/channels in"=w2284, "error in"=w2283) -> ("task out"=w2282:refnum<k21>, "error out"=w2252:errorcluster)  [unwired: 12 in]
        n1094 = property on="473 task" class="DAQmxName (strict)"() -> ("Value"=w2250:refnum<k21>)  [unwired: 2 in, 2 out]
        n1095 = property on="HALF DC" class="Bool (strict)"() -> ("Value"=w2264:bool)  [unwired: 2 in, 2 out]
        n1096 = property on="561 task" class="DAQmxName (strict)"() -> ("Value"=w2251:refnum<k21>)  [unwired: 2 in, 2 out]
        n1097 = call <vilib>:"DAQmx Stop Task.vi"("task/channels in"=w2268, "error in"=w2266) -> ("task out"=w2267:refnum<k21>, "error out"=w2265:errorcluster)  [unwired: 12 in]
        n1098 = call <vilib>:"DAQmx Stop Task.vi"("task/channels in"=w2272, "error in"=w2270) -> ("task out"=w2271:refnum<k21>, "error out"=w2269:errorcluster)  [unwired: 12 in]
        n1099 = flat-sequence {
          tunnel: w2252 -> [w2294]
          tunnel: w2282 -> [w2297]
          tunnel: w2269 -> [w2302]
          tunnel: w2267 -> [w2303]
          tunnel: w2271 -> [w2304]
          tunnel: [w2304] -> w2278
          tunnel: [w2303] -> w2277
          tunnel: [w2302] -> w2276
          tunnel: [w2297] -> w2275
          tunnel: [w2301] -> w2274
          tunnel: [w2300] -> w2273
          tunnel: w2264 -> [w2299]
          tunnel: w2265 -> [w2298]
          tunnel: w2263 -> [w2296]
          tunnel: w2262 -> [w2295]
          tunnel: [w2293] -> w2261
          tunnel: [w2291] -> w2260
          tunnel: [w2290] -> w2259
          tunnel: [w2289] -> w2256
          tunnel: [w2288] -> w2255
          tunnel: w2251 -> [w2287]
          tunnel: w2250 -> [w2286]
          tunnel: [w2453] -> w2285
          tunnel: [w2439] -> w2281
          tunnel: [w2433] -> w2280
          tunnel: [w2429] -> w2279
          tunnel: w2278 -> [w2412]
          tunnel: w2277 -> [w2414]
          tunnel: w2276 -> [w2411]
          tunnel: w2275 -> [w2445]
          tunnel: w2274 -> [w2413]
          tunnel: w2273 -> [w2415]
          tunnel: w2261 -> [w2402]
          tunnel: w2260 -> [w2401]
          tunnel: w2259 -> [w2400]
          tunnel: [w2401] -> w2258
          tunnel: [w2400] -> w2257
          tunnel: w2256 -> [w2398]
          tunnel: w2255 -> [w2399]
          tunnel: [w2399] -> w2254
          tunnel: [w2398] -> w2253
          frame #0 {
            # "Switch between full power and low power\nstates"
            n1100 = property on="Power control" class="Bool (strict)"() -> ("Value"=w2292:bool)  [unwired: 2 in, 2 out]
            n1101 = case shown="False" w2292 {
              tunnel: [w2320 w2367] -> w2301
              tunnel: [w2319 w2369] -> w2300
              tunnel: w2299 -> [w2318 w2357]
              tunnel: w2298 -> [w2317 w2368]
              tunnel: w2296 -> [w2308 w2366]
              tunnel: w2295 -> [w2307 w2365]
              tunnel: w2294 -> [w2310 w2360]
              tunnel: [w2309 w2359] -> w2293
              tunnel: [w2306 w2364] -> w2291
              tunnel: [w2305 w2363] -> w2290
              tunnel: [w2308 w2362] -> w2289
              tunnel: [w2307 w2361] -> w2288
              tunnel: w2287 -> [w2306 w2356]
              tunnel: w2286 -> [w2305 w2355]
              frame False {
                n1102 = case shown="True" w2318 {
                  tunnel: [w2331 w2342] -> w2320
                  tunnel: [w2327 w2346] -> w2319
                  tunnel: w2317 -> [w2325 w2347]
                  tunnel: [w2327 w2346] -> w2311
                  frame True {
                    n1103 = property on="Duty Cycle \nDenominator" class="DigNum (strict)"(error in=w2325) -> (error out=w2324:errorcluster, "Value"=w2326:dbl)  [unwired: 1 in, 1 out]
                    n1104 = property on="Duty Cycle 1\nfull DC" class="Knob (strict)"(error in=w2324) -> (error out=w2338:errorcluster, "Value"=w2337:dbl)  [unwired: 1 in, 1 out]
                    n1105 = Divide(x=w2337, y=w2326) -> (x/y=w2321:dbl)
                    n1106 = Number To Decimal String(number=w2326) -> (decimal integer string=w2328:string)  [unwired: 1 in]
                    n1107 = property on="Duty Cycle 1" class="Knob (strict)"(error in=w2338, "Value"=w2321) -> (error out=w2323:errorcluster)  [unwired: 1 in, 1 out]
                    n1108 = property on="Duty Cycle 1\npreset" class="Knob (strict)"(error in=w2323, "Value"=w2321) -> (error out=w2322:errorcluster)  [unwired: 1 in, 1 out]
                    n1109 = property on="Low Power\nFrames" class="DigNum (strict)"(error in=w2322) -> (error out=w2334:errorcluster, "Value"=w2333:i32)  [unwired: 1 in, 1 out]
                    n1110 = property on="Illuminated Frames" class="DigNum (strict)"(error in=w2334, "Value"=w2333) -> (error out=w2332:errorcluster)  [unwired: 1 in, 1 out]
                    n1111 = Concatenate Strings("1/" ("string"), w2328) -> (w2330:string)
                    n1112 = Less?(x=w2321, y=0.0001) -> (x < y?=w2335:bool)
                    n1113 = case shown="False" w2335 {
                      tunnel: [w2339 0.0001] -> w2327
                      tunnel: w2321 -> [w2339 _]
                      frame False {
                      }
                      frame True {
                      }
                    }
                    n1114 = property on="HALF DC" class="Bool (strict)"(error in=w2332, "BoolText.Text"=w2330) -> (error out=w2331:errorcluster)  [unwired: 1 in, 1 out]
                  }
                  frame False {
                    n1115 = property on="Duty Cycle \nDenominator" class="DigNum (strict)" props=["Value"](error in=w2347) -> (error out=w2350:errorcluster)  [unwired: 1 in, 2 out]
                    n1116 = property on="Duty Cycle 1\npreset" class="Knob (strict)"() -> ("Value"=w2344:dbl)  [unwired: 2 in, 2 out]
                    n1117 = property on="Duty Cycle 1" class="Knob (strict)"(error in=w2350, "Value"=w2344) -> (error out=w2345:errorcluster)  [unwired: 1 in, 1 out]
                    n1118 = property on="Full Power \nFrames" class="DigNum (strict)"(error in=w2345) -> (error out=w2349:errorcluster, "Value"=w2348:i32)  [unwired: 1 in, 1 out]
                    n1119 = property on="Illuminated Frames" class="DigNum (strict)"(error in=w2349, "Value"=w2348) -> (error out=w2343:errorcluster)  [unwired: 1 in, 1 out]
                    n1120 = property on="HALF DC" class="Bool (strict)"(error in=w2343, "BoolText.Text"="1/1" ("Boolean Text.Text")) -> (error out=w2342:errorcluster)  [unwired: 1 in, 1 out]
                    n1121 = Greater Or Equal?(x=w2344, y=1) -> (x >= y?=w2352:bool)
                    n1122 = case shown="False" w2352 {
                      tunnel: [w2353 0.9999] -> w2346
                      tunnel: w2344 -> [w2353 _]
                      frame False {
                      }
                      frame True {
                      }
                    }
                  }
                }
                n1123 = Greater?(x=w2311, y=0.5) -> (0:w2316:bool)
                n1124 = Select(t="WARNING! Laser DC > 0.5\nAFLEX not possible", s=w2316, f="AFLEX conditions\nnormal") -> (s? t:f=w2315:string)
                n1125 = property on="AFLEX warning" class="Bool (strict)"(error in=w2310, "Caption.Text"=w2315, "Value"=w2316) -> (error out=w2309:errorcluster)  [unwired: 1 in, 1 out]
              }
              frame True {
                n1126 = property on="Duty Cycle \nDenominator" class="DigNum (strict)"() -> ("Value"=w2358:dbl)  [unwired: 2 in, 2 out]
                n1127 = case shown="False" w2357 {
                  tunnel: w2360 -> [w2378 w2382]
                  tunnel: [w2377 w2381] -> w2359
                  tunnel: w2358 -> [_ w2380]
                  frame False {
                    n1128 = property on="HALF DC" class="Bool (strict)"(error in=w2378, "BoolText.Text"="1/1" ("Boolean Text.Text")) -> (error out=w2377:errorcluster)  [unwired: 1 in, 1 out]
                  }
                  frame True {
                    n1129 = Number To Decimal String(number=w2380) -> (decimal integer string=w2384:string)  [unwired: 1 in]
                    n1130 = Concatenate Strings("1/" ("string"), w2384) -> (w2379:string)
                    n1131 = property on="HALF DC" class="Bool (strict)"(error in=w2382, "BoolText.Text"=w2379) -> (error out=w2381:errorcluster)  [unwired: 1 in, 1 out]
                  }
                }
                n1132 = property on="Duty Cycle 1" class="Knob (strict)"(error in=w2368) -> (error out=w2367:errorcluster, "Value"=w2369:dbl)  [unwired: 1 in, 1 out]
                n1133 = property on="Level at max 561nm (0-5V)" class="DigNum (strict)"(error in=w2366) -> (error out=w2374:errorcluster, "Value"=w2373:dbl)  [unwired: 1 in, 1 out]
                n1134 = case shown="False" w2357 {
                  tunnel: w2358 -> [_ w2396]
                  tunnel: [w2391 w2394] -> w2375
                  tunnel: w2373 -> [w2391 w2392]
                  frame False {
                  }
                  frame True {
                    n1135 = Divide(x=1.0, y=w2396) -> (x/y=w2393:dbl)
                    n1136 = Multiply(x=w2393, y=w2392) -> (x*y=w2394:dbl)
                  }
                }
                n1137 = property on="Level at max 473nm (0-5V)" class="DigNum (strict)"(error in=w2365) -> (error out=w2371:errorcluster, "Value"=w2370:dbl)  [unwired: 1 in, 1 out]
                n1138 = case shown="True" w2357 {
                  tunnel: w2358 -> [_ w2390]
                  tunnel: [w2385 w2388] -> w2372
                  tunnel: w2370 -> [w2385 w2386]
                  frame False {
                  }
                  frame True {
                    n1139 = Divide(x=1.0, y=w2390) -> (x/y=w2387:dbl)
                    n1140 = Multiply(x=w2387, y=w2386) -> (x*y=w2388:dbl)
                  }
                }
                n1141 = call-poly <vilib>:"DAQmx Write.vi"("task/channels in"=w2356, "data"=w2375, "error in"=w2374) -> ("task out"=w2364:refnum<k21>, "error out"=w2362:errorcluster)  [unwired: 10 in, 1 out]
                n1142 = call-poly <vilib>:"DAQmx Write.vi"("task/channels in"=w2355, "data"=w2372, "error in"=w2371) -> ("task out"=w2363:refnum<k21>, "error out"=w2361:errorcluster)  [unwired: 10 in, 1 out]
              }
            }
          }
          frame #1 {
            (unwired) 0.05 ("x")
            (unwired) 0.05 ("y")
            # "Force system to calculate from updated values"
            # "Trigger"
            # "473 nm"
            # "561 nm"
            n1143 = local read "First frame\ndelay (ms)"() -> (w2449:dbl)
            n1144 = local read "Frequency 1"() -> (w2405:dbl)
            n1145 = local read "Duty Cycle camera"() -> (w2447:dbl)
            n1146 = property on="Continous ill" class="Bool (strict)"() -> ("Value"=w2410:bool)  [unwired: 2 in, 2 out]
            n1147 = local read "Frame rate"() -> (w2406:dbl)
            n1148 = property class="DAQmx Channel"(reference=w2412, error in=w2411, "CO.Pulse.Freq"=w2406, "CO.Pulse.DutyCyc"=w2447) -> (reference out=w2440:refnum<k21>, error out=w2438:errorcluster)
            n1149 = Divide(x=w2449, y=1000) -> (x/y=w2420:dbl)
            n1150 = Multiply(x=w2406, y=w2420) -> (x*y=w2451:dbl)
            n1151 = To Long Integer(number=w2451) -> (32bit integer=w2435:i32)
            n1152 = Reciprocal(x=w2406) -> (1/x=w2450:dbl)
            n1153 = local read "Illuminated Frames"() -> (w2409:i32)
            n1154 = Multiply(x=w2435, y=w2450) -> (x*y=w2441:dbl)
            n1155 = local read "Finishing frames"() -> (w2436:i32)
            n1156 = property on="Initial calculated\ndelay (frames)" class="DigNum (strict)"("Value"=w2451) -> ()  [unwired: 2 in, 2 out]
            n1157 = property on="delay\ncompensation" class="DigNum (strict)"() -> ("Value"=w2397:dbl)  [unwired: 2 in, 2 out]
            n1158 = Multiply(x=w2441, y=1000) -> (x*y=w2446:dbl)
            n1159 = property on="Laser delay (ms)" class="DigNum (strict)"("Value"=w2446) -> ()  [unwired: 2 in, 2 out]
            n1160 = Add(x=w2409, y=w2435) -> (x+y=w2424:i32)
            n1161 = Divide(x=w2409, y=2) -> (x/y=w2425:dbl)
            n1162 = Subtract(x=w2420, y=w2397) -> (x-y=w2422:dbl)
            n1163 = Multiply(x=w2397, y=w2406) -> (x*y=w2417:dbl)
            n1164 = To Long Integer(number=w2425) -> (32bit integer=w2408:i32)
            n1165 = case shown="False" w2410 {
              tunnel: [w2459 w2479] -> w2404
              tunnel: w2406 -> [w2461 w2480]
              tunnel: w2405 -> [w2462 _]
              tunnel: w2409 -> [w2455 w2484]
              tunnel: [w2456 1] -> w2407
              tunnel: [w2454 w2481] -> _
              tunnel: w2408 -> [w2458 _]
              tunnel: [w2460 0.0] -> w2403
              frame False {
                n1166 = property on="Frequency 1" class="Knob (strict)" props=["Value"]() -> ()  [unwired: 2 in, 3 out]
                n1167 = property on="Pulsed" class="Bool (strict)"() -> ("Value"=w2457:bool)  [unwired: 2 in, 2 out]
                n1168 = local read "Duty Cycle 1\npreset"() -> (w2454:dbl)
                n1169 = case shown="False" w2457 {
                  tunnel: w2462 -> [w2470 _]
                  tunnel: w2461 -> [w2469 w2476]
                  tunnel: w2454 -> [_ _]
                  tunnel: [w2465 0.0] -> w2460
                  tunnel: [w2464 w2476] -> w2459
                  tunnel: w2458 -> [w2463 _]
                  tunnel: [w2463 w2475] -> w2456
                  tunnel: w2455 -> [_ w2475]
                  frame False {
                    n1170 = property on="Link rates" class="Bool (strict)"() -> ("Value"=w2468:bool)  [unwired: 2 in, 2 out]
                    n1171 = case shown="True" w2468 {
                      tunnel: [w2471 w2472] -> w2464
                      tunnel: w2469 -> [_ w2474]
                      tunnel: w2470 -> [w2471 _]
                      frame False {
                      }
                      frame True {
                        n1172 = Divide(x=w2474, y=2) -> (x/y=w2472:dbl)
                        n1173 = property on="Frequency 1" class="Knob (strict)"("Value"=w2472) -> ()  [unwired: 2 in, 2 out]
                      }
                    }
                    n1174 = Multiply(x=w2464, y=2) -> (x*y=w2467:dbl)
                    n1175 = Reciprocal(x=w2467) -> (1/x=w2465:dbl)
                  }
                  frame True {
                  }
                }
                n1176 = property on="Duty Cycle 1" class="Knob (strict)"("Value"=w2454) -> ()  [unwired: 2 in, 2 out]
                n1177 = property on="Duty Cycle 1\npreset" class="Knob (strict)"("Value"=w2454) -> ()  [unwired: 2 in, 2 out]
              }
              frame True {
                w2481 = 0.9999 ("x")
                n1178 = Reciprocal(x=w2480) -> (1/x=w2485:dbl)
                n1179 = Multiply(x=w2485, y=w2484) -> (x*y=w2482:dbl)
                n1180 = property on="Duty Cycle 1" class="Knob (strict)"("Value"=w2481) -> ()  [unwired: 2 in, 2 out]
                n1181 = Divide(x=w2481, y=w2482) -> (x/y=w2479:dbl)
                n1182 = property on="Frequency 1" class="Knob (strict)"("Value"=w2479) -> ()  [unwired: 2 in, 2 out]
              }
            }
            n1183 = property class="DAQmx Channel"(reference=w2414, error in=w2413, "CO.Pulse.Freq"=w2404, "CO.Pulse.DutyCyc"=w2415, "CO.Pulse.Freq.InitialDelay"=w2441) -> (reference out=w2430:refnum<k21>, error out=w2428:errorcluster)
            n1184 = Add(x=w2441, y=w2403) -> (x+y=w2442:dbl)
            n1185 = property class="DAQmx Channel"(reference=w2445, error in=w2402, "CO.Pulse.Freq"=w2404, "CO.Pulse.DutyCyc"=w2415, "CO.Pulse.Freq.InitialDelay"=w2442) -> (reference out=w2434:refnum<k21>, error out=w2432:errorcluster)
            n1186 = Multiply(x=w2403, y=1000) -> (x*y=w2443:dbl)
            n1187 = property on="Initial delay\n473 nm (ms)" class="DigNum (strict)"("Value"=w2443) -> ()  [unwired: 2 in, 2 out]
            n1188 = Add(x=w2436, y=w2424) -> (x+y=w2416:i32)
            n1189 = property class="DAQmx Timing"(reference=w2440, error in=w2438, "SampQuant.SampPerChan"=w2416) -> (reference out=w2439:refnum<k21>, error out=w2437:errorcluster)
            n1190 = Multiply(x=w2406, y=w2422) -> (x*y=w2423:dbl)
            n1191 = To Long Integer(number=w2417) -> (32bit integer=w2418:i32)
            n1192 = Subtract(x=w2416, y=w2418) -> (x-y=w2419:i32)
            n1193 = To Long Integer(number=w2423) -> (32bit integer=w2421:i32)
            n1194 = property on="Trigger pulses" class="DigNum (strict)"("Value"=w2416) -> ()  [unwired: 2 in, 2 out]
            n1195 = property class="DAQmx Timing"(reference=w2430, error in=w2428, "SampQuant.SampPerChan"=w2407) -> (reference out=w2429:refnum<k21>, error out=w2427:errorcluster)
            n1196 = property class="DAQmx Timing"(reference=w2434, error in=w2432, "SampQuant.SampPerChan"=w2407) -> (reference out=w2433:refnum<k21>, error out=w2431:errorcluster)
            n1197 = property on="Frames to acquire" class="DigNum (strict)"("Value"=w2419) -> ()  [unwired: 2 in, 2 out]
            n1198 = property on="Laser pulses" class="DigNum (strict)"("Value"=w2407) -> ()  [unwired: 2 in, 2 out]
            n1199 = property on="Initial frames" class="DigNum (strict)"("Value"=w2421) -> ()  [unwired: 2 in, 2 out]
            n1200 = Merge Errors(w2437, w2427, w2431) -> (w2453:errorcluster)
          }
        }
      }
      event "Populate": Value Change {
        n1201 = event-data() -> ()  [unwired: 1 in, 6 out]
        n1202 = call <vilib>:"DAQmx Stop Task.vi"("task/channels in"=w2506, "error in"=w2505) -> ("task out"=w2504:refnum<k21>, "error out"=w2503:errorcluster)  [unwired: 12 in]
        n1203 = call <vilib>:"DAQmx Stop Task.vi"("task/channels in"=w2489, "error in"=w2487) -> ("task out"=w2488:refnum<k21>, "error out"=w2486:errorcluster)  [unwired: 12 in]
        n1204 = call <vilib>:"DAQmx Stop Task.vi"("task/channels in"=w2493, "error in"=w2491) -> ("task out"=w2492:refnum<k21>, "error out"=w2490:errorcluster)  [unwired: 12 in]
        n1205 = flat-sequence {
          tunnel: w2503 -> [w2513]
          tunnel: w2504 -> [w2512]
          tunnel: w2490 -> [w2514]
          tunnel: w2488 -> [w2515]
          tunnel: w2492 -> [w2516]
          tunnel: [w2516] -> w2499
          tunnel: [w2515] -> w2498
          tunnel: [w2514] -> w2497
          tunnel: [w2512] -> w2496
          tunnel: [w2513] -> w2495
          tunnel: [w2508] -> w2494
          tunnel: w2486 -> [w2511]
          tunnel: [w2569] -> w2507
          tunnel: [w2554] -> w2502
          tunnel: [w2548] -> w2501
          tunnel: [w2544] -> w2500
          tunnel: w2499 -> [w2528]
          tunnel: w2498 -> [w2530]
          tunnel: w2497 -> [w2527]
          tunnel: w2496 -> [w2561]
          tunnel: w2495 -> [w2560]
          tunnel: w2494 -> [w2529]
          frame #0 {
            # "Populate Low Power Frames with content of Full Power \nFrames before sending it to Illuminated Frames"
            n1206 = property on="Full Power \nFrames" class="DigNum (strict)"(error in=w2511) -> (error out=w2509:errorcluster, "Value"=w2510:i32)  [unwired: 1 in, 1 out]
            n1207 = property on="Low Power\nFrames" class="DigNum (strict)"(error in=w2509, "Value"=w2510) -> (error out=w2508:errorcluster)  [unwired: 1 in, 1 out]
          }
          frame #1 {
            (unwired) 0.05 ("x")
            (unwired) 0.05 ("y")
            # "Force system to calculate from updated values"
            # "Trigger"
            # "473 nm"
            # "561 nm"
            n1208 = local read "First frame\ndelay (ms)"() -> (w2565:dbl)
            n1209 = local read "Duty Cycle camera"() -> (w2563:dbl)
            n1210 = local read "Frame rate"() -> (w2522:dbl)
            n1211 = property on="Continous ill" class="Bool (strict)"() -> ("Value"=w2526:bool)  [unwired: 2 in, 2 out]
            n1212 = property on="Frequency 1" class="Knob (strict)"() -> ("Value"=w2524:dbl)  [unwired: 2 in, 2 out]
            n1213 = property class="DAQmx Channel"(reference=w2528, error in=w2527, "CO.Pulse.Freq"=w2522, "CO.Pulse.DutyCyc"=w2563) -> (reference out=w2555:refnum<k21>, error out=w2553:errorcluster)
            n1214 = Divide(x=w2565, y=1000) -> (x/y=w2535:dbl)
            n1215 = Multiply(x=w2522, y=w2535) -> (x*y=w2567:dbl)
            n1216 = To Long Integer(number=w2567) -> (32bit integer=w2550:i32)
            n1217 = Reciprocal(x=w2522) -> (1/x=w2566:dbl)
            n1218 = local read "Illuminated Frames"() -> (w2518:i32)
            n1219 = Multiply(x=w2550, y=w2566) -> (x*y=w2556:dbl)
            n1220 = local read "Finishing frames"() -> (w2551:i32)
            n1221 = property on="Initial calculated\ndelay (frames)" class="DigNum (strict)"("Value"=w2567) -> ()  [unwired: 2 in, 2 out]
            n1222 = property on="delay\ncompensation" class="DigNum (strict)"() -> ("Value"=w2517:dbl)  [unwired: 2 in, 2 out]
            n1223 = Multiply(x=w2556, y=1000) -> (x*y=w2562:dbl)
            n1224 = property on="Laser delay (ms)" class="DigNum (strict)"("Value"=w2562) -> ()  [unwired: 2 in, 2 out]
            n1225 = Add(x=w2518, y=w2550) -> (x+y=w2539:i32)
            n1226 = Subtract(x=w2535, y=w2517) -> (x-y=w2537:dbl)
            n1227 = Multiply(x=w2517, y=w2522) -> (x*y=w2532:dbl)
            n1228 = Divide(x=w2518, y=2) -> (x/y=w2540:dbl)
            n1229 = Add(x=w2551, y=w2539) -> (x+y=w2531:i32)
            n1230 = property class="DAQmx Timing"(reference=w2555, error in=w2553, "SampQuant.SampPerChan"=w2531) -> (reference out=w2554:refnum<k21>, error out=w2552:errorcluster)
            n1231 = Multiply(x=w2522, y=w2537) -> (x*y=w2538:dbl)
            n1232 = To Long Integer(number=w2532) -> (32bit integer=w2533:i32)
            n1233 = To Long Integer(number=w2540) -> (32bit integer=w2520:i32)
            n1234 = case shown="False" w2526 {
              tunnel: [w2577 w2597] -> w2523
              tunnel: [w2570 1] -> w2519
              tunnel: [w2575 w2598] -> w2521
              tunnel: [w2578 0.0] -> w2525
              tunnel: w2522 -> [w2573 w2595]
              tunnel: w2524 -> [w2574 _]
              tunnel: w2520 -> [w2572 _]
              tunnel: w2518 -> [w2571 w2594]
              frame False {
                n1235 = property on="Pulsed" class="Bool (strict)"() -> ("Value"=w2576:bool)  [unwired: 2 in, 2 out]
                n1236 = property on="Duty Cycle 1\npreset" class="Knob (strict)"() -> ("Value"=w2575:dbl)  [unwired: 2 in, 2 out]
                n1237 = case shown="False" w2576 {
                  tunnel: w2575 -> [_ _]
                  tunnel: [w2583 0.0] -> w2578
                  tunnel: [w2582 w2592] -> w2577
                  tunnel: w2574 -> [w2581 _]
                  tunnel: w2573 -> [w2580 w2592]
                  tunnel: w2572 -> [w2579 _]
                  tunnel: w2571 -> [_ w2591]
                  tunnel: [w2579 w2591] -> w2570
                  frame False {
                    n1238 = property on="Link rates" class="Bool (strict)"() -> ("Value"=w2586:bool)  [unwired: 2 in, 2 out]
                    n1239 = case shown="True" w2586 {
                      tunnel: [w2587 w2589] -> w2582
                      tunnel: w2581 -> [w2587 _]
                      tunnel: w2580 -> [_ w2588]
                      frame False {
                      }
                      frame True {
                        n1240 = Divide(x=w2588, y=2) -> (x/y=w2589:dbl)
                        n1241 = property on="Frequency 1" class="Knob (strict)"("Value"=w2589) -> ()  [unwired: 2 in, 2 out]
                      }
                    }
                    n1242 = Multiply(x=w2582, y=2) -> (x*y=w2585:dbl)
                    n1243 = Reciprocal(x=w2585) -> (1/x=w2583:dbl)
                  }
                  frame True {
                  }
                }
                n1244 = property on="Duty Cycle 1" class="Knob (strict)"("Value"=w2575) -> ()  [unwired: 2 in, 2 out]
              }
              frame True {
                w2598 = 0.9999 ("x")
                n1245 = Reciprocal(x=w2595) -> (1/x=w2601:dbl)
                n1246 = Multiply(x=w2601, y=w2594) -> (x*y=w2599:dbl)
                n1247 = property on="Duty Cycle 1" class="Knob (strict)"("Value"=w2598) -> ()  [unwired: 2 in, 2 out]
                n1248 = Divide(x=w2598, y=w2599) -> (x/y=w2597:dbl)
                n1249 = property on="Frequency 1" class="Knob (strict)"("Value"=w2597) -> ()  [unwired: 2 in, 2 out]
              }
            }
            n1250 = property class="DAQmx Channel"(reference=w2530, error in=w2529, "CO.Pulse.Freq"=w2523, "CO.Pulse.DutyCyc"=w2521, "CO.Pulse.Freq.InitialDelay"=w2556) -> (reference out=w2545:refnum<k21>, error out=w2543:errorcluster)
            n1251 = Add(x=w2556, y=w2525) -> (x+y=w2557:dbl)
            n1252 = property class="DAQmx Channel"(reference=w2561, error in=w2560, "CO.Pulse.Freq"=w2523, "CO.Pulse.DutyCyc"=w2521, "CO.Pulse.Freq.InitialDelay"=w2557) -> (reference out=w2549:refnum<k21>, error out=w2547:errorcluster)
            n1253 = Multiply(x=w2525, y=1000) -> (x*y=w2558:dbl)
            n1254 = property on="Initial delay\n473 nm (ms)" class="DigNum (strict)"("Value"=w2558) -> ()  [unwired: 2 in, 2 out]
            n1255 = Subtract(x=w2531, y=w2533) -> (x-y=w2534:i32)
            n1256 = To Long Integer(number=w2538) -> (32bit integer=w2536:i32)
            n1257 = property on="Frames to acquire" class="DigNum (strict)"("Value"=w2534) -> ()  [unwired: 2 in, 2 out]
            n1258 = property on="Initial frames" class="DigNum (strict)"("Value"=w2536) -> ()  [unwired: 2 in, 2 out]
            n1259 = property on="Trigger pulses" class="DigNum (strict)"("Value"=w2531) -> ()  [unwired: 2 in, 2 out]
            n1260 = property class="DAQmx Timing"(reference=w2545, error in=w2543, "SampQuant.SampPerChan"=w2519) -> (reference out=w2544:refnum<k21>, error out=w2542:errorcluster)
            n1261 = property class="DAQmx Timing"(reference=w2549, error in=w2547, "SampQuant.SampPerChan"=w2519) -> (reference out=w2548:refnum<k21>, error out=w2546:errorcluster)
            n1262 = property on="Laser pulses" class="DigNum (strict)"("Value"=w2519) -> ()  [unwired: 2 in, 2 out]
            n1263 = Merge Errors(w2552, w2542, w2546) -> (w2569:errorcluster)
          }
        }
      }
      event "Duty Cycle camera": Value Change {
        (unwired) 0.05 ("x")
        (unwired) 0.05 ("y")
        # "These operations have been moved to the Settings pane.\nThus there is no need for rigorous control of \ncontinous/pulsed mode state"
        # "Trigger"
        # "473 nm"
        # "561 nm"
        n1264 = event-data() -> ()  [unwired: 1 in, 1 out]
        n1265 = call <vilib>:"DAQmx Stop Task.vi"("task/channels in"=w2659, "error in"=w2658) -> ("task out"=w2650:refnum<k21>, "error out"=w2606:errorcluster)  [unwired: 12 in]
        n1266 = call <vilib>:"DAQmx Stop Task.vi"("task/channels in"=w2663, "error in"=w2661) -> ("task out"=w2652:refnum<k21>, "error out"=w2611:errorcluster)  [unwired: 12 in]
        n1267 = call <vilib>:"DAQmx Stop Task.vi"("task/channels in"=w2664, "error in"=w2660) -> ("task out"=w2653:refnum<k21>, "error out"=w2613:errorcluster)  [unwired: 12 in]
        n1268 = property on="Frequency 1" class="Knob (strict)"(error in=w2611) -> (error out=w2610:errorcluster, "Value"=w2612:dbl)  [unwired: 1 in, 1 out]
        n1269 = property on="Frame rate" class="Knob (strict)"(error in=w2613) -> (error out=w2615:errorcluster, "Value"=w2614:dbl)  [unwired: 1 in, 1 out]
        n1270 = Multiply(x=w2612, y=2) -> (x*y=w2648:dbl)
        n1271 = property on="First frame\ndelay (ms)" class="DigNum (strict)"() -> ("Value"=w2607:dbl)  [unwired: 2 in, 2 out]
        n1272 = property on="Duty Cycle camera" class="Knob (strict)"(error in=w2615) -> (error out=w2605:errorcluster, "Value"=w2604:dbl)  [unwired: 1 in, 1 out]
        n1273 = property on="Duty Cycle 1" class="Knob (strict)"(error in=w2610) -> (error out=w2608:errorcluster, "Value"=w2609:dbl)  [unwired: 1 in, 1 out]
        n1274 = Reciprocal(x=w2648) -> (1/x=w2646:dbl)
        n1275 = property on="Duty Cycle camera 2" class="Knob (strict)"(error in=w2605, "Value"=w2604) -> (error out=w2603:errorcluster)  [unwired: 1 in, 1 out]
        n1276 = Multiply(x=w2646, y=1000) -> (x*y=w2645:dbl)
        n1277 = property class="DAQmx Channel"(reference=w2653, error in=w2603, "CO.Pulse.Freq"=w2614, "CO.Pulse.DutyCyc"=w2604) -> (reference out=w2642:refnum<k21>, error out=w2640:errorcluster)
        n1278 = Divide(x=w2607, y=1000) -> (x/y=w2621:dbl)
        n1279 = property on="Initial delay\n473 nm (ms)" class="DigNum (strict)"("Value"=w2645) -> ()  [unwired: 2 in, 2 out]
        n1280 = Multiply(x=w2614, y=w2621) -> (x*y=w2656:dbl)
        n1281 = To Long Integer(number=w2656) -> (32bit integer=w2637:i32)
        n1282 = Reciprocal(x=w2614) -> (1/x=w2655:dbl)
        n1283 = property on="delay\ncompensation" class="DigNum (strict)"() -> ("Value"=w2602:dbl)  [unwired: 2 in, 2 out]
        n1284 = local read "Illuminated Frames"() -> (w2624:i32)
        n1285 = Multiply(x=w2637, y=w2655) -> (x*y=w2643:dbl)
        n1286 = Add(x=w2643, y=w2646) -> (x+y=w2644:dbl)
        n1287 = property class="DAQmx Channel"(reference=w2652, error in=w2608, "CO.Pulse.Freq"=w2612, "CO.Pulse.DutyCyc"=w2609, "CO.Pulse.Freq.InitialDelay"=w2643) -> (reference out=w2632:refnum<k21>, error out=w2630:errorcluster)
        n1288 = property class="DAQmx Channel"(reference=w2650, error in=w2606, "CO.Pulse.Freq"=w2612, "CO.Pulse.DutyCyc"=w2609, "CO.Pulse.Freq.InitialDelay"=w2644) -> (reference out=w2636:refnum<k21>, error out=w2634:errorcluster)
        n1289 = local read "Finishing frames"() -> (w2638:i32)
        n1290 = property on="Initial calculated\ndelay (frames)" class="DigNum (strict)"("Value"=w2656) -> ()  [unwired: 2 in, 2 out]
        n1291 = Multiply(x=w2643, y=1000) -> (x*y=w2651:dbl)
        n1292 = property on="Laser delay (ms)" class="DigNum (strict)"("Value"=w2651) -> ()  [unwired: 2 in, 2 out]
        n1293 = Add(x=w2624, y=w2637) -> (x+y=w2626:i32)
        n1294 = Subtract(x=w2621, y=w2602) -> (x-y=w2622:dbl)
        n1295 = Multiply(x=w2602, y=w2614) -> (x*y=w2617:dbl)
        n1296 = Divide(x=w2624, y=2) -> (x/y=w2627:dbl)
        n1297 = Add(x=w2638, y=w2626) -> (x+y=w2616:i32)
        n1298 = property class="DAQmx Timing"(reference=w2642, error in=w2640, "SampQuant.SampPerChan"=w2616) -> (reference out=w2641:refnum<k21>, error out=w2639:errorcluster)
        n1299 = Multiply(x=w2614, y=w2622) -> (x*y=w2623:dbl)
        n1300 = To Long Integer(number=w2617) -> (32bit integer=w2618:i32)
        n1301 = To Long Integer(number=w2623) -> (32bit integer=w2620:i32)
        n1302 = Subtract(x=w2616, y=w2618) -> (x-y=w2619:i32)
        n1303 = To Long Integer(number=w2627) -> (32bit integer=w2625:i32)
        n1304 = property on="Initial frames" class="DigNum (strict)"("Value"=w2620) -> ()  [unwired: 2 in, 2 out]
        n1305 = property on="Frames to acquire" class="DigNum (strict)"("Value"=w2619) -> ()  [unwired: 2 in, 2 out]
        n1306 = property class="DAQmx Timing"(reference=w2632, error in=w2630, "SampQuant.SampPerChan"=w2625) -> (reference out=w2631:refnum<k21>, error out=w2629:errorcluster)
        n1307 = property on="Trigger pulses" class="DigNum (strict)"("Value"=w2616) -> ()  [unwired: 2 in, 2 out]
        n1308 = property class="DAQmx Timing"(reference=w2636, error in=w2634, "SampQuant.SampPerChan"=w2625) -> (reference out=w2635:refnum<k21>, error out=w2633:errorcluster)
        n1309 = property on="Laser pulses" class="DigNum (strict)"("Value"=w2625) -> ()  [unwired: 2 in, 2 out]
        n1310 = Merge Errors(w2639, w2629, w2633) -> (w2662:errorcluster)
      }
      event "First frame\ndelay (ms)": Value Change {
        (unwired) 0.05 ("x")
        (unwired) 0.05 ("y")
        # "Trigger"
        # "473 nm"
        # "561 nm"
        n1311 = event-data() -> ()  [unwired: 1 in, 1 out]
        n1312 = property on="Continous ill" class="Bool (strict)"() -> ("Value"=w2674:bool)  [unwired: 2 in, 2 out]
        n1313 = call <vilib>:"DAQmx Stop Task.vi"("task/channels in"=w2718, "error in"=w2717) -> ("task out"=w2705:refnum<k21>, "error out"=w2704:errorcluster)  [unwired: 12 in]
        n1314 = property on="Frequency 1" class="Knob (strict)"() -> ("Value"=w2672:dbl)  [unwired: 2 in, 2 out]
        n1315 = call <vilib>:"DAQmx Stop Task.vi"("task/channels in"=w2723, "error in"=w2719) -> ("task out"=w2711:refnum<k21>, "error out"=w2710:errorcluster)  [unwired: 12 in]
        n1316 = call <vilib>:"DAQmx Stop Task.vi"("task/channels in"=w2722, "error in"=w2720) -> ("task out"=w2708:refnum<k21>, "error out"=w2707:errorcluster)  [unwired: 12 in]
        n1317 = local read "First frame\ndelay (ms)"() -> (w2713:dbl)
        n1318 = local read "Duty Cycle camera"() -> (w2709:dbl)
        n1319 = local read "Frame rate"() -> (w2670:dbl)
        n1320 = property class="DAQmx Channel"(reference=w2711, error in=w2710, "CO.Pulse.Freq"=w2670, "CO.Pulse.DutyCyc"=w2709) -> (reference out=w2699:refnum<k21>, error out=w2697:errorcluster)
        n1321 = Divide(x=w2713, y=1000) -> (x/y=w2679:dbl)
        n1322 = Multiply(x=w2670, y=w2679) -> (x*y=w2715:dbl)
        n1323 = To Long Integer(number=w2715) -> (32bit integer=w2694:i32)
        n1324 = Reciprocal(x=w2670) -> (1/x=w2714:dbl)
        n1325 = property on="delay\ncompensation" class="DigNum (strict)"() -> ("Value"=w2665:dbl)  [unwired: 2 in, 2 out]
        n1326 = local read "Illuminated Frames"() -> (w2667:i32)
        n1327 = Multiply(x=w2694, y=w2714) -> (x*y=w2700:dbl)
        n1328 = local read "Finishing frames"() -> (w2695:i32)
        n1329 = property on="Initial calculated\ndelay (frames)" class="DigNum (strict)"("Value"=w2715) -> ()  [unwired: 2 in, 2 out]
        n1330 = Multiply(x=w2700, y=1000) -> (x*y=w2706:dbl)
        n1331 = property on="Laser delay (ms)" class="DigNum (strict)"("Value"=w2706) -> ()  [unwired: 2 in, 2 out]
        n1332 = Add(x=w2667, y=w2694) -> (x+y=w2683:i32)
        n1333 = Subtract(x=w2679, y=w2665) -> (x-y=w2681:dbl)
        n1334 = Multiply(x=w2665, y=w2670) -> (x*y=w2676:dbl)
        n1335 = Add(x=w2695, y=w2683) -> (x+y=w2675:i32)
        n1336 = Divide(x=w2667, y=2) -> (x/y=w2684:dbl)
        n1337 = To Long Integer(number=w2684) -> (32bit integer=w2669:i32)
        n1338 = case shown="False" w2674 {
          tunnel: [w2731 w2751] -> w2671
          tunnel: [w2724 1] -> w2668
          tunnel: [w2729 w2752] -> w2666
          tunnel: [w2732 0.0] -> w2673
          tunnel: w2670 -> [w2727 w2749]
          tunnel: w2672 -> [w2728 _]
          tunnel: w2669 -> [w2726 _]
          tunnel: w2667 -> [w2725 w2748]
          frame False {
            n1339 = property on="Pulsed" class="Bool (strict)"() -> ("Value"=w2730:bool)  [unwired: 2 in, 2 out]
            n1340 = property on="Duty Cycle 1\npreset" class="Knob (strict)"() -> ("Value"=w2729:dbl)  [unwired: 2 in, 2 out]
            n1341 = case shown="False" w2730 {
              tunnel: w2729 -> [_ _]
              tunnel: [w2737 0.0] -> w2732
              tunnel: [w2736 w2746] -> w2731
              tunnel: w2728 -> [w2735 _]
              tunnel: w2727 -> [w2734 w2746]
              tunnel: w2726 -> [w2733 _]
              tunnel: w2725 -> [_ w2745]
              tunnel: [w2733 w2745] -> w2724
              frame False {
                n1342 = property on="Link rates" class="Bool (strict)"() -> ("Value"=w2740:bool)  [unwired: 2 in, 2 out]
                n1343 = case shown="True" w2740 {
                  tunnel: [w2741 w2743] -> w2736
                  tunnel: w2735 -> [w2741 _]
                  tunnel: w2734 -> [_ w2742]
                  frame False {
                  }
                  frame True {
                    n1344 = Divide(x=w2742, y=2) -> (x/y=w2743:dbl)
                    n1345 = property on="Frequency 1" class="Knob (strict)"("Value"=w2743) -> ()  [unwired: 2 in, 2 out]
                  }
                }
                n1346 = Multiply(x=w2736, y=2) -> (x*y=w2739:dbl)
                n1347 = Reciprocal(x=w2739) -> (1/x=w2737:dbl)
              }
              frame True {
              }
            }
            n1348 = property on="Duty Cycle 1" class="Knob (strict)"("Value"=w2729) -> ()  [unwired: 2 in, 2 out]
          }
          frame True {
            w2752 = 0.9999 ("x")
            n1349 = Reciprocal(x=w2749) -> (1/x=w2755:dbl)
            n1350 = Multiply(x=w2755, y=w2748) -> (x*y=w2753:dbl)
            n1351 = property on="Duty Cycle 1" class="Knob (strict)"("Value"=w2752) -> ()  [unwired: 2 in, 2 out]
            n1352 = Divide(x=w2752, y=w2753) -> (x/y=w2751:dbl)
            n1353 = property on="Frequency 1" class="Knob (strict)"("Value"=w2751) -> ()  [unwired: 2 in, 2 out]
          }
        }
        n1354 = Add(x=w2700, y=w2673) -> (x+y=w2701:dbl)
        n1355 = Multiply(x=w2673, y=1000) -> (x*y=w2702:dbl)
        n1356 = property class="DAQmx Channel"(reference=w2708, error in=w2707, "CO.Pulse.Freq"=w2671, "CO.Pulse.DutyCyc"=w2666, "CO.Pulse.Freq.InitialDelay"=w2700) -> (reference out=w2689:refnum<k21>, error out=w2687:errorcluster)
        n1357 = property class="DAQmx Channel"(reference=w2705, error in=w2704, "CO.Pulse.Freq"=w2671, "CO.Pulse.DutyCyc"=w2666, "CO.Pulse.Freq.InitialDelay"=w2701) -> (reference out=w2693:refnum<k21>, error out=w2691:errorcluster)
        n1358 = property on="Initial delay\n473 nm (ms)" class="DigNum (strict)"("Value"=w2702) -> ()  [unwired: 2 in, 2 out]
        n1359 = property class="DAQmx Timing"(reference=w2699, error in=w2697, "SampQuant.SampPerChan"=w2675) -> (reference out=w2698:refnum<k21>, error out=w2696:errorcluster)
        n1360 = Multiply(x=w2670, y=w2681) -> (x*y=w2682:dbl)
        n1361 = To Long Integer(number=w2676) -> (32bit integer=w2677:i32)
        n1362 = To Long Integer(number=w2682) -> (32bit integer=w2680:i32)
        n1363 = Subtract(x=w2675, y=w2677) -> (x-y=w2678:i32)
        n1364 = property on="Frames to acquire" class="DigNum (strict)"("Value"=w2678) -> ()  [unwired: 2 in, 2 out]
        n1365 = property on="Initial frames" class="DigNum (strict)"("Value"=w2680) -> ()  [unwired: 2 in, 2 out]
        n1366 = property class="DAQmx Timing"(reference=w2689, error in=w2687, "SampQuant.SampPerChan"=w2668) -> (reference out=w2688:refnum<k21>, error out=w2686:errorcluster)
        n1367 = property on="Trigger pulses" class="DigNum (strict)"("Value"=w2675) -> ()  [unwired: 2 in, 2 out]
        n1368 = property on="Laser pulses" class="DigNum (strict)"("Value"=w2668) -> ()  [unwired: 2 in, 2 out]
        n1369 = property class="DAQmx Timing"(reference=w2693, error in=w2691, "SampQuant.SampPerChan"=w2668) -> (reference out=w2692:refnum<k21>, error out=w2690:errorcluster)
        n1370 = Merge Errors(w2696, w2686, w2690) -> (w2721:errorcluster)
      }
      event "Finishing frames": Value Change {
        (unwired) 0.05 ("x")
        (unwired) 0.05 ("y")
        # "Trigger"
        # "473 nm"
        # "561 nm"
        n1371 = event-data() -> ()  [unwired: 1 in, 1 out]
        n1372 = call <vilib>:"DAQmx Stop Task.vi"("task/channels in"=w2809, "error in"=w2808) -> ("task out"=w2796:refnum<k21>, "error out"=w2795:errorcluster)  [unwired: 12 in]
        n1373 = property on="Continous ill" class="Bool (strict)"() -> ("Value"=w2765:bool)  [unwired: 2 in, 2 out]
        n1374 = property on="Frequency 1" class="Knob (strict)"() -> ("Value"=w2764:dbl)  [unwired: 2 in, 2 out]
        n1375 = local read "First frame\ndelay (ms)"() -> (w2804:dbl)
        n1376 = call <vilib>:"DAQmx Stop Task.vi"("task/channels in"=w2814, "error in"=w2810) -> ("task out"=w2802:refnum<k21>, "error out"=w2801:errorcluster)  [unwired: 12 in]
        n1377 = call <vilib>:"DAQmx Stop Task.vi"("task/channels in"=w2813, "error in"=w2811) -> ("task out"=w2799:refnum<k21>, "error out"=w2798:errorcluster)  [unwired: 12 in]
        n1378 = local read "Duty Cycle camera"() -> (w2800:dbl)
        n1379 = local read "Frame rate"() -> (w2761:dbl)
        n1380 = Divide(x=w2804, y=1000) -> (x/y=w2771:dbl)
        n1381 = property class="DAQmx Channel"(reference=w2802, error in=w2801, "CO.Pulse.Freq"=w2761, "CO.Pulse.DutyCyc"=w2800) -> (reference out=w2790:refnum<k21>, error out=w2788:errorcluster)
        n1382 = Multiply(x=w2761, y=w2771) -> (x*y=w2806:dbl)
        n1383 = To Long Integer(number=w2806) -> (32bit integer=w2785:i32)
        n1384 = Reciprocal(x=w2761) -> (1/x=w2805:dbl)
        n1385 = local read "Illuminated Frames"() -> (w2757:i32)
        n1386 = Multiply(x=w2785, y=w2805) -> (x*y=w2791:dbl)
        n1387 = local read "Finishing frames"() -> (w2786:i32)
        n1388 = property on="Initial calculated\ndelay (frames)" class="DigNum (strict)"("Value"=w2806) -> ()  [unwired: 2 in, 2 out]
        n1389 = Multiply(x=w2791, y=1000) -> (x*y=w2797:dbl)
        n1390 = property on="Laser delay (ms)" class="DigNum (strict)"("Value"=w2797) -> ()  [unwired: 2 in, 2 out]
        n1391 = Add(x=w2757, y=w2785) -> (x+y=w2774:i32)
        n1392 = Add(x=w2786, y=w2774) -> (x+y=w2766:i32)
        n1393 = Divide(x=w2757, y=2) -> (x/y=w2775:dbl)
        n1394 = To Long Integer(number=w2775) -> (32bit integer=w2759:i32)
        n1395 = case shown="False" w2765 {
          tunnel: [w2822 w2842] -> w2762
          tunnel: [w2815 1] -> w2758
          tunnel: [w2820 w2843] -> w2760
          tunnel: [w2823 0.0] -> w2763
          tunnel: w2761 -> [w2818 w2840]
          tunnel: w2764 -> [w2819 _]
          tunnel: w2759 -> [w2817 _]
          tunnel: w2757 -> [w2816 w2839]
          frame False {
            n1396 = property on="Pulsed" class="Bool (strict)"() -> ("Value"=w2821:bool)  [unwired: 2 in, 2 out]
            n1397 = property on="Duty Cycle 1\npreset" class="Knob (strict)"() -> ("Value"=w2820:dbl)  [unwired: 2 in, 2 out]
            n1398 = case shown="False" w2821 {
              tunnel: w2820 -> [_ _]
              tunnel: [w2828 0.0] -> w2823
              tunnel: [w2827 w2837] -> w2822
              tunnel: w2819 -> [w2826 _]
              tunnel: w2818 -> [w2825 w2837]
              tunnel: w2817 -> [w2824 _]
              tunnel: w2816 -> [_ w2836]
              tunnel: [w2824 w2836] -> w2815
              frame False {
                n1399 = property on="Link rates" class="Bool (strict)"() -> ("Value"=w2831:bool)  [unwired: 2 in, 2 out]
                n1400 = case shown="True" w2831 {
                  tunnel: [w2832 w2834] -> w2827
                  tunnel: w2826 -> [w2832 _]
                  tunnel: w2825 -> [_ w2833]
                  frame False {
                  }
                  frame True {
                    n1401 = Divide(x=w2833, y=2) -> (x/y=w2834:dbl)
                    n1402 = property on="Frequency 1" class="Knob (strict)"("Value"=w2834) -> ()  [unwired: 2 in, 2 out]
                  }
                }
                n1403 = Multiply(x=w2827, y=2) -> (x*y=w2830:dbl)
                n1404 = Reciprocal(x=w2830) -> (1/x=w2828:dbl)
              }
              frame True {
              }
            }
            n1405 = property on="Duty Cycle 1" class="Knob (strict)"("Value"=w2820) -> ()  [unwired: 2 in, 2 out]
          }
          frame True {
            w2843 = 0.9999 ("x")
            n1406 = Reciprocal(x=w2840) -> (1/x=w2846:dbl)
            n1407 = Multiply(x=w2846, y=w2839) -> (x*y=w2844:dbl)
            n1408 = property on="Duty Cycle 1" class="Knob (strict)"("Value"=w2843) -> ()  [unwired: 2 in, 2 out]
            n1409 = Divide(x=w2843, y=w2844) -> (x/y=w2842:dbl)
            n1410 = property on="Frequency 1" class="Knob (strict)"("Value"=w2842) -> ()  [unwired: 2 in, 2 out]
          }
        }
        n1411 = Add(x=w2791, y=w2763) -> (x+y=w2792:dbl)
        n1412 = Multiply(x=w2763, y=1000) -> (x*y=w2793:dbl)
        n1413 = property class="DAQmx Channel"(reference=w2799, error in=w2798, "CO.Pulse.Freq"=w2762, "CO.Pulse.DutyCyc"=w2760, "CO.Pulse.Freq.InitialDelay"=w2791) -> (reference out=w2780:refnum<k21>, error out=w2778:errorcluster)
        n1414 = property class="DAQmx Channel"(reference=w2796, error in=w2795, "CO.Pulse.Freq"=w2762, "CO.Pulse.DutyCyc"=w2760, "CO.Pulse.Freq.InitialDelay"=w2792) -> (reference out=w2784:refnum<k21>, error out=w2782:errorcluster)
        n1415 = property on="Initial delay\n473 nm (ms)" class="DigNum (strict)"("Value"=w2793) -> ()  [unwired: 2 in, 2 out]
        n1416 = property on="delay\ncompensation" class="DigNum (strict)"() -> ("Value"=w2756:dbl)  [unwired: 2 in, 2 out]
        n1417 = Subtract(x=w2771, y=w2756) -> (x-y=w2772:dbl)
        n1418 = Multiply(x=w2761, y=w2772) -> (x*y=w2773:dbl)
        n1419 = property class="DAQmx Timing"(reference=w2790, error in=w2788, "SampQuant.SampPerChan"=w2766) -> (reference out=w2789:refnum<k21>, error out=w2787:errorcluster)
        n1420 = Multiply(x=w2756, y=w2761) -> (x*y=w2767:dbl)
        n1421 = To Long Integer(number=w2773) -> (32bit integer=w2770:i32)
        n1422 = To Long Integer(number=w2767) -> (32bit integer=w2768:i32)
        n1423 = property on="Initial frames" class="DigNum (strict)"("Value"=w2770) -> ()  [unwired: 2 in, 2 out]
        n1424 = Subtract(x=w2766, y=w2768) -> (x-y=w2769:i32)
        n1425 = property on="Frames to acquire" class="DigNum (strict)"("Value"=w2769) -> ()  [unwired: 2 in, 2 out]
        n1426 = property class="DAQmx Timing"(reference=w2780, error in=w2778, "SampQuant.SampPerChan"=w2758) -> (reference out=w2779:refnum<k21>, error out=w2777:errorcluster)
        n1427 = property on="Laser pulses" class="DigNum (strict)"("Value"=w2758) -> ()  [unwired: 2 in, 2 out]
        n1428 = property on="Trigger pulses" class="DigNum (strict)"("Value"=w2766) -> ()  [unwired: 2 in, 2 out]
        n1429 = property class="DAQmx Timing"(reference=w2784, error in=w2782, "SampQuant.SampPerChan"=w2758) -> (reference out=w2783:refnum<k21>, error out=w2781:errorcluster)
        n1430 = Merge Errors(w2787, w2777, w2781) -> (w2812:errorcluster)
      }
      event "ALL LASERS": Value Change {
        n1431 = event-data() -> ()  [unwired: 1 in, 1 out]
        n1432 = call <vilib>:"DAQmx Stop Task.vi"("task/channels in"=w2857, "error in"=w2855) -> ("task out"=w2856:refnum<k21>, "error out"=w2854:errorcluster)  [unwired: 12 in]
        n1433 = call <vilib>:"DAQmx Stop Task.vi"("task/channels in"=w2861, "error in"=w2859) -> ("task out"=w2860:refnum<k21>, "error out"=w2858:errorcluster)  [unwired: 12 in]
        n1434 = call <vilib>:"DAQmx Stop Task.vi"("task/channels in"=w2853, "error in"=w2852) -> ("task out"=w2851:refnum<k21>, "error out"=w2850:errorcluster)  [unwired: 12 in]
        n1435 = property on="561 nm" class="Bool (strict)"(error in=w2854, "Value"="ALL LASERS") -> (error out=w2849:errorcluster)  [unwired: 1 in, 1 out]
        n1436 = property on="473 nm" class="Bool (strict)"(error in=w2858, "Value"="ALL LASERS") -> (error out=w2848:errorcluster)  [unwired: 1 in, 1 out]
        n1437 = case shown="True" "manual laser control" {
          tunnel: "ALL LASERS" -> [_ w2880]
          tunnel: [w2869 w2879] -> w2866
          tunnel: [w2871 w2878] -> w2865
          tunnel: [w2870 w2877] -> w2864
          tunnel: [w2868 w2876] -> w2863
          tunnel: w2860 -> [w2868 w2875]
          tunnel: w2856 -> [w2869 w2874]
          tunnel: w2849 -> [w2871 w2873]
          tunnel: w2848 -> [w2870 w2872]
          frame False {
          }
          frame True {
            n1438 = case shown="True" w2880 {
              tunnel: w2873 -> [w2882 w2892]
              tunnel: w2872 -> [w2881 w2891]
              tunnel: w2874 -> [w2890 w2900]
              tunnel: w2875 -> [w2887 w2897]
              tunnel: [w2886 w2896] -> w2879
              tunnel: [w2885 w2895] -> w2878
              tunnel: [w2884 w2894] -> w2876
              tunnel: [w2883 w2893] -> w2877
              frame True {
                w2888 = 10192 items=["High"=10192, "Low"=10214] ("CO.Pulse.IdleState")
                w2889 = 10192 items=["High"=10192, "Low"=10214] ("CO.Pulse.IdleState")
                n1439 = property class="DAQmx Channel"(reference=w2887, error in=w2881, "CO.Pulse.IdleState"=w2888) -> (reference out=w2884:refnum<k21>, error out=w2883:errorcluster)
                n1440 = property class="DAQmx Channel"(reference=w2890, error in=w2882, "CO.Pulse.IdleState"=w2889) -> (reference out=w2886:refnum<k21>, error out=w2885:errorcluster)
              }
              frame False {
                w2898 = 10214 items=["High"=10192, "Low"=10214] ("CO.Pulse.IdleState")
                w2899 = 10214 items=["High"=10192, "Low"=10214] ("CO.Pulse.IdleState")
                n1441 = property class="DAQmx Channel"(reference=w2897, error in=w2891, "CO.Pulse.IdleState"=w2898) -> (reference out=w2894:refnum<k21>, error out=w2893:errorcluster)
                n1442 = property class="DAQmx Channel"(reference=w2900, error in=w2892, "CO.Pulse.IdleState"=w2899) -> (reference out=w2896:refnum<k21>, error out=w2895:errorcluster)
              }
            }
          }
        }
        n1443 = Merge Errors(w2850, w2865, w2864) -> (w2862:errorcluster)
      }
      event "ALL LASERS 2": Value Change {
        n1444 = event-data() -> ()  [unwired: 1 in, 1 out]
        n1445 = call <vilib>:"DAQmx Stop Task.vi"("task/channels in"=w2914, "error in"=w2912) -> ("task out"=w2913:refnum<k21>, "error out"=w2911:errorcluster)  [unwired: 12 in]
        n1446 = call <vilib>:"DAQmx Stop Task.vi"("task/channels in"=w2918, "error in"=w2916) -> ("task out"=w2917:refnum<k21>, "error out"=w2915:errorcluster)  [unwired: 12 in]
        n1447 = call <vilib>:"DAQmx Stop Task.vi"("task/channels in"=w2910, "error in"=w2909) -> ("task out"=w2908:refnum<k21>, "error out"=w2907:errorcluster)  [unwired: 12 in]
        n1448 = property on="AFLEX" class="Bool (strict)"() -> ("Value"=w2901:bool)  [unwired: 2 in, 2 out]
        n1449 = case shown="False" w2901 {
          tunnel: w2917 -> [w2936 w2963]
          tunnel: w2915 -> [w2935 w2967]
          tunnel: w2913 -> [w2934 w2964]
          tunnel: w2911 -> [w2933 w2968]
          tunnel: "ALL LASERS 2" -> [w2932 w2969]
          tunnel: [w2929 w2965] -> w2905
          tunnel: [w2928 w2964] -> w2904
          tunnel: [w2925 w2966] -> w2903
          tunnel: [w2924 w2963] -> w2902
          frame False {
            n1450 = case shown="False" w2932 {
              selector: w2932 -> [w2948 w2961]
              tunnel: w2933 -> [w2949 w2962]
              tunnel: w2935 -> [w2947 w2960]
              tunnel: w2934 -> [w2946 w2959]
              tunnel: w2936 -> [w2942 w2955]
              tunnel: [w2940 w2953] -> w2931
              tunnel: [w2939 w2952] -> w2930
              tunnel: [w2938 w2951] -> w2927
              tunnel: [w2937 w2950] -> w2926
              frame True {
                w2943 = 10192 items=["High"=10192, "Low"=10214] ("CO.Pulse.IdleState")
                w2944 = 10192 items=["High"=10192, "Low"=10214] ("CO.Pulse.IdleState")
                n1451 = property on="561 nm 2" class="Bool (strict)"(error in=w2949, "Value"=w2948) -> (error out=w2945:errorcluster)  [unwired: 1 in, 1 out]
                n1452 = property on="473 nm 2" class="Bool (strict)"(error in=w2947, "Value"=w2948) -> (error out=w2941:errorcluster)  [unwired: 1 in, 1 out]
                n1453 = property class="DAQmx Channel"(reference=w2942, error in=w2941, "CO.Pulse.IdleState"=w2943) -> (reference out=w2938:refnum<k21>, error out=w2937:errorcluster)
                n1454 = property class="DAQmx Channel"(reference=w2946, error in=w2945, "CO.Pulse.IdleState"=w2944) -> (reference out=w2940:refnum<k21>, error out=w2939:errorcluster)
              }
              frame False {
                w2956 = 10214 items=["High"=10192, "Low"=10214] ("CO.Pulse.IdleState")
                w2957 = 10214 items=["High"=10192, "Low"=10214] ("CO.Pulse.IdleState")
                n1455 = property on="561 nm 2" class="Bool (strict)"(error in=w2962, "Value"=w2961) -> (error out=w2958:errorcluster)  [unwired: 1 in, 1 out]
                n1456 = property on="473 nm 2" class="Bool (strict)"(error in=w2960, "Value"=w2961) -> (error out=w2954:errorcluster)  [unwired: 1 in, 1 out]
                n1457 = property class="DAQmx Channel"(reference=w2955, error in=w2954, "CO.Pulse.IdleState"=w2956) -> (reference out=w2951:refnum<k21>, error out=w2950:errorcluster)
                n1458 = property class="DAQmx Channel"(reference=w2959, error in=w2958, "CO.Pulse.IdleState"=w2957) -> (reference out=w2953:refnum<k21>, error out=w2952:errorcluster)
              }
            }
            n1459 = call <vilib>:"DAQmx Start Task.vi"("task/channels in"=w2931, "error in"=w2930) -> ("task out"=w2922:refnum<k21>, "error out"=w2923:errorcluster)  [unwired: 12 in]
            n1460 = call <vilib>:"DAQmx Start Task.vi"("task/channels in"=w2927, "error in"=w2926) -> ("task out"=w2920:refnum<k21>, "error out"=w2921:errorcluster)  [unwired: 12 in]
            n1461 = call <vilib>:"DAQmx Stop Task.vi"("task/channels in"=w2922, "error in"=w2923) -> ("task out"=w2928:refnum<k21>, "error out"=w2929:errorcluster)  [unwired: 12 in]
            n1462 = call <vilib>:"DAQmx Stop Task.vi"("task/channels in"=w2920, "error in"=w2921) -> ("task out"=w2924:refnum<k21>, "error out"=w2925:errorcluster)  [unwired: 12 in]
          }
          frame True {
            n1463 = property on="561 nm 2" class="Bool (strict)"(error in=w2968, "Value"=w2969) -> (error out=w2965:errorcluster)  [unwired: 1 in, 1 out]
            n1464 = property on="473 nm 2" class="Bool (strict)"(error in=w2967, "Value"=w2969) -> (error out=w2966:errorcluster)  [unwired: 1 in, 1 out]
          }
        }
        n1465 = Merge Errors(w2907, w2905, w2903) -> (w2919:errorcluster)
      }
      event "ALL OFF": Value Change {
        w2982 = FALSE
        w2986 = 10214 items=["High"=10192, "Low"=10214] ("CO.Pulse.IdleState")
        w2987 = 10214 items=["High"=10192, "Low"=10214] ("CO.Pulse.IdleState")
        n1466 = event-data() -> ()  [unwired: 1 in, 1 out]
        n1467 = call <vilib>:"DAQmx Stop Task.vi"("task/channels in"=w2996, "error in"=w2994) -> ("task out"=w2995:refnum<k21>, "error out"=w2993:errorcluster)  [unwired: 12 in]
        n1468 = call <vilib>:"DAQmx Stop Task.vi"("task/channels in"=w3000, "error in"=w2998) -> ("task out"=w2999:refnum<k21>, "error out"=w2997:errorcluster)  [unwired: 12 in]
        n1469 = call <vilib>:"DAQmx Stop Task.vi"("task/channels in"=w2992, "error in"=w2991) -> ("task out"=w2990:refnum<k21>, "error out"=w2989:errorcluster)  [unwired: 12 in]
        n1470 = property on="561 nm" class="Bool (strict)"(error in=w2993, "Value"=w2982) -> (error out=w2988:errorcluster)  [unwired: 1 in, 1 out]
        n1471 = property on="473 nm" class="Bool (strict)"(error in=w2997, "Value"=w2982) -> (error out=w2985:errorcluster)  [unwired: 1 in, 1 out]
        n1472 = property class="DAQmx Channel"(reference=w2999, error in=w2985, "CO.Pulse.IdleState"=w2986) -> (reference out=w2973:refnum<k21>, error out=w2971:errorcluster)
        n1473 = property class="DAQmx Channel"(reference=w2995, error in=w2988, "CO.Pulse.IdleState"=w2987) -> (reference out=w2975:refnum<k21>, error out=w2977:errorcluster)
        n1474 = call <vilib>:"DAQmx Start Task.vi"("task/channels in"=w2973, "error in"=w2971) -> ("task out"=w2978:refnum<k21>, "error out"=w2979:errorcluster)  [unwired: 12 in]
        n1475 = call <vilib>:"DAQmx Start Task.vi"("task/channels in"=w2975, "error in"=w2977) -> ("task out"=w2980:refnum<k21>, "error out"=w2981:errorcluster)  [unwired: 12 in]
        n1476 = call <vilib>:"DAQmx Stop Task.vi"("task/channels in"=w2978, "error in"=w2979) -> ("task out"=w2972:refnum<k21>, "error out"=w2970:errorcluster)  [unwired: 12 in]
        n1477 = call <vilib>:"DAQmx Stop Task.vi"("task/channels in"=w2980, "error in"=w2981) -> ("task out"=w2974:refnum<k21>, "error out"=w2976:errorcluster)  [unwired: 12 in]
        n1478 = Merge Errors(w2976, w2970) -> (w2984:errorcluster)
        n1479 = property on="ALL LASERS" class="Bool (strict)"(error in=w2984, "Value"=w2982) -> (error out=w2983:errorcluster)  [unwired: 1 in, 1 out]
        n1480 = Merge Errors(w2989, w2983) -> (w3001:errorcluster)
      }
      event "ALL OFF 2": Value Change {
        w3014 = FALSE
        w3018 = 10214 items=["High"=10192, "Low"=10214] ("CO.Pulse.IdleState")
        w3019 = 10214 items=["High"=10192, "Low"=10214] ("CO.Pulse.IdleState")
        n1481 = event-data() -> ()  [unwired: 1 in, 1 out]
        n1482 = call <vilib>:"DAQmx Stop Task.vi"("task/channels in"=w3028, "error in"=w3026) -> ("task out"=w3027:refnum<k21>, "error out"=w3025:errorcluster)  [unwired: 12 in]
        n1483 = call <vilib>:"DAQmx Stop Task.vi"("task/channels in"=w3032, "error in"=w3030) -> ("task out"=w3031:refnum<k21>, "error out"=w3029:errorcluster)  [unwired: 12 in]
        n1484 = call <vilib>:"DAQmx Stop Task.vi"("task/channels in"=w3024, "error in"=w3023) -> ("task out"=w3022:refnum<k21>, "error out"=w3021:errorcluster)  [unwired: 12 in]
        n1485 = property on="473 nm 2" class="Bool (strict)"(error in=w3029, "Value"=w3014) -> (error out=w3017:errorcluster)  [unwired: 1 in, 1 out]
        n1486 = property on="561 nm 2" class="Bool (strict)"(error in=w3025, "Value"=w3014) -> (error out=w3020:errorcluster)  [unwired: 1 in, 1 out]
        n1487 = property class="DAQmx Channel"(reference=w3031, error in=w3017, "CO.Pulse.IdleState"=w3018) -> (reference out=w3005:refnum<k21>, error out=w3003:errorcluster)
        n1488 = property class="DAQmx Channel"(reference=w3027, error in=w3020, "CO.Pulse.IdleState"=w3019) -> (reference out=w3009:refnum<k21>, error out=w3006:errorcluster)
        n1489 = call <vilib>:"DAQmx Start Task.vi"("task/channels in"=w3005, "error in"=w3003) -> ("task out"=w3010:refnum<k21>, "error out"=w3011:errorcluster)  [unwired: 12 in]
        n1490 = call <vilib>:"DAQmx Start Task.vi"("task/channels in"=w3009, "error in"=w3006) -> ("task out"=w3012:refnum<k21>, "error out"=w3013:errorcluster)  [unwired: 12 in]
        n1491 = call <vilib>:"DAQmx Stop Task.vi"("task/channels in"=w3010, "error in"=w3011) -> ("task out"=w3004:refnum<k21>, "error out"=w3002:errorcluster)  [unwired: 12 in]
        n1492 = call <vilib>:"DAQmx Stop Task.vi"("task/channels in"=w3012, "error in"=w3013) -> ("task out"=w3008:refnum<k21>, "error out"=w3007:errorcluster)  [unwired: 12 in]
        n1493 = Merge Errors(w3007, w3002) -> (w3016:errorcluster)
        n1494 = property on="ALL LASERS 2" class="Bool (strict)"(error in=w3016, "Value"=w3014) -> (error out=w3015:errorcluster)  [unwired: 1 in, 1 out]
        n1495 = Merge Errors(w3021, w3015) -> (w3033:errorcluster)
      }
      event "manual laser control": Value Change {
        w3046 = FALSE
        w3050 = 10214 items=["High"=10192, "Low"=10214] ("CO.Pulse.IdleState")
        w3051 = 10214 items=["High"=10192, "Low"=10214] ("CO.Pulse.IdleState")
        n1496 = event-data() -> ()  [unwired: 1 in, 1 out]
        n1497 = call <vilib>:"DAQmx Stop Task.vi"("task/channels in"=w3056, "error in"=w3055) -> ("task out"=w3054:refnum<k21>, "error out"=w3053:errorcluster)  [unwired: 12 in]
        n1498 = call <vilib>:"DAQmx Stop Task.vi"("task/channels in"=w3060, "error in"=w3058) -> ("task out"=w3059:refnum<k21>, "error out"=w3057:errorcluster)  [unwired: 12 in]
        n1499 = call <vilib>:"DAQmx Stop Task.vi"("task/channels in"=w3064, "error in"=w3062) -> ("task out"=w3063:refnum<k21>, "error out"=w3061:errorcluster)  [unwired: 12 in]
        n1500 = property on="473 nm" class="Bool (strict)"(error in=w3061, "Value"=w3046) -> (error out=w3049:errorcluster)  [unwired: 1 in, 1 out]
        n1501 = property on="561 nm" class="Bool (strict)"(error in=w3057, "Value"=w3046) -> (error out=w3052:errorcluster)  [unwired: 1 in, 1 out]
        n1502 = property class="DAQmx Channel"(reference=w3063, error in=w3049, "CO.Pulse.IdleState"=w3050) -> (reference out=w3037:refnum<k21>, error out=w3035:errorcluster)
        n1503 = property class="DAQmx Channel"(reference=w3059, error in=w3052, "CO.Pulse.IdleState"=w3051) -> (reference out=w3041:refnum<k21>, error out=w3038:errorcluster)
        n1504 = call <vilib>:"DAQmx Start Task.vi"("task/channels in"=w3037, "error in"=w3035) -> ("task out"=w3042:refnum<k21>, "error out"=w3043:errorcluster)  [unwired: 12 in]
        n1505 = call <vilib>:"DAQmx Start Task.vi"("task/channels in"=w3041, "error in"=w3038) -> ("task out"=w3044:refnum<k21>, "error out"=w3045:errorcluster)  [unwired: 12 in]
        n1506 = call <vilib>:"DAQmx Stop Task.vi"("task/channels in"=w3042, "error in"=w3043) -> ("task out"=w3036:refnum<k21>, "error out"=w3034:errorcluster)  [unwired: 12 in]
        n1507 = call <vilib>:"DAQmx Stop Task.vi"("task/channels in"=w3044, "error in"=w3045) -> ("task out"=w3040:refnum<k21>, "error out"=w3039:errorcluster)  [unwired: 12 in]
        n1508 = Merge Errors(w3039, w3034) -> (w3048:errorcluster)
        n1509 = property on="ALL LASERS" class="Bool (strict)"(error in=w3048, "Value"=w3046) -> (error out=w3047:errorcluster)  [unwired: 1 in, 1 out]
        n1510 = Merge Errors(w3053, w3047) -> (w3065:errorcluster)
      }
      event "561 nm": Value Change {
        n1511 = event-data() -> ()  [unwired: 1 in, 1 out]
        n1512 = call <vilib>:"DAQmx Stop Task.vi"("task/channels in"=w3078, "error in"=w3076) -> ("task out"=w3077:refnum<k21>, "error out"=w3075:errorcluster)  [unwired: 12 in]
        n1513 = call <vilib>:"DAQmx Stop Task.vi"("task/channels in"=w3074, "error in"=w3072) -> ("task out"=w3073:refnum<k21>, "error out"=w3071:errorcluster)  [unwired: 12 in]
        n1514 = call <vilib>:"DAQmx Stop Task.vi"("task/channels in"=w3070, "error in"=w3069) -> ("task out"=w3068:refnum<k21>, "error out"=w3067:errorcluster)  [unwired: 12 in]
        n1515 = property on="manual laser control" class="Bool (strict)"() -> ("Value"=w3066:bool)  [unwired: 2 in, 2 out]
        n1516 = case shown="True" "561 nm" {
          selector: "561 nm" -> [_ w3102]
          tunnel: w3075 -> [w3091 w3107]
          tunnel: w3071 -> [w3087 w3103]
          tunnel: w3077 -> [w3092 w3108]
          tunnel: w3073 -> [w3088 w3104]
          tunnel: [w3090 w3106] -> w3083
          tunnel: [w3089 w3105] -> w3080
          tunnel: [w3088 w3104] -> w3082
          tunnel: [w3087 w3103] -> w3079
          tunnel: w3066 -> [w3085 w3101]
          frame True {
            n1517 = property on="473 nm" class="Bool (strict)"() -> ("Value"=w3086:bool)  [unwired: 2 in, 2 out]
            n1518 = case shown="True" w3085 {
              tunnel: w3092 -> [w3094 w3099]
              tunnel: w3091 -> [w3093 w3097]
              tunnel: [w3094 w3096] -> w3090
              tunnel: [w3093 w3095] -> w3089
              frame False {
              }
              frame True {
                w3098 = 10192 items=["High"=10192, "Low"=10214] ("CO.Pulse.IdleState")
                n1519 = property class="DAQmx Channel"(reference=w3099, error in=w3097, "CO.Pulse.IdleState"=w3098) -> (reference out=w3096:refnum<k21>, error out=w3095:errorcluster)
              }
            }
            n1520 = case shown="True" w3086 {
              selector: w3086 -> [_ w3100]
              frame False {
              }
              frame True {
                n1521 = property on="ALL LASERS" class="Bool (strict)"("Value"=w3100) -> ()  [unwired: 2 in, 2 out]
              }
            }
          }
          frame False {
            n1522 = property on="ALL LASERS" class="Bool (strict)"("Value"=w3102) -> ()  [unwired: 2 in, 2 out]
            n1523 = case shown="False" w3101 {
              tunnel: w3108 -> [w3110 w3115]
              tunnel: w3107 -> [w3109 w3113]
              tunnel: [w3110 w3112] -> w3106
              tunnel: [w3109 w3111] -> w3105
              frame False {
              }
              frame True {
                w3114 = 10214 items=["High"=10192, "Low"=10214] ("CO.Pulse.IdleState")
                n1524 = property class="DAQmx Channel"(reference=w3115, error in=w3113, "CO.Pulse.IdleState"=w3114) -> (reference out=w3112:refnum<k21>, error out=w3111:errorcluster)
              }
            }
          }
        }
        n1525 = Merge Errors(w3067, w3080, w3079) -> (w3081:errorcluster)
      }
      event "561 nm 2": Value Change {
        n1526 = event-data() -> ()  [unwired: 1 in, 1 out]
        n1527 = property on="AFLEX" class="Bool (strict)"() -> ("Value"=w3116:bool)  [unwired: 2 in, 2 out]
        n1528 = call <vilib>:"DAQmx Stop Task.vi"("task/channels in"=w3133, "error in"=w3131) -> ("task out"=w3132:refnum<k21>, "error out"=w3130:errorcluster)  [unwired: 12 in]
        n1529 = call <vilib>:"DAQmx Stop Task.vi"("task/channels in"=w3129, "error in"=w3127) -> ("task out"=w3128:refnum<k21>, "error out"=w3126:errorcluster)  [unwired: 12 in]
        n1530 = call <vilib>:"DAQmx Stop Task.vi"("task/channels in"=w3125, "error in"=w3124) -> ("task out"=w3123:refnum<k21>, "error out"=w3122:errorcluster)  [unwired: 12 in]
        n1531 = case shown="True" w3116 {
          tunnel: w3132 -> [w3143 w3171]
          tunnel: w3130 -> [w3142 w3170]
          tunnel: w3128 -> [w3141 w3169]
          tunnel: w3126 -> [w3140 w3168]
          tunnel: "561 nm 2" -> [w3139 w3167]
          tunnel: [w3137 w3161] -> w3120
          tunnel: [w3138 w3159] -> w3119
          tunnel: [w3136 w3156] -> w3118
          tunnel: [w3135 w3155] -> w3117
          frame True {
            n1532 = case shown="False" w3139 {
              selector: w3139 -> [_ w3152]
              tunnel: w3142 -> [w3144 w3151]
              tunnel: w3140 -> [w3147 w3153]
              tunnel: w3143 -> [w3145 w3150]
              tunnel: w3141 -> [w3148 w3154]
              tunnel: [w3145 w3150] -> w3138
              tunnel: [w3148 w3154] -> w3136
              tunnel: [w3147 w3153] -> w3135
              tunnel: [w3144 w3151] -> w3137
              frame True {
                n1533 = property on="473 nm 2" class="Bool (strict)"() -> ("Value"=w3146:bool)  [unwired: 2 in, 2 out]
                n1534 = case shown="True" w3146 {
                  selector: w3146 -> [_ w3149]
                  frame False {
                  }
                  frame True {
                    n1535 = property on="ALL LASERS 2" class="Bool (strict)"("Value"=w3149) -> ()  [unwired: 2 in, 2 out]
                  }
                }
              }
              frame False {
                n1536 = property on="ALL LASERS 2" class="Bool (strict)"("Value"=w3152) -> ()  [unwired: 2 in, 2 out]
              }
            }
          }
          frame False {
            n1537 = case shown="True" w3167 {
              selector: w3167 -> [_ w3181]
              tunnel: w3170 -> [w3177 w3186]
              tunnel: w3168 -> [w3173 w3182]
              tunnel: w3171 -> [w3179 w3188]
              tunnel: w3169 -> [w3174 w3183]
              tunnel: [w3176 w3185] -> w3160
              tunnel: [w3175 w3184] -> w3162
              tunnel: [w3174 w3183] -> w3157
              tunnel: [w3173 w3182] -> w3158
              frame True {
                w3178 = 10192 items=["High"=10192, "Low"=10214] ("CO.Pulse.IdleState")
                n1538 = property on="473 nm 2" class="Bool (strict)"() -> ("Value"=w3172:bool)  [unwired: 2 in, 2 out]
                n1539 = case shown="True" w3172 {
                  selector: w3172 -> [_ w3180]
                  frame False {
                  }
                  frame True {
                    n1540 = property on="ALL LASERS 2" class="Bool (strict)"("Value"=w3180) -> ()  [unwired: 2 in, 2 out]
                  }
                }
                n1541 = property class="DAQmx Channel"(reference=w3179, error in=w3177, "CO.Pulse.IdleState"=w3178) -> (reference out=w3176:refnum<k21>, error out=w3175:errorcluster)
              }
              frame False {
                w3187 = 10214 items=["High"=10192, "Low"=10214] ("CO.Pulse.IdleState")
                n1542 = property on="ALL LASERS 2" class="Bool (strict)"("Value"=w3181) -> ()  [unwired: 2 in, 2 out]
                n1543 = property class="DAQmx Channel"(reference=w3188, error in=w3186, "CO.Pulse.IdleState"=w3187) -> (reference out=w3185:refnum<k21>, error out=w3184:errorcluster)
              }
            }
            n1544 = call <vilib>:"DAQmx Start Task.vi"("task/channels in"=w3160, "error in"=w3162) -> ("task out"=w3165:refnum<k21>, "error out"=w3166:errorcluster)  [unwired: 12 in]
            n1545 = call <vilib>:"DAQmx Start Task.vi"("task/channels in"=w3157, "error in"=w3158) -> ("task out"=w3163:refnum<k21>, "error out"=w3164:errorcluster)  [unwired: 12 in]
            n1546 = call <vilib>:"DAQmx Stop Task.vi"("task/channels in"=w3165, "error in"=w3166) -> ("task out"=w3159:refnum<k21>, "error out"=w3161:errorcluster)  [unwired: 12 in]
            n1547 = call <vilib>:"DAQmx Stop Task.vi"("task/channels in"=w3163, "error in"=w3164) -> ("task out"=w3156:refnum<k21>, "error out"=w3155:errorcluster)  [unwired: 12 in]
          }
        }
        n1548 = Merge Errors(w3122, w3120, w3117) -> (w3134:errorcluster)
      }
      event "473 nm": Value Change {
        n1549 = event-data() -> ()  [unwired: 1 in, 1 out]
        n1550 = call <vilib>:"DAQmx Stop Task.vi"("task/channels in"=w3199, "error in"=w3201) -> ("task out"=w3198:refnum<k21>, "error out"=w3200:errorcluster)  [unwired: 12 in]
        n1551 = call <vilib>:"DAQmx Stop Task.vi"("task/channels in"=w3192, "error in"=w3193) -> ("task out"=w3191:refnum<k21>, "error out"=w3190:errorcluster)  [unwired: 12 in]
        n1552 = call <vilib>:"DAQmx Stop Task.vi"("task/channels in"=w3197, "error in"=w3195) -> ("task out"=w3196:refnum<k21>, "error out"=w3194:errorcluster)  [unwired: 12 in]
        n1553 = property on="manual laser control" class="Bool (strict)"() -> ("Value"=w3189:bool)  [unwired: 2 in, 2 out]
        n1554 = case shown="False" "473 nm" {
          selector: "473 nm" -> [_ w3225]
          tunnel: w3200 -> [w3210 w3226]
          tunnel: w3194 -> [w3214 w3230]
          tunnel: w3198 -> [w3211 w3227]
          tunnel: w3196 -> [w3215 w3231]
          tunnel: [w3213 w3229] -> w3206
          tunnel: [w3212 w3228] -> w3203
          tunnel: [w3211 w3227] -> w3205
          tunnel: [w3210 w3226] -> w3204
          tunnel: w3189 -> [w3208 w3224]
          frame True {
            n1555 = property on="561 nm" class="Bool (strict)"() -> ("Value"=w3209:bool)  [unwired: 2 in, 2 out]
            n1556 = case shown="True" w3208 {
              tunnel: w3215 -> [w3217 w3221]
              tunnel: w3214 -> [w3216 w3220]
              tunnel: [w3217 w3219] -> w3213
              tunnel: [w3216 w3218] -> w3212
              frame False {
              }
              frame True {
                w3222 = 10192 items=["High"=10192, "Low"=10214] ("CO.Pulse.IdleState")
                n1557 = property class="DAQmx Channel"(reference=w3221, error in=w3220, "CO.Pulse.IdleState"=w3222) -> (reference out=w3219:refnum<k21>, error out=w3218:errorcluster)
              }
            }
            n1558 = case shown="True" w3209 {
              selector: w3209 -> [_ w3223]
              frame False {
              }
              frame True {
                n1559 = property on="ALL LASERS" class="Bool (strict)"("Value"=w3223) -> ()  [unwired: 2 in, 2 out]
              }
            }
          }
          frame False {
            n1560 = property on="ALL LASERS" class="Bool (strict)"("Value"=w3225) -> ()  [unwired: 2 in, 2 out]
            n1561 = case shown="False" w3224 {
              tunnel: w3231 -> [w3233 w3237]
              tunnel: w3230 -> [w3232 w3236]
              tunnel: [w3233 w3235] -> w3229
              tunnel: [w3232 w3234] -> w3228
              frame False {
              }
              frame True {
                w3238 = 10214 items=["High"=10192, "Low"=10214] ("CO.Pulse.IdleState")
                n1562 = property class="DAQmx Channel"(reference=w3237, error in=w3236, "CO.Pulse.IdleState"=w3238) -> (reference out=w3235:refnum<k21>, error out=w3234:errorcluster)
              }
            }
          }
        }
        n1563 = Merge Errors(w3190, w3204, w3203) -> (w3202:errorcluster)
      }
      event "473 nm 2": Value Change {
        n1564 = event-data() -> ()  [unwired: 1 in, 1 out]
        n1565 = call <vilib>:"DAQmx Stop Task.vi"("task/channels in"=w3254, "error in"=w3256) -> ("task out"=w3253:refnum<k21>, "error out"=w3255:errorcluster)  [unwired: 12 in]
        n1566 = call <vilib>:"DAQmx Stop Task.vi"("task/channels in"=w3247, "error in"=w3248) -> ("task out"=w3246:refnum<k21>, "error out"=w3245:errorcluster)  [unwired: 12 in]
        n1567 = property on="AFLEX" class="Bool (strict)"() -> ("Value"=w3239:bool)  [unwired: 2 in, 2 out]
        n1568 = call <vilib>:"DAQmx Stop Task.vi"("task/channels in"=w3252, "error in"=w3250) -> ("task out"=w3251:refnum<k21>, "error out"=w3249:errorcluster)  [unwired: 12 in]
        n1569 = case shown="True" w3239 {
          tunnel: w3255 -> [w3266 w3294]
          tunnel: w3253 -> [w3265 w3293]
          tunnel: w3251 -> [w3264 w3292]
          tunnel: w3249 -> [w3263 w3291]
          tunnel: "473 nm 2" -> [w3262 w3290]
          tunnel: [w3261 w3283] -> w3243
          tunnel: [w3260 w3282] -> w3242
          tunnel: [w3259 w3280] -> w3241
          tunnel: [w3258 w3278] -> w3240
          frame True {
            n1570 = case shown="False" w3262 {
              selector: w3262 -> [_ w3275]
              tunnel: w3266 -> [w3270 w3276]
              tunnel: w3263 -> [w3268 w3274]
              tunnel: w3265 -> [w3271 w3277]
              tunnel: w3264 -> [w3267 w3273]
              tunnel: [w3267 w3273] -> w3259
              tunnel: [w3271 w3277] -> w3261
              tunnel: [w3270 w3276] -> w3260
              tunnel: [w3268 w3274] -> w3258
              frame True {
                n1571 = property on="561 nm 2" class="Bool (strict)"() -> ("Value"=w3269:bool)  [unwired: 2 in, 2 out]
                n1572 = case shown="True" w3269 {
                  selector: w3269 -> [_ w3272]
                  frame False {
                  }
                  frame True {
                    n1573 = property on="ALL LASERS 2" class="Bool (strict)"("Value"=w3272) -> ()  [unwired: 2 in, 2 out]
                  }
                }
              }
              frame False {
                n1574 = property on="ALL LASERS 2" class="Bool (strict)"("Value"=w3275) -> ()  [unwired: 2 in, 2 out]
              }
            }
          }
          frame False {
            n1575 = case shown="True" w3290 {
              selector: w3290 -> [_ w3304]
              tunnel: w3294 -> [w3296 w3305]
              tunnel: w3291 -> [w3300 w3309]
              tunnel: w3293 -> [w3297 w3306]
              tunnel: w3292 -> [w3301 w3310]
              tunnel: [w3299 w3308] -> w3281
              tunnel: [w3298 w3307] -> w3279
              tunnel: [w3297 w3306] -> w3285
              tunnel: [w3296 w3305] -> w3284
              frame True {
                w3302 = 10192 items=["High"=10192, "Low"=10214] ("CO.Pulse.IdleState")
                n1576 = property on="561 nm 2" class="Bool (strict)"() -> ("Value"=w3295:bool)  [unwired: 2 in, 2 out]
                n1577 = case shown="True" w3295 {
                  selector: w3295 -> [_ w3303]
                  frame False {
                  }
                  frame True {
                    n1578 = property on="ALL LASERS 2" class="Bool (strict)"("Value"=w3303) -> ()  [unwired: 2 in, 2 out]
                  }
                }
                n1579 = property class="DAQmx Channel"(reference=w3301, error in=w3300, "CO.Pulse.IdleState"=w3302) -> (reference out=w3299:refnum<k21>, error out=w3298:errorcluster)
              }
              frame False {
                w3311 = 10214 items=["High"=10192, "Low"=10214] ("CO.Pulse.IdleState")
                n1580 = property on="ALL LASERS 2" class="Bool (strict)"("Value"=w3304) -> ()  [unwired: 2 in, 2 out]
                n1581 = property class="DAQmx Channel"(reference=w3310, error in=w3309, "CO.Pulse.IdleState"=w3311) -> (reference out=w3308:refnum<k21>, error out=w3307:errorcluster)
              }
            }
            n1582 = call <vilib>:"DAQmx Start Task.vi"("task/channels in"=w3285, "error in"=w3284) -> ("task out"=w3288:refnum<k21>, "error out"=w3289:errorcluster)  [unwired: 12 in]
            n1583 = call <vilib>:"DAQmx Start Task.vi"("task/channels in"=w3281, "error in"=w3279) -> ("task out"=w3286:refnum<k21>, "error out"=w3287:errorcluster)  [unwired: 12 in]
            n1584 = call <vilib>:"DAQmx Stop Task.vi"("task/channels in"=w3288, "error in"=w3289) -> ("task out"=w3283:refnum<k21>, "error out"=w3282:errorcluster)  [unwired: 12 in]
            n1585 = call <vilib>:"DAQmx Stop Task.vi"("task/channels in"=w3286, "error in"=w3287) -> ("task out"=w3280:refnum<k21>, "error out"=w3278:errorcluster)  [unwired: 12 in]
          }
        }
        n1586 = Merge Errors(w3245, w3242, w3240) -> (w3257:errorcluster)
      }
      event "EPI 2": Value Change {
        n1587 = event-data() -> ()  [unwired: 1 in, 1 out]
        n1588 = call <vilib>:"DAQmx Stop Task.vi"("task/channels in"=w3327, "error in"=w3325) -> ("task out"=w3326:refnum<k21>, "error out"=w3321:errorcluster)  [unwired: 12 in]
        n1589 = call <vilib>:"DAQmx Stop Task.vi"("task/channels in"=w3324, "error in"=w3322) -> ("task out"=w3323:refnum<k21>, "error out"=w3317:errorcluster)  [unwired: 12 in]
        n1590 = call <vilib>:"DAQmx Stop Task.vi"("task/channels in"=w3318, "error in"=w3319) -> ("task out"=w3316:refnum<k21>, "error out"=w3315:errorcluster)  [unwired: 12 in]
        n1591 = property on="EPI 3" class="Bool (strict)"(error in=w3314, "Value"="EPI 2") -> (error out=w3313:errorcluster)  [unwired: 1 in, 1 out]
        n1592 = case shown="True" "Link shutters 2" {
          tunnel: w3335 -> [w3341 w3354]
          tunnel: w3313 -> [w3340 w3353]
          tunnel: w3334 -> [w3337 w3352]
          tunnel: w3333 -> [w3336 w3351]
          tunnel: [w3336 w3344] -> w3329
          tunnel: [w3337 w3349] -> w3330
          tunnel: [w3339 w3348] -> w3332
          tunnel: [w3338 w3347] -> w3331
          tunnel: "EPI 2" -> [w3342 w3346]
          frame False {
            n1593 = call-poly <vilib>:"DAQmx Write.vi"("task/channels in"=w3341, "data"=w3342, "error in"=w3340) -> ("task out"=w3339:refnum<k21>, "error out"=w3338:errorcluster)  [unwired: 10 in, 1 out]
          }
          frame True {
            n1594 = Not(x=w3346) -> (.not. x?=w3343:bool)
            n1595 = call-poly <vilib>:"DAQmx Write.vi"("task/channels in"=w3354, "data"=w3346, "error in"=w3353) -> ("task out"=w3348:refnum<k21>, "error out"=w3347:errorcluster)  [unwired: 10 in, 1 out]
            n1596 = call-poly <vilib>:"DAQmx Write.vi"("task/channels in"=w3352, "data"=w3343, "error in"=w3351) -> ("task out"=w3349:refnum<k21>, "error out"=w3350:errorcluster)  [unwired: 10 in, 1 out]
            n1597 = property on="FRAP 2" class="Bool (strict)"(error in=w3350, "Value"=w3343) -> (error out=w3345:errorcluster)  [unwired: 1 in, 1 out]
            n1598 = property on="FRAP 3" class="Bool (strict)"(error in=w3345, "Value"=w3343) -> (error out=w3344:errorcluster)  [unwired: 1 in, 1 out]
          }
        }
        n1599 = Merge Errors(w3321, w3317, w3315) -> (w3320:errorcluster)
      }
      event "FRAP 2": Value Change {
        n1600 = event-data() -> ()  [unwired: 1 in, 1 out]
        n1601 = property on="FRAP 3" class="Bool (strict)"(error in=w3357, "Value"="FRAP 2") -> (error out=w3356:errorcluster)  [unwired: 1 in, 1 out]
        n1602 = property on="Link shutters 2" class="Bool (strict)"() -> ("Value"=w3378:bool)  [unwired: 2 in, 2 out]
        n1603 = call <vilib>:"DAQmx Stop Task.vi"("task/channels in"=w3366, "error in"=w3365) -> ("task out"=w3364:refnum<k21>, "error out"=w3361:errorcluster)  [unwired: 12 in]
        n1604 = call <vilib>:"DAQmx Stop Task.vi"("task/channels in"=w3368, "error in"=w3367) -> ("task out"=w3363:refnum<k21>, "error out"=w3359:errorcluster)  [unwired: 12 in]
        n1605 = call <vilib>:"DAQmx Stop Task.vi"("task/channels in"=w3370, "error in"=w3369) -> ("task out"=w3362:refnum<k21>, "error out"=w3358:errorcluster)  [unwired: 12 in]
        n1606 = case shown="True" w3378 {
          tunnel: w3377 -> [w3380 w3395]
          tunnel: w3376 -> [w3381 w3389]
          tunnel: w3375 -> [w3384 w3396]
          tunnel: w3356 -> [w3383 w3390]
          tunnel: [w3382 w3391] -> w3371
          tunnel: [w3379 w3394] -> w3372
          tunnel: [w3380 w3393] -> w3374
          tunnel: [w3381 w3392] -> w3373
          tunnel: "FRAP 2" -> [w3385 w3397]
          frame False {
            n1607 = call-poly <vilib>:"DAQmx Write.vi"("task/channels in"=w3384, "data"=w3385, "error in"=w3383) -> ("task out"=w3379:refnum<k21>, "error out"=w3382:errorcluster)  [unwired: 10 in, 1 out]
          }
          frame True {
            n1608 = Not(x=w3397) -> (.not. x?=w3386:bool)
            n1609 = call-poly <vilib>:"DAQmx Write.vi"("task/channels in"=w3396, "data"=w3397, "error in"=w3390) -> ("task out"=w3394:refnum<k21>, "error out"=w3391:errorcluster)  [unwired: 10 in, 1 out]
            n1610 = call-poly <vilib>:"DAQmx Write.vi"("task/channels in"=w3395, "data"=w3386, "error in"=w3389) -> ("task out"=w3393:refnum<k21>, "error out"=w3388:errorcluster)  [unwired: 10 in, 1 out]
            n1611 = property on="EPI 3" class="Bool (strict)"(error in=w3388, "Value"=w3386) -> (error out=w3387:errorcluster)  [unwired: 1 in, 1 out]
            n1612 = property on="EPI 2" class="Bool (strict)"(error in=w3387, "Value"=w3386) -> (error out=w3392:errorcluster)  [unwired: 1 in, 1 out]
          }
        }
        n1613 = Merge Errors(w3361, w3359, w3358) -> (w3360:errorcluster)
      }
      event "Manual pump ctrl": Value Change {
        n1614 = event-data() -> ()  [unwired: 1 in, 1 out]
        n1615 = call <vilib>:"DAQmx Stop Task.vi"("task/channels in"=w3416, "error in"=w3415) -> ("task out"=w3414:refnum<k21>, "error out"=w3411:errorcluster)  [unwired: 12 in]
        n1616 = call <vilib>:"DAQmx Stop Task.vi"("task/channels in"=w3418, "error in"=w3417) -> ("task out"=w3413:refnum<k21>, "error out"=w3409:errorcluster)  [unwired: 12 in]
        n1617 = call <vilib>:"DAQmx Stop Task.vi"("task/channels in"=w3420, "error in"=w3419) -> ("task out"=w3412:refnum<k21>, "error out"=w3408:errorcluster)  [unwired: 12 in]
        n1618 = case shown="True" "Manual pump ctrl" {
          tunnel: [w3421 w3426] -> w3400
          tunnel: w3402 -> [_ _]
          tunnel: w3401 -> [w3421 w3432]
          tunnel: "Pump ID" -> [_ w3422]
          tunnel: "Syringe size" -> [_ w3436]
          frame False {
          }
          frame True {
            n1619 = property on="Inited pump port" class="VISAName"(error in=w3432) -> (error out=w3425:errorcluster, "Value"=w3423:refnum<visa-resource-name>)  [unwired: 1 in, 1 out]
            n1620 = call-by-ref "SPM100 control noinit v3.2.vi"("error in"=w3425, "Syringe size"=w3436, "Pump No."=w3422, "Visa resource"=w3423) -> ("error out"=w3424:errorcluster, "dV"=w3429:dbl, "VISA resource name out"=w3433:refnum<visa-resource-name>)  [unwired: 3 in, 2 out]
            "dV" <- w3429
            n1621 = property on="Manual pump ctrl" class="Bool (strict)"(error in=w3424, "Value"=FALSE ("Manual pump ctrl")) -> (error out=w3434:errorcluster)  [unwired: 1 in, 1 out]
            n1622 = property on="Inited pump port" class="VISAName"(error in=w3434, "Value"=w3433) -> (error out=w3428:errorcluster)  [unwired: 1 in, 1 out]
            n1623 = property on="Deliverable volume (ml)" class="DigNum (strict)"(error in=w3428) -> (error out=w3427:errorcluster, "Value"=w3431:dbl)  [unwired: 1 in, 1 out]
            n1624 = Add(x=w3431, y=w3429) -> (x+y=w3430:dbl)
            n1625 = property on="Deliverable volume (ml)" class="DigNum (strict)"(error in=w3427, "Value"=w3430) -> (error out=w3426:errorcluster)  [unwired: 1 in, 1 out]
          }
        }
        n1626 = Merge Errors(w3411, w3409, w3408) -> (w3410:errorcluster)
      }
      event "Enable pump control": Value Change {
        n1627 = event-data() -> ()  [unwired: 1 in, 1 out]
        n1628 = call <vilib>:"DAQmx Stop Task.vi"("task/channels in"=w3457, "error in"=w3456) -> ("task out"=w3455:refnum<k21>, "error out"=w3452:errorcluster)  [unwired: 12 in]
        n1629 = call <vilib>:"DAQmx Stop Task.vi"("task/channels in"=w3459, "error in"=w3458) -> ("task out"=w3454:refnum<k21>, "error out"=w3450:errorcluster)  [unwired: 12 in]
        n1630 = call <vilib>:"DAQmx Stop Task.vi"("task/channels in"=w3461, "error in"=w3460) -> ("task out"=w3453:refnum<k21>, "error out"=w3449:errorcluster)  [unwired: 12 in]
        n1631 = case shown="False" "Enable pump control" {
          tunnel: [w3462 w3465] -> w3442
          tunnel: w3443 -> [w3462 w3465]
          tunnel: [T2."Disabled and Grayed Out" ("Disabled") T2."Enabled" ("Disabled")] -> w3441
          frame False {
          }
          frame True {
          }
        }
        n1632 = property on="Pump start" class="Bool (strict)"(error in=w3442, "DisabledEnum"=w3441, "Value"=FALSE ("Pump start")) -> (error out=w3437:errorcluster)  [unwired: 1 in, 1 out]
        n1633 = property on="Shot no." class="DigNum (strict)"(error in=w3437, "Value"=1 ("Shot no.")) -> (error out=w3438:errorcluster)  [unwired: 1 in, 1 out]
        n1634 = Merge Errors(w3452, w3450, w3449) -> (w3451:errorcluster)
      }
      event "Pump start": Value Change {
        (unwired) T2."Disabled and Grayed Out" ("Disabled")
        n1635 = event-data() -> ()  [unwired: 1 in, 1 out]
        n1636 = call <vilib>:"DAQmx Stop Task.vi"("task/channels in"=w3488, "error in"=w3487) -> ("task out"=w3486:refnum<k21>, "error out"=w3483:errorcluster)  [unwired: 12 in]
        n1637 = call <vilib>:"DAQmx Stop Task.vi"("task/channels in"=w3490, "error in"=w3489) -> ("task out"=w3485:refnum<k21>, "error out"=w3481:errorcluster)  [unwired: 12 in]
        n1638 = call <vilib>:"DAQmx Stop Task.vi"("task/channels in"=w3492, "error in"=w3491) -> ("task out"=w3484:refnum<k21>, "error out"=w3480:errorcluster)  [unwired: 12 in]
        n1639 = property on="Pump start" class="Bool (strict)"(error in=w3471) -> (error out=w3470:errorcluster, "Value"=w3469:bool)  [unwired: 1 in, 1 out]
        n1640 = property on="Pump running" class="Bool (strict)"() -> ("Value"=w3466:bool)  [unwired: 2 in, 2 out]
        n1641 = Not(x=w3469) -> (.not. x?=w3468:bool)
        n1642 = And(x=w3468, y=w3466) -> (x .and. y?=w3467:bool)
        n1643 = case shown="True" w3467 {
          tunnel: w3470 -> [_ w3509]
          frame False {
          }
          frame True {
            n1644 = property on="modal pump reference" class="VIRef (strict)"(error in=w3509) -> (error out=w3508:errorcluster, "Value"=w3507:refnum<vi>)  [unwired: 1 in, 1 out]
            n1645 = call-by-ref "Wait On Asynchronous Call"(reference=w3507, error in=w3508) -> (reference out=w3495:refnum<vi>, error out=w3506:errorcluster, "VISA resource name out"=w3505:refnum<visa-resource-name>, "Closing"=w3504:bool, "dV"=w3499:dbl)  [unwired: 12 in, 1 out]
            n1646 = property on="Inited pump port" class="VISAName"(error in=w3506, "Value"=w3505) -> (error out=w3498:errorcluster)  [unwired: 1 in, 1 out]
            n1647 = property on="Closing" class="Bool (strict)"(error in=w3498, "Value"=w3504) -> (error out=w3497:errorcluster)  [unwired: 1 in, 1 out]
            n1648 = property on="Deliverable volume (ml)" class="DigNum (strict)"(error in=w3497) -> (error out=w3501:errorcluster, "Value"=w3502:dbl)  [unwired: 1 in, 1 out]
            n1649 = Add(x=w3502, y=w3499) -> (x+y=w3503:dbl)
            n1650 = property on="dV" class="DigNum (strict)"(error in=w3501, "Value"=w3499) -> (error out=w3500:errorcluster)  [unwired: 1 in, 1 out]
            n1651 = property on="Deliverable volume (ml)" class="DigNum (strict)"(error in=w3500, "Value"=w3503) -> (error out=w3494:errorcluster)  [unwired: 1 in, 1 out]
            n1652 = Close Reference(reference=w3495, error in (no error)=w3494) -> (error out=w3493:errorcluster)
            n1653 = property on="Pump running" class="Bool (strict)"(error in=w3493, "Value"=FALSE ("Pump running")) -> ()  [unwired: 1 in, 2 out]
          }
        }
        n1654 = property on="Shot no." class="DigNum (strict)"(error in=w3471, "Value"=1 ("Shot no.")) -> (error out=w3474:errorcluster)  [unwired: 1 in, 1 out]
        n1655 = property on="Closing" class="Bool (strict)"(error in=w3474, "Value"=FALSE ("Closing")) -> (error out=w3473:errorcluster)  [unwired: 1 in, 1 out]
        n1656 = Merge Errors(w3483, w3481, w3480) -> (w3482:errorcluster)
      }
    }
    n1657 = Not(x=w251) -> (.not. x?=w250:bool)
    n1658 = Compound Arithmetic op=AND("Pump start", w253, w250) -> (w255:bool)
    n1659 = case shown="False" w284 {
      tunnel: [w364 w428] -> w305
      tunnel: [w363 w426] -> w291
      tunnel: w256 -> [w355 w426]
      tunnel: [w362 w429] -> w303
      tunnel: [w361 w426] -> w292
      tunnel: w300 -> [w360 w428]
      tunnel: w299 -> [w356 w429]
      tunnel: [w359 w427] -> w297
      tunnel: w295 -> [w357 w427]
      tunnel: [w358 w426] -> w290
      frame False {
        # "Trigger"
        n1660 = property on="Tab Control" class="TabCtl (strict)"() -> ("Value"=w354:T1)  [unwired: 2 in, 2 out]
        n1661 = case shown="\"Finite sequences\", Default" w354 {
          tunnel: [w379 w398] -> w364
          tunnel: [w378 w397] -> w363
          tunnel: w360 -> [w377 w399]
          tunnel: [w376 w395] -> w359
          tunnel: [w375 w393] -> w358
          tunnel: w357 -> [w374 w396]
          tunnel: w355 -> [w368 w394]
          frame "Finite sequences", Default {
            n1662 = property on="manual laser control" class="Bool (strict)"(error in=w368) -> (error out=w369:errorcluster, "Value"=w365:bool)  [unwired: 1 in, 1 out]
            n1663 = property on="561 nm" class="Bool (strict)"(error in=w368) -> (error out=w372:errorcluster, "Value"=w367:bool)  [unwired: 1 in, 1 out]
            n1664 = property on="473 nm" class="Bool (strict)"(error in=w369) -> (error out=w373:errorcluster, "Value"=w371:bool)  [unwired: 1 in, 1 out]
            n1665 = Or(x=w367, y=w365) -> (x .or. y?=w366:bool)
            n1666 = Or(x=w371, y=w365) -> (x .or. y?=w370:bool)
            n1667 = case shown="True" w370 {
              tunnel: [w381 w385] -> w376
              tunnel: [w380 w384] -> w375
              tunnel: w374 -> [w381 w383]
              tunnel: w373 -> [w380 w382]
              frame False {
              }
              frame True {
                # "473 nm"
                n1668 = call <vilib>:"DAQmx Start Task.vi"("task/channels in"=w383, "error in"=w382) -> ("task out"=w385:refnum<k21>, "error out"=w384:errorcluster)  [unwired: 12 in]
              }
            }
            n1669 = case shown="True" w366 {
              tunnel: [w387 w391] -> w379
              tunnel: [w386 w390] -> w378
              tunnel: w377 -> [w387 w389]
              tunnel: w372 -> [w386 w388]
              frame False {
              }
              frame True {
                # "561 nm"
                n1670 = call <vilib>:"DAQmx Start Task.vi"("task/channels in"=w389, "error in"=w388) -> ("task out"=w391:refnum<k21>, "error out"=w390:errorcluster)  [unwired: 12 in]
              }
            }
          }
          frame "Continous camera triggering" {
            n1671 = property on="AFLEX" class="Bool (strict)"() -> ("Value"=w392:bool)  [unwired: 2 in, 2 out]
            n1672 = case shown="True" w392 {
              tunnel: w399 -> [w402 w413]
              tunnel: [w402 w412] -> w398
              tunnel: [w401 w411] -> w397
              tunnel: w396 -> [w400 w410]
              tunnel: [w400 w409] -> w395
              tunnel: w394 -> [w401 w405]
              tunnel: [w401 w408] -> w393
              frame False {
              }
              frame True {
                n1673 = property on="561 nm 2" class="Bool (strict)"(error in=w405) -> (error out=w407:errorcluster, "Value"=w406:bool)  [unwired: 1 in, 1 out]
                n1674 = property on="473 nm 2" class="Bool (strict)"(error in=w405) -> (error out=w404:errorcluster, "Value"=w403:bool)  [unwired: 1 in, 1 out]
                n1675 = case shown="True" w406 {
                  tunnel: w413 -> [w421 w425]
                  tunnel: [w421 w424] -> w412
                  tunnel: [w420 w423] -> w411
                  tunnel: w407 -> [w420 w422]
                  frame False {
                  }
                  frame True {
                    # "561 nm"
                    n1676 = call <vilib>:"DAQmx Start Task.vi"("task/channels in"=w425, "error in"=w422) -> ("task out"=w424:refnum<k21>, "error out"=w423:errorcluster)  [unwired: 12 in]
                  }
                }
                n1677 = case shown="True" w403 {
                  tunnel: w410 -> [w415 w419]
                  tunnel: [w415 w418] -> w409
                  tunnel: [w414 w417] -> w408
                  tunnel: w404 -> [w414 w416]
                  frame False {
                  }
                  frame True {
                    # "473 nm"
                    n1678 = call <vilib>:"DAQmx Start Task.vi"("task/channels in"=w419, "error in"=w416) -> ("task out"=w418:refnum<k21>, "error out"=w417:errorcluster)  [unwired: 12 in]
                  }
                }
              }
            }
          }
        }
        n1679 = call <vilib>:"DAQmx Start Task.vi"("task/channels in"=w356, "error in"=w355) -> ("task out"=w362:refnum<k21>, "error out"=w361:errorcluster)  [unwired: 12 in]
      }
      frame True {
      }
    }
    n1680 = case shown="True" w255 {
      tunnel: w257 -> [_ w308]
      tunnel: w252 -> [w307 w318]
      tunnel: [w307 w311] -> w248
      frame False {
      }
      frame True {
        n1681 = property on="Shot no." class="DigNum (strict)"() -> ("Value"=w309:i32)  [unwired: 2 in, 2 out]
        n1682 = property on="Shots before pump start" class="DigNum (strict)"() -> ("Value"=w321:i32)  [unwired: 2 in, 2 out]
        n1683 = Decrement(x=w309) -> (x-1=w310:i32)
        n1684 = Equal?(x=w310, y=w321) -> (x = y?=w320:bool)
        n1685 = case shown="True" w320 {
          tunnel: [w324 0.0 ("dV")] -> w314
          tunnel: w309 -> [w326 _]
          tunnel: w308 -> [_ w338]
          frame False {
            (unwired) 1 ("y")
            n1686 = property on="Shots to acquire" class="DigNum (strict)"() -> (error out=w322:errorcluster, "Value"=w323:i32)  [unwired: 2 in, 1 out]
            n1687 = Equal?(x=w326, y=w323) -> (x = y?=w325:bool)
            n1688 = case shown="True" w325 {
              tunnel: w322 -> [_ w332]
              tunnel: [0.0 ("dV") w335] -> w324
              frame False {
              }
              frame True {
                n1689 = property on="modal pump reference" class="VIRef (strict)"(error in=w332) -> (error out=w331:errorcluster, "Value"=w333:refnum<vi>)  [unwired: 1 in, 1 out]
                n1690 = call-by-ref "Wait On Asynchronous Call"(reference=w333, error in=w331) -> (reference out=w334:refnum<vi>, error out=w330:errorcluster, "VISA resource name out"=w337:refnum<visa-resource-name>, "Closing"=→"Closing":bool, "dV"=w335:dbl)  [unwired: 12 in, 1 out]
                n1691 = property on="Inited pump port" class="VISAName"("Value"=w337) -> ()  [unwired: 2 in, 2 out]
                n1692 = Close Reference(reference=w334, error in (no error)=w330) -> (error out=w328:errorcluster)
                n1693 = property on="Pump running" class="Bool (strict)"(error in=w328, "Value"=FALSE ("Exit pump ctrl")) -> ()  [unwired: 1 in, 2 out]
              }
            }
          }
          frame True {
            n1694 = Open VI Reference(type specifier VI Refnum (for type only)=refnum<vi> refnum, vi path="vi path", options=256) -> (vi reference=w342:refnum<vi>, error out=w341:errorcluster)  [unwired: 3 in]
            n1695 = property on="Pump ID" class="DigNum (strict)"() -> ("Value"=w349:i32)  [unwired: 2 in, 2 out]
            n1696 = property on="Syringe size" class="Ring (strict)"() -> ("Value"=w347:dbl)  [unwired: 2 in, 2 out]
            n1697 = call-by-ref "Start Asynchronous Call"(reference=w342, error in=w341, "VISA resource in"=w338, "Time to run (sec.)"="Running time (s)", "Max volume"="Deliverable volume (ml)", "Pump No."=w349, "Syringe size"=w347, "Infuse/\nWithdraw"=TRUE ("Infuse/\nWithdraw"), "Flow rate"="Flow rate", "FlowRateUnit"="FlowRateUnit") -> (reference out=→"modal pump reference":refnum<vi>)  [unwired: 4 in, 5 out]
            "Pump running" <- TRUE ("Exit pump ctrl")
          }
        }
        n1698 = property on="In Done\nstate" class="Bool (strict)"(error in=w318, "Value"=FALSE ("In Done\nstate")) -> (error out=w315:errorcluster)  [unwired: 1 in, 1 out]
        n1699 = property on="Deliverable volume (ml)" class="DigNum (strict)"(error in=w315) -> (error out=w313:errorcluster, "Value"=w316:dbl)  [unwired: 1 in, 1 out]
        n1700 = Add(x=w316, y=w314) -> (x+y=w317:dbl)
        n1701 = property on="dV" class="DigNum (strict)"(error in=w313, "Value"=w314) -> (error out=w312:errorcluster)  [unwired: 1 in, 1 out]
        n1702 = property on="Deliverable volume (ml)" class="DigNum (strict)"(error in=w312, "Value"=w317) -> (error out=w311:errorcluster)  [unwired: 1 in, 1 out]
      }
    }
    n1703 = property on="Loops" class="DigNum (strict)"() -> ("Value"=w294:i32)  [unwired: 2 in, 2 out]
    n1704 = Increment(x=w294) -> (x+1=→"Loops":i32)
    n1705 = Unbundle By Name(w292) -> ("status"=w288:bool)
    n1706 = Unbundle By Name(w291) -> ("status"=w289:bool)
    n1707 = Unbundle By Name(w290) -> ("status"=w287:bool)
    n1708 = Or(x=w288, y=w289) -> (x .or. y?=w286:bool)
    n1709 = Or(x=w286, y=w287) -> (x .or. y?=w285:bool)
    n1710 = Or(x=w285, y=w284) -> (x .or. y?=w306:bool)
    n1711 = property on="In Done\nstate" class="Bool (strict)"(error in=w248, "Value"=FALSE ("In Done\nstate")) -> ()  [unwired: 1 in, 2 out]
  }
  n1712 = call <vilib>:"DAQmx Stop Task.vi"("task/channels in"=w23, "error in"=w22) -> ("task out"=w21:refnum<k21>, "error out"=w20:errorcluster)  [unwired: 12 in]
  n1713 = call-poly <vilib>:"DAQmx Write.vi"("task/channels in"=w99, "data"=w100, "error in"=w98) -> ("task out"=w105:refnum<k21>, "error out"=w104:errorcluster)  [unwired: 10 in, 1 out]
  n1714 = call-poly <vilib>:"DAQmx Write.vi"("task/channels in"=w97, "data"=w100, "error in"=w57) -> ("task out"=w107:refnum<k21>, "error out"=w106:errorcluster)  [unwired: 10 in, 1 out]
  n1715 = call <vilib>:"DAQmx Clear Task.vi"("task in"=w21, "error in"=w20) -> ("error out"=w19:errorcluster)  [unwired: 13 in]
  n1716 = call <vilib>:"DAQmx Stop Task.vi"("task/channels in"=w105, "error in"=w104) -> ("task out"=w110:refnum<k21>, "error out"=w103:errorcluster)  [unwired: 12 in]
  n1717 = call <vilib>:"DAQmx Stop Task.vi"("task/channels in"=w107, "error in"=w106) -> ("task out"=w109:refnum<k21>, "error out"=w108:errorcluster)  [unwired: 12 in]
  n1718 = property on="Inited pump port" class="VISAName"(error in=w2) -> (error out=w1:errorcluster, "Value"=w3:refnum<visa-resource-name>)  [unwired: 1 in, 1 out]
  n1719 = property on="Power control" class="Bool (strict)"() -> ("Value"=w52:bool)  [unwired: 2 in, 2 out]
  n1720 = case shown="True" w52 {
    tunnel: w59 -> [_ w3520]
    tunnel: [w3511 w3518] -> w58
    tunnel: w51 -> [w3511 w3514]
    tunnel: [w3510 w3516] -> w54
    tunnel: w53 -> [_ w3515]
    tunnel: w50 -> [w3510 w3512]
    frame False {
    }
    frame True {
      n1721 = call <vilib>:"DAQmx Stop Task.vi"("task/channels in"=w3520, "error in"=w3514) -> ("task out"=w3519:refnum<k21>, "error out"=w3521:errorcluster)  [unwired: 12 in]
      n1722 = call <vilib>:"DAQmx Stop Task.vi"("task/channels in"=w3515, "error in"=w3512) -> ("task out"=w3513:refnum<k21>, "error out"=w3517:errorcluster)  [unwired: 12 in]
      n1723 = call <vilib>:"DAQmx Clear Task.vi"("task in"=w3519, "error in"=w3521) -> ("error out"=w3518:errorcluster)  [unwired: 13 in]
      n1724 = call <vilib>:"DAQmx Clear Task.vi"("task in"=w3513, "error in"=w3517) -> ("error out"=w3516:errorcluster)  [unwired: 13 in]
    }
  }
  n1725 = call <vilib>:"DAQmx Clear Task.vi"("task in"=w142, "error in"=w144) -> ("error out"=w143:errorcluster)  [unwired: 13 in]
  n1726 = call <vilib>:"DAQmx Clear Task.vi"("task in"=w176, "error in"=w175) -> ("error out"=w177:errorcluster)  [unwired: 13 in]
  n1727 = call <vilib>:"DAQmx Clear Task.vi"("task in"=w139, "error in"=w140) -> ("error out"=w141:errorcluster)  [unwired: 13 in]
  n1728 = call <vilib>:"DAQmx Clear Task.vi"("task in"=w110, "error in"=w103) -> ("error out"=w102:errorcluster)  [unwired: 13 in]
  n1729 = call <vilib>:"DAQmx Clear Task.vi"("task in"=w109, "error in"=w108) -> ("error out"=w101:errorcluster)  [unwired: 13 in]
  n1730 = VISA Close(VISA resource name=w3, error in (no error)=w1) -> (error out=w11:errorcluster)
  n1731 = Merge Errors(w19, w177, w143, w141, w102, w101, w58, w54, w11) -> (w136:errorcluster)
  n1732 = property on="ALL LASERS" class="Bool (strict)"(error in=w136, "Value"=w45) -> (error out=w138:errorcluster)  [unwired: 1 in, 1 out]
  n1733 = property on="561 nm" class="Bool (strict)"(error in=w138, "Value"=w45) -> (error out=w137:errorcluster)  [unwired: 1 in, 1 out]
  n1734 = property on="473 nm" class="Bool (strict)"(error in=w137, "Value"=w45) -> (error out=w123:errorcluster)  [unwired: 1 in, 1 out]
  n1735 = property on="manual laser control" class="Bool (strict)"(error in=w123, "Value"=w45) -> (error out=w46:errorcluster)  [unwired: 1 in, 1 out]
  n1736 = property on="Continous ill" class="Bool (strict)"(error in=w46, "Value"=w45) -> (error out=w119:errorcluster)  [unwired: 1 in, 1 out]
  n1737 = property on="HALF DC" class="Bool (strict)"(error in=w119, "Value"=w45, "DisabledEnum"=w74) -> (error out=w96:errorcluster)  [unwired: 1 in, 1 out]
  n1738 = property on="EPI" class="Bool (strict)"(error in=w96, "Value"=w45) -> (error out=w48:errorcluster)  [unwired: 1 in, 1 out]
  n1739 = property on="EPI 2" class="Bool (strict)"(error in=w48, "Value"=w45) -> (error out=w49:errorcluster)  [unwired: 1 in, 1 out]
  n1740 = property on="FRAP 2" class="Bool (strict)"(error in=w49, "Value"=w45) -> (error out=w47:errorcluster)  [unwired: 1 in, 1 out]
  n1741 = property on="FRAP" class="Bool (strict)"(error in=w47, "Value"=w45) -> (error out=w76:errorcluster)  [unwired: 1 in, 1 out]
  n1742 = property on="Link rates" class="Bool (strict)"(error in=w76, "Value"=TRUE ("Link rates"), "DisabledEnum"=w74) -> (error out=w75:errorcluster)  [unwired: 1 in, 1 out]
  n1743 = property on="Link shutters" class="Bool (strict)"(error in=w75, "Value"=w7, "DisabledEnum"=w74) -> (error out=w80:errorcluster)  [unwired: 1 in, 1 out]
  n1744 = property on="Pulsed" class="Bool (strict)"(error in=w80, "Value"=w7) -> (error out=w78:errorcluster)  [unwired: 1 in, 1 out]
  n1745 = property on="Frequency 1" class="Knob (strict)"(error in=w78, "DisabledEnum"=w74) -> (error out=w77:errorcluster)  [unwired: 1 in, 1 out]
  n1746 = property on="Duty Cycle 1\npreset" class="Knob (strict)"(error in=w77) -> (error out=w121:errorcluster, "Value"=w120:dbl)  [unwired: 1 in, 1 out]
  n1747 = property on="Duty Cycle 1" class="Knob (strict)"(error in=w121, "Value"=w120, "DisabledEnum"=w74, "Scale.Maximum"=0.5 ("Scale.Range:Maximum")) -> (error out=w10:errorcluster)  [unwired: 1 in, 1 out]
  n1748 = flat-sequence {
    tunnel: [w3523] -> w89
    tunnel: w4 -> [w3523]
    frame #0 {
      n1749 = Wait Until Next ms Multiple(millisecond multiple=u32 500) -> ()  [unwired: 1 out]
    }
  }
  n1750 = property on="Pump start" class="Bool (strict)"(error in=w10, "Value"=w7, "DisabledEnum"=T2."Disabled and Grayed Out" ("Disabled")) -> (error out=w8:errorcluster)  [unwired: 1 in, 1 out]
  n1751 = property on="Enable pump control" class="Bool (strict)"(error in=w8, "Value"=w7) -> (error out=w5:errorcluster)  [unwired: 1 in, 1 out]
  n1752 = property on="EPI 3" class="Bool (strict)"(error in=w5, "Value"=w7) -> (error out=w6:errorcluster)  [unwired: 1 in, 1 out]
  n1753 = property on="FRAP 3" class="Bool (strict)"(error in=w6, "Value"=w7) -> (error out=w4:errorcluster)  [unwired: 1 in, 1 out]
  n1754 = property on="stop" class="Bool (strict)"(error in=w89, "Value"=FALSE ("Stop pressed")) -> (error out=w130:errorcluster)  [unwired: 1 in, 1 out]
  n1755 = call <vilib>:"General Error Handler.vi"("type of dialog (OK msg:1)"=w195, "error in (no error)"=w130) -> ("error out"=→"error out":errorcluster)  [unwired: 9 in, 4 out]
  "Duty Cycle 1\npreset" <- "Duty Cycle 1"
  "Full Power \nFrames" <- "Illuminated Frames"
  "Duty Cycle 1\nfull DC" <- "Duty Cycle 1"
